vi "FP_Tracker.vi"() -> ()   [LabVIEW 2018, in "Tracker.lvlib"]
uses:
  Tracker.lvlib
  SubVi's/Controls/CTL_IO_status_indicator.ctl
  SubVi's/Controls/CTL_Zones_control_and_indicator.ctl
  SubVi's/Controls/CTL_Zone_indicator.ctl
  SubVi's/Controls/CTL_All_References.ctl
  SubVi's/Controls/CTL_Controls_References.ctl
  SubVi's/Controls/CTL_Indicators_References.ctl
  SubVi's/Controls/CTL_Panes_and_VIs_References.ctl
  SubVi's/Controls/CTL_Cage_radial_segmentation.ctl
  SubVi's/Controls/CTL_Image_Geometrical_and_scaling_parameters.ctl
  <vilib>/ProgressBar/Progress Bar Dialog.lvclass
  SubVi's/Controls/CTL_Calibration_parameters.ctl
  SubVi's/Controls/CTL_Dispenser_calibration_info.ctl
  SubVi's/Controls/CTL_Pre-filter_params.ctl
  SubVi's/Controls/CTL_Mouse_Draw_Params.ctl
  SubVi's/Controls/CTL_IO_params_cluster.ctl
  SubVi's/Controls/CTL_Overlays_cluster.ctl
  SubVi's/Controls/CTL_Animal_Coordinates_and_Speed.ctl
  SubVi's/Controls/CTL_Settings_cluster.ctl
  SubVi's/Controls/CTL_Histogram_parameters.ctl
  SubVi's/Controls/CTL_Filter_selector.ctl
  SubVi's/Controls/CTL_Acquisition_speed_selector.ctl
  SubVi's/Controls/CTL_Segmented_plot_parameters_2.ctl
  Libraries/Cage Diagram/Typedefs/CTL_Cage_type.ctl
  SubVi's/Controls/CTL_Cage_all_segmentation_params_set.ctl
  SubVi's/Controls/CTL_Conditions_Array.ctl
  SubVi's/Controls/CTL_Conditions_Cluster.ctl
  SubVi's/Controls/CTL_Condition_type.ctl
  SubVi's/Controls/CTL_Comparison_type.ctl
  SubVi's/Controls/CTL_Validity_check_criteria.ctl
  SubVi's/Controls/CTL_Response_info.ctl
  SubVi's/Controls/CTL_Condition_response_type.ctl
  SubVi's/Controls/CTL_Reponse_port_info.ctl
  SubVi's/Controls/CTL_Pixel_to_Zone_array.ctl
  SubVi's/Controls/CTL_Stats_parameters_(online).ctl
  SubVi's/Controls/CTL_Control_States.ctl
  SubVi's/Controls/CTL_States_cluster.ctl
  <vilib>/Platform/TimedLoop/XDataNode/timing_clust.ctl
  <vilib>/Platform/TimedLoop/XDataNode/nitl_modes.ctl
  <vilib>/Platform/TimedLoop/XDataNode/wakeup.ctl
  <vilib>/Utility/error.llb/DialogType.ctl
  SubVi's/Controls/CTL_Settings_parameters_groups.ctl
  Libraries/TTL IO/Typedefs/CTL_Parameter_transfer_name.ctl
  SubVi's/Controls/CTL_Post-processing_params.ctl
  <vilib>/vision/Image Controls.llb/IMAQ Image.ctl
  <vilib>/Utility/miscctls.llb/LVBoundsTypeDef.ctl
  SubVi's/Controls/CTL_Color_ramp.ctl
  <vilib>/Instr/_visa.llb/VISA Flush IO Buffer Mask.ctl
  SubVi's/Controls/CTL_Full_data_frame.ctl
  SubVi's/Controls/CTL_Measurements_and_Statistics.ctl
  <extravilib>/ChannelInstances/Stream-t'Tracker.lvlib-CTL_Full_data_frame.ctl'/Read With Abort.vi
  <extravilib>/ChannelInstances/Lossy Stream-t'Tracker.lvlib-CTL_Measurements_and_Statistics.ctl'/Write With Abort.vi
  <extravilib>/ChannelInstances/Lossy Stream-t'Tracker.lvlib-CTL_Animal_Coordinates_and_Speed.ctl'/Read With Abort.vi
  <extravilib>/ChannelInstances/Lossy Stream-a[.](dbl)/Read With Abort.vi
  <extravilib>/ChannelInstances/Lossy Stream-t'Tracker.lvlib-CTL_Measurements_and_Statistics.ctl'/Read With Abort.vi
  <extravilib>/ChannelInstances/Lossy Stream-a[.](dbl)/Write With Abort.vi
  <extravilib>/ChannelInstances/Lossy Stream-t'Tracker.lvlib-CTL_Animal_Coordinates_and_Speed.ctl'/Write With Abort.vi
  <extravilib>/ChannelInstances/Stream-t'Tracker.lvlib-CTL_Full_data_frame.ctl'/Write With Abort.vi
  <extravilib>/ChannelInstances/Stream-t'Tracker.lvlib-CTL_Full_data_frame.ctl'/EndpointRead.vi
  <extravilib>/ChannelInstances/Lossy Stream-t'Tracker.lvlib-CTL_Measurements_and_Statistics.ctl'/Endpoint.vi
  <extravilib>/ChannelInstances/Lossy Stream-t'Tracker.lvlib-CTL_Animal_Coordinates_and_Speed.ctl'/EndpointRead.vi
  <extravilib>/ChannelInstances/Lossy Stream-a[.](dbl)/EndpointRead.vi
  <extravilib>/ChannelInstances/Lossy Stream-t'Tracker.lvlib-CTL_Measurements_and_Statistics.ctl'/EndpointRead.vi
  <extravilib>/ChannelInstances/Lossy Stream-a[.](dbl)/Endpoint.vi
  <extravilib>/ChannelInstances/Lossy Stream-t'Tracker.lvlib-CTL_Animal_Coordinates_and_Speed.ctl'/Endpoint.vi
  <extravilib>/ChannelInstances/Stream-t'Tracker.lvlib-CTL_Full_data_frame.ctl'/Endpoint.vi
  <extravilib>/ChannelInstances/Lossy Stream-t'Tracker.lvlib-CTL_Measurements_and_Statistics.ctl'/Instantiate.vi
  <extravilib>/ChannelInstances/Stream-t'Tracker.lvlib-CTL_Full_data_frame.ctl'/Instantiate.vi
  <extravilib>/ChannelInstances/Lossy Stream-t'Tracker.lvlib-CTL_Animal_Coordinates_and_Speed.ctl'/Instantiate.vi
  <extravilib>/ChannelInstances/Lossy Stream-a[.](dbl)/Instantiate.vi
  SubVi's/SW_Globals_2.2+.vi
  <vilib>/Platform/TimedLoop/scheduler/LVUserAPI/_suppVIs/Create_1kHz_TSource.vi
  <extravilib>/ChannelInstances/Stream-t'Tracker.lvlib-CTL_Full_data_frame.ctl'/)Channel.vi
  <resource>/ChannelSupport/_ChannelSupport/WaitIfNeeded.vi
  <extravilib>/ChannelInstances/Lossy Stream-t'Tracker.lvlib-CTL_Measurements_and_Statistics.ctl'/)Channel.vi
  <extravilib>/ChannelInstances/Lossy Stream-t'Tracker.lvlib-CTL_Animal_Coordinates_and_Speed.ctl'/)Channel.vi
  <extravilib>/ChannelInstances/Lossy Stream-a[.](dbl)/)Channel.vi
  <vilib>/nisyscfg/Close (Resources).vi
  <vilib>/nisyscfg/Close (System).vi
  <userlib>/_OpenG.lib/file/file.llb/Valid Path - Traditional__ogtk.vi
  <vilib>/Utility/file.llb/Write Delimited Spreadsheet (DBL).vi
  <userlib>/_OpenG.lib/file/file.llb/File Exists - Scalar__ogtk.vi
  <vilib>/Platform/TimedLoop/XDataNode/XDataNode.xnode
  <vilib>/Platform/TimedLoop/XDataNode/XDNodeRunTimeDep.lvlib
  Common_Resources.lvlib
  <vilib>/nisyscfg/nisyscfg.lvlib
  <resource>/objmgr/nicontrollersysapi.rc
  <vilib>/Utility/config.llb/NI_LVConfig.lvlib
  <resource>/objmgr/nisysapi.rc
  Device low-level comms.lvlib
  <vilib>/Analysis/NI_AALBase.lvlib
  <extravilib>/ChannelInstances/Lossy Stream-a[.](dbl).lvlib
  <extravilib>/ChannelInstances/Stream-t'Tracker.lvlib-CTL_Full_data_frame.ctl'.lvlib
  <extravilib>/ChannelInstances/Lossy Stream-t'Tracker.lvlib-CTL_Animal_Coordinates_and_Speed.ctl'.lvlib
  <extravilib>/ChannelInstances/Lossy Stream-t'Tracker.lvlib-CTL_Measurements_and_Statistics.ctl'.lvlib
  <vilib>/ptbypt/NI_PtbyPt.lvlib
  Libraries/Tracks Repair/Tracks Repair.lvlib
  Libraries/Stream Data/Stream Data.lvlib
  Libraries/TTL IO/TTL IO.lvlib
  Libraries/Cage Diagram/Cage Diagram.lvlib
panel:
  out "VISA resource name out":refnum<visa-resource-name>
  in  "Load custom? (F)":bool
  out "Settings path to load":path
  out "Loaded.TDMS.path":path
  out "Frame #":u32
  in  "Start over":bool
  out "Active speed chunk":dbl[](array[numeric])
  out "Active part of track":cluster{"Numeric":dbl, "Numeric":dbl}[](array[cluster])
  in  "Stats parameters (online)":T1={"Mouse drawing parameters"={"Trace length, samples"=0, "Rainbow track"=FALSE, "Rainbow track is speed"=FALSE, "Bright mouse lineout"=FALSE, "Colors array"=[], "Pixels per mm"=0.0}, "Size of the image (480x480)"={"Numeric Control"=480.0, "Numeric Control"=480.0}, "Array of the pixel to zone correspondences"=[], "Hist. bins array"=[], "Histogram parameters"={"max"=300.0, "min"=0.0, "# bins"=10, "threshold"=8.0, "thr. type"=enum."higher accepted"}}
  out "Hist. X axis":dbl[](array[numeric])
  out "Loaded.zones":i8[](array[numeric])
  out "Pixel to zone":T3
  out "Current zone":T5
  in  "Save settings":bool
  in  "Reset zones":bool
  in  "Reset stimuli":bool
  out "Array of conditions":T6 {"Specifier(s)"."Validity criteria(s)"."Validity value" min=0.0 step=0.1 format="%.2g"; "Specifier(s)"."Value" step=1.0 format="%#.2g"}
  out "Ready":bool=TRUE
  in  "Check HW connection":bool
  in  "Set IO config":bool
  in  "Cage radial segmentation":T14={"CENTER"={"Radius, mm CENTER"=30}, "MIDFIELD"={"Radius, mm MIDFIELD"=75, "N segments MIDFIELD"=2, "Starting angle MIDFIELD"=0}, "BORDER"={"N segments BORDER"=4, "Starting angle BORDER"=0}} caption="Radial segmentation" {"BORDER"."N segments BORDER" min=1 max=12; "MIDFIELD"."N segments MIDFIELD" max=8; "CENTER"."Radius, mm CENTER" min=5 step=1}
  in  "Diagram (generated)":T15(plugin-control)=refnum
  out "Act. frame time, s":dbl
  out "Settings cluster (local)":T16={"Defaults"={"Default User"=0.0, "VISA Resource Name "="", "Histogram parameters"={"max"=300.0, "min"=0.0, "# bins"=10, "threshold"=8.0, "thr. type"=enum."higher accepted"}}, "Recording and saving"={"Researcher name"="", "Name prefix"="", "Data post-processing"={"Filter type"=enum."Savitzky-Golay", "Length"=31, "Order"=3}, "Stop at"=0.0, "\"Stop at\" enabled"=FALSE, "Default save folder path"=path "", "Acquisition FPS"=enum."Max"}, "Geometry"={"Sensor board size"=enum."", "Bridge swap"=FALSE, "Twisted neck"=FALSE, "Bridge H. offset"=0.0, "Bridge V. offset"=0.0, "Magnets orientation"=0.0, "Cage type"=0, "Cage parameters"={"Round"=variant(i16 0), "Square"=variant(u16 0), "Donut-maze"=variant(u16 0), "T-maze"=variant(u8 0), "Sociability-maze"=variant(u8 0)}}, "IO parameters"={"IO general config."=0, "IO 1 configuration"=0, "IO 2 configuration"=0, "IO 3 configuration"=0, "IO 4 configuration"=0, "Activate ext. RS-232"=0, "IO inversion config."=0, "Sync capability"=1}, "Conditions presets array"=[{"Enabled"=FALSE, "Name"="", "Specifier(s)"=[], "Response"={"Response type"=enum."Air puff", "TTL port"=enum."Port 1", "TTL pulse length, ms"=0.0}, "Has been set"=FALSE}, {"Enabled"=FALSE, "Name"="", "Specifier(s)"=[], "Response"={"Response type"=enum."Air puff", "TTL port"=enum."Port 1", "TTL pulse length, ms"=0.0}, "Has been set"=FALSE}, {"Enabled"=FALSE, "Name"="", "Specifier(s)"=[], "Response"={"Response type"=enum."Air puff", "TTL port"=enum."Port 1", "TTL pulse length, ms"=0.0}, "Has been set"=FALSE}, {"Enabled"=FALSE, "Name"="", "Specifier(s)"=[], "Response"={"Response type"=enum."Air puff", "TTL port"=enum."Port 1", "TTL pulse length, ms"=0.0}, "Has been set"=FALSE}, {"Enabled"=FALSE, "Name"="", "Specifier(s)"=[], "Response"={"Response type"=enum."Air puff", "TTL port"=enum."Port 1", "TTL pulse length, ms"=0.0}, "Has been set"=FALSE}, {"Enabled"=FALSE, "Name"="", "Specifier(s)"=[], "Response"={"Response type"=enum."Air puff", "TTL port"=enum."Port 1", "TTL pulse length, ms"=0.0}, "Has been set"=FALSE}, {"Enabled"=FALSE, "Name"="", "Specifier(s)"=[], "Response"={"Response type"=enum."Air puff", "TTL port"=enum."Port 1", "TTL pulse length, ms"=0.0}, "Has been set"=FALSE}, {"Enabled"=FALSE, "Name"="", "Specifier(s)"=[], "Response"={"Response type"=enum."Air puff", "TTL port"=enum."Port 1", "TTL pulse length, ms"=0.0}, "Has been set"=FALSE}, {"Enabled"=FALSE, "Name"="", "Specifier(s)"=[], "Response"={"Response type"=enum."Air puff", "TTL port"=enum."Port 1", "TTL pulse length, ms"=0.0}, "Has been set"=FALSE}, {"Enabled"=FALSE, "Name"="", "Specifier(s)"=[], "Response"={"Response type"=enum."Air puff", "TTL port"=enum."Port 1", "TTL pulse length, ms"=0.0}, "Has been set"=FALSE}, {"Enabled"=FALSE, "Name"="", "Specifier(s)"=[], "Response"={"Response type"=enum."Air puff", "TTL port"=enum."Port 1", "TTL pulse length, ms"=0.0}, "Has been set"=FALSE}, {"Enabled"=FALSE, "Name"="", "Specifier(s)"=[], "Response"={"Response type"=enum."Air puff", "TTL port"=enum."Port 1", "TTL pulse length, ms"=0.0}, "Has been set"=FALSE}, {"Enabled"=FALSE, "Name"="", "Specifier(s)"=[], "Response"={"Response type"=enum."Air puff", "TTL port"=enum."Port 1", "TTL pulse length, ms"=0.0}, "Has been set"=FALSE}, {"Enabled"=FALSE, "Name"="", "Specifier(s)"=[], "Response"={"Response type"=enum."Air puff", "TTL port"=enum."Port 1", "TTL pulse length, ms"=0.0}, "Has been set"=FALSE}], "Calibration parameters"={"Timing calibration sw/hw"=1.0, "True FPS"=80.0, "True frame time, s"=80.0, "Disp. calibration info"=[]}, "Settings loaded OK"=FALSE} {"Calibration parameters"."True frame time, s" format="%.10g"; "Calibration parameters"."Disp. calibration info"."Speed, µl per ms" format="%.3g"; "Calibration parameters"."True FPS" format="%.10g"; "Calibration parameters"."Timing calibration sw/hw" format="%.10g"; "Conditions presets array"."Specifier(s)"."Validity criteria(s)"."Validity value" min=0.0 step=0.1 format="%.2g"; "Conditions presets array"."Specifier(s)"."Value" step=1.0 format="%#.2g"; "Recording and saving"."Data post-processing"."Order" min=3 max=11 step=2; "Recording and saving"."Data post-processing"."Length" min=5 max=301 step=2; "Geometry"."Cage type" items=["Round", "Square", "Donut-maze", "T-maze", "Sociability maze", ""]}
  out "Loaded.TTL IO and Key":string[][](array[string])
  out "Loaded.HW ts and Frame HW time":u32[][](array[numeric])
  out "Loaded.Properties":string[][](array[string])
  out "Current position":T25
  out "Update timeline index?":bool
  out "Cur. pos. slider index":i32
  out "Timeline absolute min&max indices":T26
  out "Timeline absolute min&max":cluster{"Tl. min":dbl, "TL. max":dbl}
  out "Timeline min&max indices":T26
  out "Loaded.timeline":dbl[](array[numeric])
  out "Loaded.speed":dbl[](array[numeric])
  out "Loaded.alpha":dbl[](array[numeric])
  out "Loaded.Y":dbl[](array[numeric])
  out "Loaded.X":dbl[](array[numeric])
  out "Timeline min&max":cluster{"Tl. min":dbl, "TL. max":dbl}
  in  "Reset buffers?":bool
  out "Overlays cluster":T27
  out "Track show state":u32
  out "Start time (HW)":u32
  out "TTL in time (HW)":u32
  out "Key_pressed":string caption="Key"
  out "TDMS ref.":refnum<k34>
  out "TTL in time (SW)":timestamp
  out "IO parameters":T22
  out "Start time (SW)":timestamp
  out "Mouse drawing parameters":T2
  out "Pre-filter params.":T28
  out "Sensor board size":string
  out "FPS status":i32=80
  out "Rainbow is speed":bool=TRUE
  out "Calibration parameters":T23={"Timing calibration sw/hw"=1.0, "True FPS"=80.0, "True frame time, s"=80.0, "Disp. calibration info"=[]} {"True frame time, s" format="%.10g"; "Disp. calibration info"."Speed, µl per ms" format="%.3g"; "True FPS" format="%.10g"; "Timing calibration sw/hw" format="%.10g"}
  in  "Calibration samples":i32=2000
  out "Calibration SW timings":dbl[](array[numeric])
  out "Calibration HW timings":u32[](array[numeric])
  out "Progress Bar Dialog":refnum<class "Progress Bar Dialog.lvclass">
  out "VISA Resources found":string[](array[string])
  out "CPU load":sgl(slide) scale=0.0..100.0
  in  "ROIs list":i32(listbox)
  out "ROIs":T29
  out "Rainbow track":bool=TRUE
  out "Colors array":u32[](array[colorbox])
  out "UI update period":i64=53
  out "Trace length, samples":u16(slide)=20 scale=0.0..2000.0
  out "Bright mouse lineout":bool
  out "Img geom and scaling":T30
  out "Ports IO config":bool[](array[boolean])
  out "SB size":u8
  out "VISA resource name":refnum<visa-resource-name>
  out "Cage size":string="Large" caption="Cage diameter"
  in  "Set/Rec and Analyse Tab":enum32{"Settings", "Recording and Analysis"}(tab)
  in  "Reward and stimulation":string(tree) caption="Reward and stimulation conditions"
  in  "Add Reward":bool=TRUE
  in  "Modify Reward":bool=TRUE
  in  "Remove Reward":bool=TRUE
  out "Active rules":T31
  out "Average speed, mm/s":dbl caption="Avg., mm/s" format="%05.1f"
  out "Run distance, m":dbl caption="Distance, m" format="%0.3f"
  in  "Speed threshold":dbl=8.0 caption="@ mm/s >" format="%05.1f"
  in  "Rainbow (speed)":bool caption="Spdcode"
  in  "Rainbow (time)":bool caption="Timecode"
  in  "Show magnets":bool=TRUE caption="Magnets"
  in  "Playback speed":u16(ring)=3 caption="Speed" items=["5"=24, "4"=30, "3"=40, "2"=60, "1"=120, "1/2"=240, "1/3"=360, "1/4"=480, "1/5"=600]
  in  "Show heatmap":bool caption="Heat map"
  in  "Show full track":bool caption="Full track"
  in  "Show zones":bool=TRUE caption="Zones"
  in  "Trace, s":u16(slide)=5 max=30 step=1 scale=0.0..30.0
  in  "Multiplyer of chart RX":u8(slide)=1 max=9 step=1 scale=0.0..9.0
  out "Running, perc. of time":dbl caption="Run time, %" format="%05.2f"
  out "Histograms":T32(graph) caption="Speed histogram"
  in  "Reset barplot":bool
  out "Mouse speed":waveform(dbl)(graph)
  out "Mouse speed, mm/s":dbl caption="Speed, mm/s" format="%05.1f"
  out "Timing Source":string
  in  "Panes references":T33
  in  "Indicators references":T34
  in  "Controls references":T35
  in  "All references":T36
  in  "Diagram (display)":T15(plugin-control)=refnum
  out "HW info":string
  out "Port":string="Large"
  in  "Timeline":T37(slide)={"Slider"=0.0, "Slider"=648.2670807453416, "Slider"=2749.5465838509317} scale=0.016953468322753906..7.738564968109131 scale format="%<%H:%M:%S>t"
  in  "Play/Pause":bool
  in  "Open File":bool
  out "Since track start":dbl format="%<%H:%M:%S%1u>t"
  out "Current Time":timestamp=timestamp(3680686800.229 s since 1904-01-01) format="%<%H:%M:%S %d.%m.%Y>T"
  in  "Record/Stop":bool
  in  "By Zone stim. setup":T38=enum."Zone 13"
  out "IO status indicator":T39
  in  "error in (no error)":errorcluster
  out "error out":errorcluster={"status"=TRUE, "code"=1, "source"="Dequeue Element in NI_LVConfig.lvlib:Read Value Without Comment.vi->NI_LVConfig.lvlib:Read Key (I32).vi->SW_Load_settings_to_main_tab.vi"}
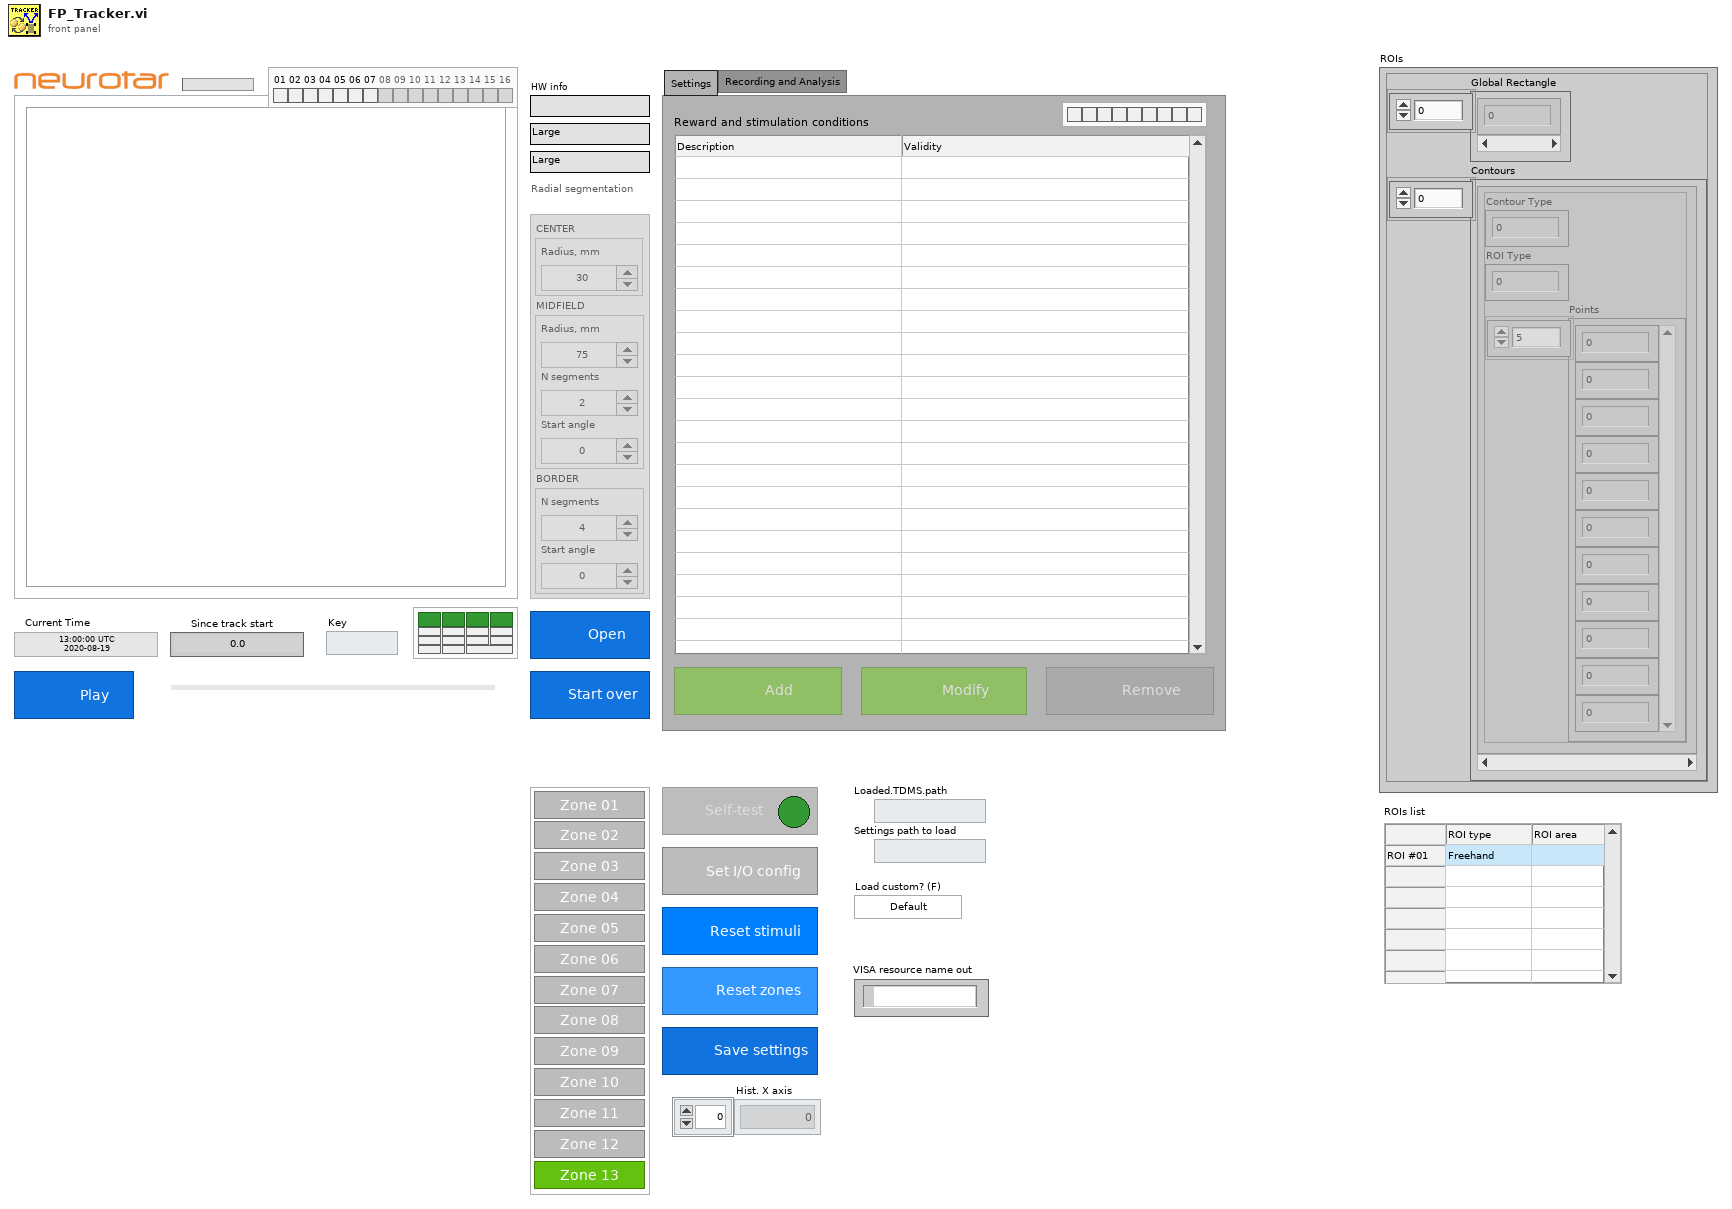
[diagram p1: front panel]
types:
  T1 = typedef "Common_Resources.lvlib/CTL_Stats_parameters_(online).ctl" = cluster{"Mouse drawing parameters":T2, "Size of the image (480x480)":cluster{"Numeric Control":dbl, "Numeric Control":dbl}, "Array of the pixel to zone correspondences":T3, "Hist. bins array":dbl[], "Histogram parameters":T4}
  T2 = typedef "Common_Resources.lvlib/CTL_Mouse_Draw_Params.ctl" = cluster{"Trace length, samples":u16, "Rainbow track":bool, "Rainbow track is speed":bool, "Bright mouse lineout":bool, "Colors array":u32[], "Pixels per mm":dbl}
  T3 = typedef "Common_Resources.lvlib/CTL_Pixel_to_Zone_array.ctl" = i8[][]
  T4 = typedef "Common_Resources.lvlib/CTL_Histogram_parameters.ctl" = cluster{"max":dbl, "min":dbl, "# bins":i32, "threshold":dbl, "thr. type":enum16{"higher accepted", "lower accepted"}}
  T5 = typedef "Common_Resources.lvlib/CTL_Zone_indicator.ctl" = cluster{"01":bool, "02":bool, "03":bool, "04":bool, "05":bool, "06":bool, "07":bool, "08":bool, "09":bool, "10":bool, "11":bool, "12":bool, "13":bool, "14":bool, "15":bool, "16":bool}
  T6 = typedef "Common_Resources.lvlib/CTL_Conditions_Array.ctl" = T7[]
  T7 = typedef "Common_Resources.lvlib/CTL_Conditions_Cluster.ctl" = cluster{"Enabled":bool, "Name":string, "Specifier(s)":cluster{"Specifier enabled":bool, "Condition type":T8, "Comparison type":T9, "Value":dbl, "Validity criteria(s)":cluster{"V. check enabled":bool, "Criteria":T10, "Validity value":dbl}[]}[], "Response":T11, "Has been set":bool}
  T8 = typedef "Common_Resources.lvlib/CTL_Condition_type.ctl" = enum16{"Speed", "Zone", "Angle to wall"}
  T9 = typedef "Common_Resources.lvlib/CTL_Comparison_type.ctl" = enum16{"Less", "Less or Equal", "Equal", "Greater or Equal", "Greater", "Not Equal"}
  T10 = typedef "Common_Resources.lvlib/CTL_Validity_check_criteria.ctl" = enum16{"Running bout (seconds)", "Running bout (meters)"}
  T11 = typedef "Common_Resources.lvlib/CTL_Response_info.ctl" = cluster{"Response type":T12, "TTL port":T13, "TTL pulse length, ms":dbl}
  T12 = typedef "Common_Resources.lvlib/CTL_Condition_response_type.ctl" = enum16{"None", "Air puff", "Liquid reward", "TTL pulse", "TTL pulse (ubr)", "TTL signal"}
  T13 = typedef "Common_Resources.lvlib/CTL_Reponse_port_info.ctl" = enum16{"Port 1", "Port 2", "Port 3", "Port 4"}
  T14 = typedef "Common_Resources.lvlib/CTL_Cage_radial_segmentation.ctl" = cluster{"CENTER":cluster{"Radius, mm CENTER":u16}, "MIDFIELD":cluster{"Radius, mm MIDFIELD":u16, "N segments MIDFIELD":u8, "Starting angle MIDFIELD":i16}, "BORDER":cluster{"N segments BORDER":u8, "Starting angle BORDER":i16}}
  T15 = typedef "IMAQ Image.ctl" = refnum<image>
  T16 = typedef "Common_Resources.lvlib/CTL_Settings_cluster.ctl" = cluster{"Defaults":cluster{"Default User":dbl, "VISA Resource Name ":string, "Histogram parameters":T4}, "Recording and saving":cluster{"Researcher name":string, "Name prefix":string, "Data post-processing":T17, "Stop at":dbl, "\"Stop at\" enabled":bool, "Default save folder path":path, "Acquisition FPS":T18}, "Geometry":T19, "IO parameters":T22, "Conditions presets array":T6, "Calibration parameters":T23, "Settings loaded OK":bool}
  T17 = typedef "Common_Resources.lvlib/CTL_Filter_selector.ctl" = cluster{"Filter type":enum16{"None", "Savitzky-Golay"}, "Length":i32, "Order":i32}
  T18 = typedef "Common_Resources.lvlib/CTL_Acquisition_speed_selector.ctl" = enum16{"Max", "Optimal", "Eco"}
  T19 = typedef "Common_Resources.lvlib/CTL_Segmented_plot_parameters_2.ctl" = cluster{"Sensor board size":enum16{"", "Large"}, "Bridge swap":bool, "Twisted neck":bool, "Bridge H. offset":sgl, "Bridge V. offset":sgl, "Magnets orientation":sgl, "Cage type":T20, "Cage parameters":T21}
  T20 = typedef "Cage Diagram.lvlib/CTL_Cage_type.ctl" = u16
  T21 = typedef "Common_Resources.lvlib/CTL_Cage_all_segmentation_params_set.ctl" = cluster{"Round":variant, "Square":variant, "Donut-maze":variant, "T-maze":variant, "Sociability-maze":variant}
  T22 = typedef "Common_Resources.lvlib/CTL_IO_params_cluster.ctl" = cluster{"IO general config.":u16, "IO 1 configuration":u16, "IO 2 configuration":u16, "IO 3 configuration":u16, "IO 4 configuration":u16, "Activate ext. RS-232":u16, "IO inversion config.":u16, "Sync capability":u8}
  T23 = typedef "Common_Resources.lvlib/CTL_Calibration_parameters.ctl" = cluster{"Timing calibration sw/hw":dbl, "True FPS":dbl, "True frame time, s":dbl, "Disp. calibration info":T24}
  T24 = typedef "Common_Resources.lvlib/CTL_Dispenser_calibration_info.ctl" = cluster{"Channel":u8, "Speed, µl per ms":dbl}[]
  T25 = typedef "Common_Resources.lvlib/CTL_Animal_Coordinates_and_Speed.ctl" = cluster{"R from center":dbl, "phi (mouse angular position in the cage)":dbl, "alpha (mouse rot. angle)":dbl, "X":dbl, "Y":dbl, "theta (from center towards mouse)":dbl, "beta (cage rot. against mouse)":dbl, "w (mouse angle to wall)":dbl, "Speed (filtered)":dbl}
  T26 = cluster{"Tl. min index":i32, "Tl. max index":i32}
  T27 = typedef "Common_Resources.lvlib/CTL_Overlays_cluster.ctl" = cluster{"Time-coded track overlay (array)":u32[][], "Speed-coded track overlay (array)":u32[][], "Plain track overlay pixmap":u32[][], "Location density map image":u32[][], "Speed density map image":u32[][], "Location density map":dbl[][], "Speed density map":dbl[][]}
  T28 = typedef "Common_Resources.lvlib/CTL_Pre-filter_params.ctl" = cluster{"Reverse coefficients":dbl[], "Forward coefficients":dbl[], "Full filter length (info only)":i32, "Type":enum16{"None", "FIR (PtbyPt)", "IIR (PtbyPt)"}}
  T29 = cluster{"Global Rectangle":i32[], "Contours":cluster{"Contour Type":u32, "ROI Type":u32, "Points":i32[]}[]}
  T30 = typedef "Common_Resources.lvlib/CTL_Image_Geometrical_and_scaling_parameters.ctl" = cluster{"Fonts scale factor":dbl, "Pixels per mm":dbl, "Radius of displayed outer segments, pix":dbl, "Radius of displayed midfield segments, pix":dbl, "Radius of displayed central segment, pix":dbl}
  T31 = cluster{"01":bool, "02":bool, "03":bool, "04":bool, "05":bool, "06":bool, "07":bool, "08":bool, "09":bool}
  T32 = cluster{"X Values":dbl[], "Histogram: h(x)":dbl[]}
  T33 = typedef "Common_Resources.lvlib/CTL_Panes_and_VIs_References.ctl" = cluster{"Pane":refnum<vi>, "This VI":refnum<vi>, "Menu":refnum<k9>}
  T34 = typedef "Common_Resources.lvlib/CTL_Indicators_References.ctl" = cluster{"HW info":refnum<vi>, "Port":refnum<vi>, "Ready":refnum<vi>, "IO status indicator":refnum<vi>, "Current Time":refnum<vi>, "Record timestamp":refnum<vi>, "Mouse speed":refnum<vi>, "Mouse speed, mm/s":refnum<vi>, "Running, perc. of time":refnum<vi>, "Histograms":refnum<vi>, "Cage size":refnum<vi>, "Reward":refnum<vi>, "Current zone":refnum<vi>, "Run length, m":refnum<vi>}
  T35 = typedef "Common_Resources.lvlib/CTL_Controls_References.ctl" = cluster{"Check HW connection":refnum<vi>, "Save settings":refnum<vi>, "Reset zones":refnum<vi>, "Reset stimuli":refnum<vi>, "Record/Stop":refnum<vi>, "Reset barplot":refnum<vi>, "Multiplyer of chart RX":refnum<vi>, "Show zones":refnum<vi>, "Show magnets":refnum<vi>, "Show heatmap":refnum<vi>, "Show full track":refnum<vi>, "Open File":refnum<vi>, "Play/Pause":refnum<vi>, "Trace, s":refnum<vi>, "Playback speed":refnum<vi>, "Timeline":refnum<vi>, "By Zone stim. setup":refnum<vi>, "Set/Rec and Analyse Tab":refnum<vi>, "Cage radial segmentation":refnum<vi>, "Set IO config":refnum<vi>, "Rainbow (time)":refnum<vi>, "Rainbow (speed)":refnum<vi>, "Add Reward":refnum<vi>, "Modify Reward":refnum<vi>, "Delete Reward":refnum<vi>, "Speed threshold, mm/s":refnum<vi>, "Start Over":refnum<vi>}
  T36 = typedef "Common_Resources.lvlib/CTL_All_References.ctl" = cluster{"Controls references":T35, "Indicators references":T34, "Service references":T33}
  T37 = cluster{"Slider":dbl, "Slider":dbl, "Slider":dbl}
  T38 = typedef "Common_Resources.lvlib/CTL_Zones_control_and_indicator.ctl" = enum32{"No Selection", "Zone 01", "Zone 02", "Zone 03", "Zone 04", "Zone 05", "Zone 06", "Zone 07", "Zone 08", "Zone 09", "Zone 10", "Zone 11", "Zone 12", "Zone 13"}
  T39 = typedef "Common_Resources.lvlib/CTL_IO_status_indicator.ctl" = cluster{"IO1":bool, "IO2":bool, "IO3":bool, "IO4":bool, "St1":bool, "St2":bool, "St3":bool, "St4":bool, "Z1":bool, "Z2":bool, "Z3":bool, "Z4":bool, "Syn1":bool, "Syn2":bool, "RS-232 ext. activated":bool}
  T40 = cluster{"[0]":bool, "[1]":bool, "[2]":bool, "[3]":bool, "[4]":bool, "[5]":bool, "[6]":bool, "[7]":bool, "[8]":bool}
  T41 = cluster{"Boolean Round":bool, "code":i32, "source":string}
  T42 = typedef "Tracks Repair.lvlib/Broadcast Events--cluster.ctl" = cluster{"Module Did Init":refnum<user-event>, "Status Updated":refnum<user-event>, "Error Reported":refnum<user-event>, "Module Did Stop":refnum<user-event>, "Update Module Execution Status":refnum<user-event>}
  T43 = typedef "Stream Data.lvlib/Broadcast Events--cluster.ctl" = cluster{"Module Did Init":refnum<user-event>, "Status Updated":refnum<user-event>, "Error Reported":refnum<user-event>, "Module Did Stop":refnum<user-event>, "Update Module Execution Status":refnum<user-event>}
  T44 = typedef "TTL IO.lvlib/Broadcast Events--cluster.ctl" = cluster{"Module Did Init":refnum<user-event>, "Status Updated":refnum<user-event>, "Error Reported":refnum<user-event>, "Module Did Stop":refnum<user-event>, "Update Module Execution Status":refnum<user-event>, "Conditions that are TRUE (active rules)":refnum<user-event>}
  T45 = typedef "Cage Diagram.lvlib/Broadcast Events--cluster.ctl" = cluster{"Module Did Init":refnum<user-event>, "Status Updated":refnum<user-event>, "Error Reported":refnum<user-event>, "Module Did Stop":refnum<user-event>, "Update Module Execution Status":refnum<user-event>, "Broadcast New Layout":refnum<user-event>}
  T46 = typedef "Common_Resources.lvlib/CTL_States_cluster.ctl" = cluster{"Acq. is ON":bool, "Playing loaded":bool, "Recording now":bool, "Has been recorded":bool, "Data saved":bool, "Data loaded":bool, "Calibration mode":bool, "Offline mode":bool, "Stop and Exit":bool, "Updating layout":bool}
  T47 = typedef "Common_Resources.lvlib/CTL_Control_States.ctl" = enum16{"SW Init", "HW Init", "Close App", "Update port info (Init OK)", "Unlock UI (init OK)", "Save HW Settings", "Re-check HW (init failed)", "Configure port(s)", "Switch to Offline mode", "Switch to Online mode", "Zones layout update", "Set I/O config (silent)", "Set I/O config", "Play Start", "Play Stop", "Upd. FPS", "Upd. trace length", "Cage and recording settings", "Update filter", "Timings calibration start", "Timings calibration finish", "Dispension calibration", "Save all settings to custom location", "Save all settings", "Start Recording", "Stop Recording", "Recording post-processing", "Timeline update", "Overlay tracks update", "Load custom settings", "Load recorded data", "Save density map(s)", "Process loaded settings", "Prepare loaded data playback", "Add Reward condition", "Modify Reward condition", "Delete Reward condition", "Check Reward condition(s)", "Location map update", "Speed map update", "Start over", "Default (test)", "IDL Error", "Recalculate track with new settings"}
  T48 = typedef "XDNodeRunTimeDep.lvlib/timing_clust.ctl" = cluster{"Expected End [f-1]":u64, "Actual End [f-1]":u64, "Finished Late? [f-1]":bool, "Expected End [i-1]":u64, "Actual End [i-1]":u64, "Finished Late? [i-1]":bool, "Expected Start [i]":u64, "Actual Start [i]":u64, "Expected Start [f]":u64, "Actual Start [f]":u64, "Source Name":string, "Structure Name":string, "Period":i64, "Deadline":i64, "Offset":i64, "Start":i64, "Priority":i32, "Timeout":i32, "Mode":T49, "Wakeup Reason":T50, "Error":errorcluster, "Source Type":string, "Secondary Source Type":string, "Global End Time":u64, "Global Start Time":u64, "Frame Duration":u64, "Iteration Duration":u64, "Assigned CPU":i32, "I/O Scan Engine Mode":u32}
  T49 = typedef "XDNodeRunTimeDep.lvlib/nitl_modes.ctl" = enum32{"No Change", "Process missed periods, maintain original phase", "Discard missed periods, maintain original phase", "Process missed periods, ignore original phase", "Discard missed periods, ignore original phase"}
  T50 = typedef "XDNodeRunTimeDep.lvlib/wakeup.ctl" = enum32{"Normal", "Aborted", "Asynchronous wakeup", "Timing source error", "Timed loop error", "Timeout"}
  T51 = typedef "Common_Resources.lvlib/CTL_Full_data_frame.ctl" = cluster{"Times":cluster{"ms since ON":u32, "delta time":u32, "Frame timestamp":timestamp}, "TTLs":cluster{"TTL input":i16, "TTL output":i16}, "Animal coordinates":T25, "Magnets coords raw":cluster{"X1 raw":dbl, "Y1 raw":dbl, "X2 raw":dbl, "Y2 raw":dbl}, "Measurements and statistics":T52}
  T52 = typedef "Common_Resources.lvlib/CTL_Measurements_and_Statistics.ctl" = cluster{"Zone #":i8, "Histogram":dbl[], "Running, perc. of time":dbl, "Run, meters":dbl, "Avg. speed":dbl}
  T53 = typedef "Lossy Stream-a[.](dbl).lvlib/)Channel.ctl" = refnum<queue>
  T54 = typedef "Common_Resources.lvlib/CTL_Decoded_data_frame.ctl" = cluster{"ms since ON":u32, "delta time":u32, "X1":sgl, "Y1":sgl, "X2":sgl, "Y2":sgl, "TTL input":i16, "TTL output":i16, "Frame timestamp":timestamp, "Frame OK":bool}
  T55 = cluster{"X1 raw":dbl, "Y1 raw":dbl, "X2 raw":dbl, "Y2 raw":dbl}
  T56 = cluster{"ms since ON":u32, "delta time":u32, "Frame timestamp":timestamp}
  T57 = typedef "Common_Resources.lvlib/CTL_Cage_Coords.ctl" = cluster{"R from center":dbl, "sin(a)":dbl, "Mouse Xc":dbl, "Mouse Yc":dbl, "X1-X2":dbl, "Y1-Y2":dbl, "Cage Xc":dbl, "Cage Yc":dbl, "Frame time, s":dbl}
  T58 = typedef "Lossy Stream-t'Tracker.lvlib-CTL_Animal_Coordinates_and_Speed.ctl'.lvlib/)Channel.ctl" = refnum<queue>
  T59 = typedef "Stream-t'Tracker.lvlib-CTL_Full_data_frame.ctl'.lvlib/)Channel.ctl" = refnum<queue>
  T60 = cluster{"Numeric Control":u32, "Numeric Control":u32}[]
  T61 = typedef "Common_Resources.lvlib/CTL_Settings_parameters_groups.ctl" = string
  T62 = enum32{"Page Enabled", "Page Disabled", "Page Disabled & Grayed"}
  T63 = enum8{"Enabled", "Disabled", "Disabled and Grayed Out"}
  T64 = typedef "TTL IO.lvlib/CTL_Parameter_transfer_name.ctl" = enum16{"None", "All parameters", "IO parameters", "Conditions"}
  T65 = typedef "Common_Resources.lvlib/CTL_Post-processing_params.ctl" = cluster{"Defragment TDMS? (F)":bool, "Start time (SW)":timestamp, "Start time (HW)":u32, "Data filtering":T17, "Mouse drawing parameters":T2, "Size of the image (480x480)":cluster{"X size":dbl, "Y size":dbl}, "Image ref. in":T15, "Calibration parameters":T23, "Pixel to zone":T3}
  T66 = cluster{"TL. min index":i32, "TL. max index":i32}
  T67 = typedef "LVBoundsTypeDef.ctl" = cluster{"Width":u32, "Height":u32}
  T68 = typedef "DialogType.ctl" = u16
  T69 = cluster{"Previous step":T47, "error IO":errorcluster}
  T70 = enum32{"invalid app kind", "Development System", "Run Time System", "Student Edition", "Embedded LabVIEW", "Evaluation", "Custom"}
  T71 = typedef "Cage Diagram.lvlib/New Layout (instant) (Reply Payload)--cluster.ctl" = cluster{"Cage Diagram ref":T15, "Pixel <> Zone":T3, "Cage drawing parameters out":T72, "New Layout (instant)_error":errorcluster}
  T72 = typedef "Cage Diagram.lvlib/CTL_Cage_drawing_params.ctl" = cluster{"Draw Area Size":T73, "Cage External Dims.":T74, "Background color":u32, "Image Scaling info":T75, "Segments Colors":T76}
  T73 = typedef "Common_Resources.lvlib/CTL_Draw_Area_Size.ctl" = cluster{"Width, pix":i32, "Height, pix":i32}
  T74 = typedef "Cage Diagram.lvlib/CTL_Cage_External_dimensions.ctl" = cluster{"Width, mm":dbl, "Height, mm":dbl}
  T75 = typedef "Cage Diagram.lvlib/CTL_Image_Scaling_info.ctl" = cluster{"Fonts scale factor":dbl, "Pixels per mm":dbl}
  T76 = typedef "Common_Resources.lvlib/CTL_Segments_Colors_(pie).ctl" = cluster{"Colors array for outer segments":u32[], "Colors array for midfield segments":u32[], "Color for central segment":u32, "Fill color for no segments image":u32}
  T77 = typedef "Common_Resources.lvlib/CTL_Paths_cluster.ctl" = cluster{"Program settings":path, "Folder":path, "TDMS file reference":refnum<k34>, "TDMS track":path, "Track settings":path, "Layout picture":path, "Density map matrix (time)":path, "Density map picture (time)":path, "Density map matrix (speed)":path, "Density map picture (speed)":path, "ZIP":path}
  T78 = typedef "NI_LVConfig.lvlib/Config Data RefNum.ctl" = refnum<k1>
  T79 = enum16{"Left Button", "Center Button", "Right Button", "Window Close"}
  T80 = cluster{"Geometry out":T19, "Value":bool, "Value":bool}
  T81 = cluster{"Slider 1":dbl, "Slider 2":dbl, "Slider 3":dbl}
  T82 = cluster{"Numeric Control":dbl, "Numeric Control":dbl}
  T83 = typedef "Common_Resources.lvlib/CTL_Loaded_data_output_(offline).ctl" = cluster{"HW ts and Frame HW time":u32[][], "SW timestamp":dbl[], "TTL IO and Key":string[][], "Track properties":string[][], "Coords data":dbl[][], "Zone":i8[]}
  T84 = typedef "Cage Diagram.lvlib/Get Layout Image as Array (Reply Payload)--cluster.ctl" = cluster{"Layout image array (U32)":u32[][], "Get Layout Image as Array_error":errorcluster}
  T85 = typedef "imagedata.ctl" = cluster{"image type":i32, "image depth":i32, "image":u8[], "mask":u8[], "colors":u32[], "Rectangle":cluster{"left":i16, "top":i16, "right":i16, "bottom":i16}}
  T86 = typedef "Common_Resources.lvlib/CTL_Color_ramp.ctl" = u32[]
  T87 = typedef "LVNodeAndColumnTypeDef.ctl" = cluster{"Node":string, "Column":i32}
  T88 = typedef "VISA Flush IO Buffer Mask.ctl" = u16
  T89 = typedef "Tracker.lvlib/CTL_States_cluster.ctl" = cluster{"Acq. is ON":bool, "Playing loaded":bool, "Recording now":bool, "Has been recorded":bool, "Data saved":bool, "Data loaded":bool, "Calibration mode":bool, "Offline mode":bool, "Stop and Exit":bool, "Updating layout":bool}
  T90 = typedef "Lossy Stream-t'Tracker.lvlib-CTL_Measurements_and_Statistics.ctl'.lvlib/)Channel.ctl" = refnum<queue>
  T91 = cluster{"Tl. min":dbl, "TL. max":dbl, "Numeric":dbl}
  T92 = cluster{"array[0]":bool, "array[1]":bool, "array[2]":bool, "array[3]":bool, "array[4]":bool, "array[5]":bool, "array[6]":bool, "array[7]":bool, "array[8]":bool, "array[9]":bool, "array[10]":bool, "array[11]":bool, "array[12]":bool, "array[13]":bool, "array[14]":bool, "array[15]":bool}
  T93 = cluster{"Contour Type":u32, "ROI Type":u32, "Points":i32[]}[]
  T94 = cluster{"Active rules[0]":bool, "Active rules[1]":bool, "Active rules[2]":bool, "Active rules[3]":bool, "Active rules[4]":bool, "Active rules[5]":bool, "Active rules[6]":bool, "Active rules[7]":bool, "Active rules[8]":bool}
  T95 = typedef "eventvkey.ctl" = enum16{"ASCII", "Enter", "Return", "Shift", "Ctrl", "Alt", "Cmd", "Opt", "Caps", "NumLock", "Clear", "Break", "Up", "Down", "Left", "Right", "Insert", "Delete", "Home", "End", "PageUp", "PageDown", "Escape", "Help", "Pause", "ScrollLock", "F1", "F2", "F3", "F4", "F5", "F6", "F7", "F8", "F9", "F10", "F11", "F12", "F13", "F14", "F15", "F16", "F17", "F18", "F19", "F20", "F21", "F22", "F23", "F24", "Play", "VolumeUp", "VolumeDown", "Mute", "Two Byte Char"}
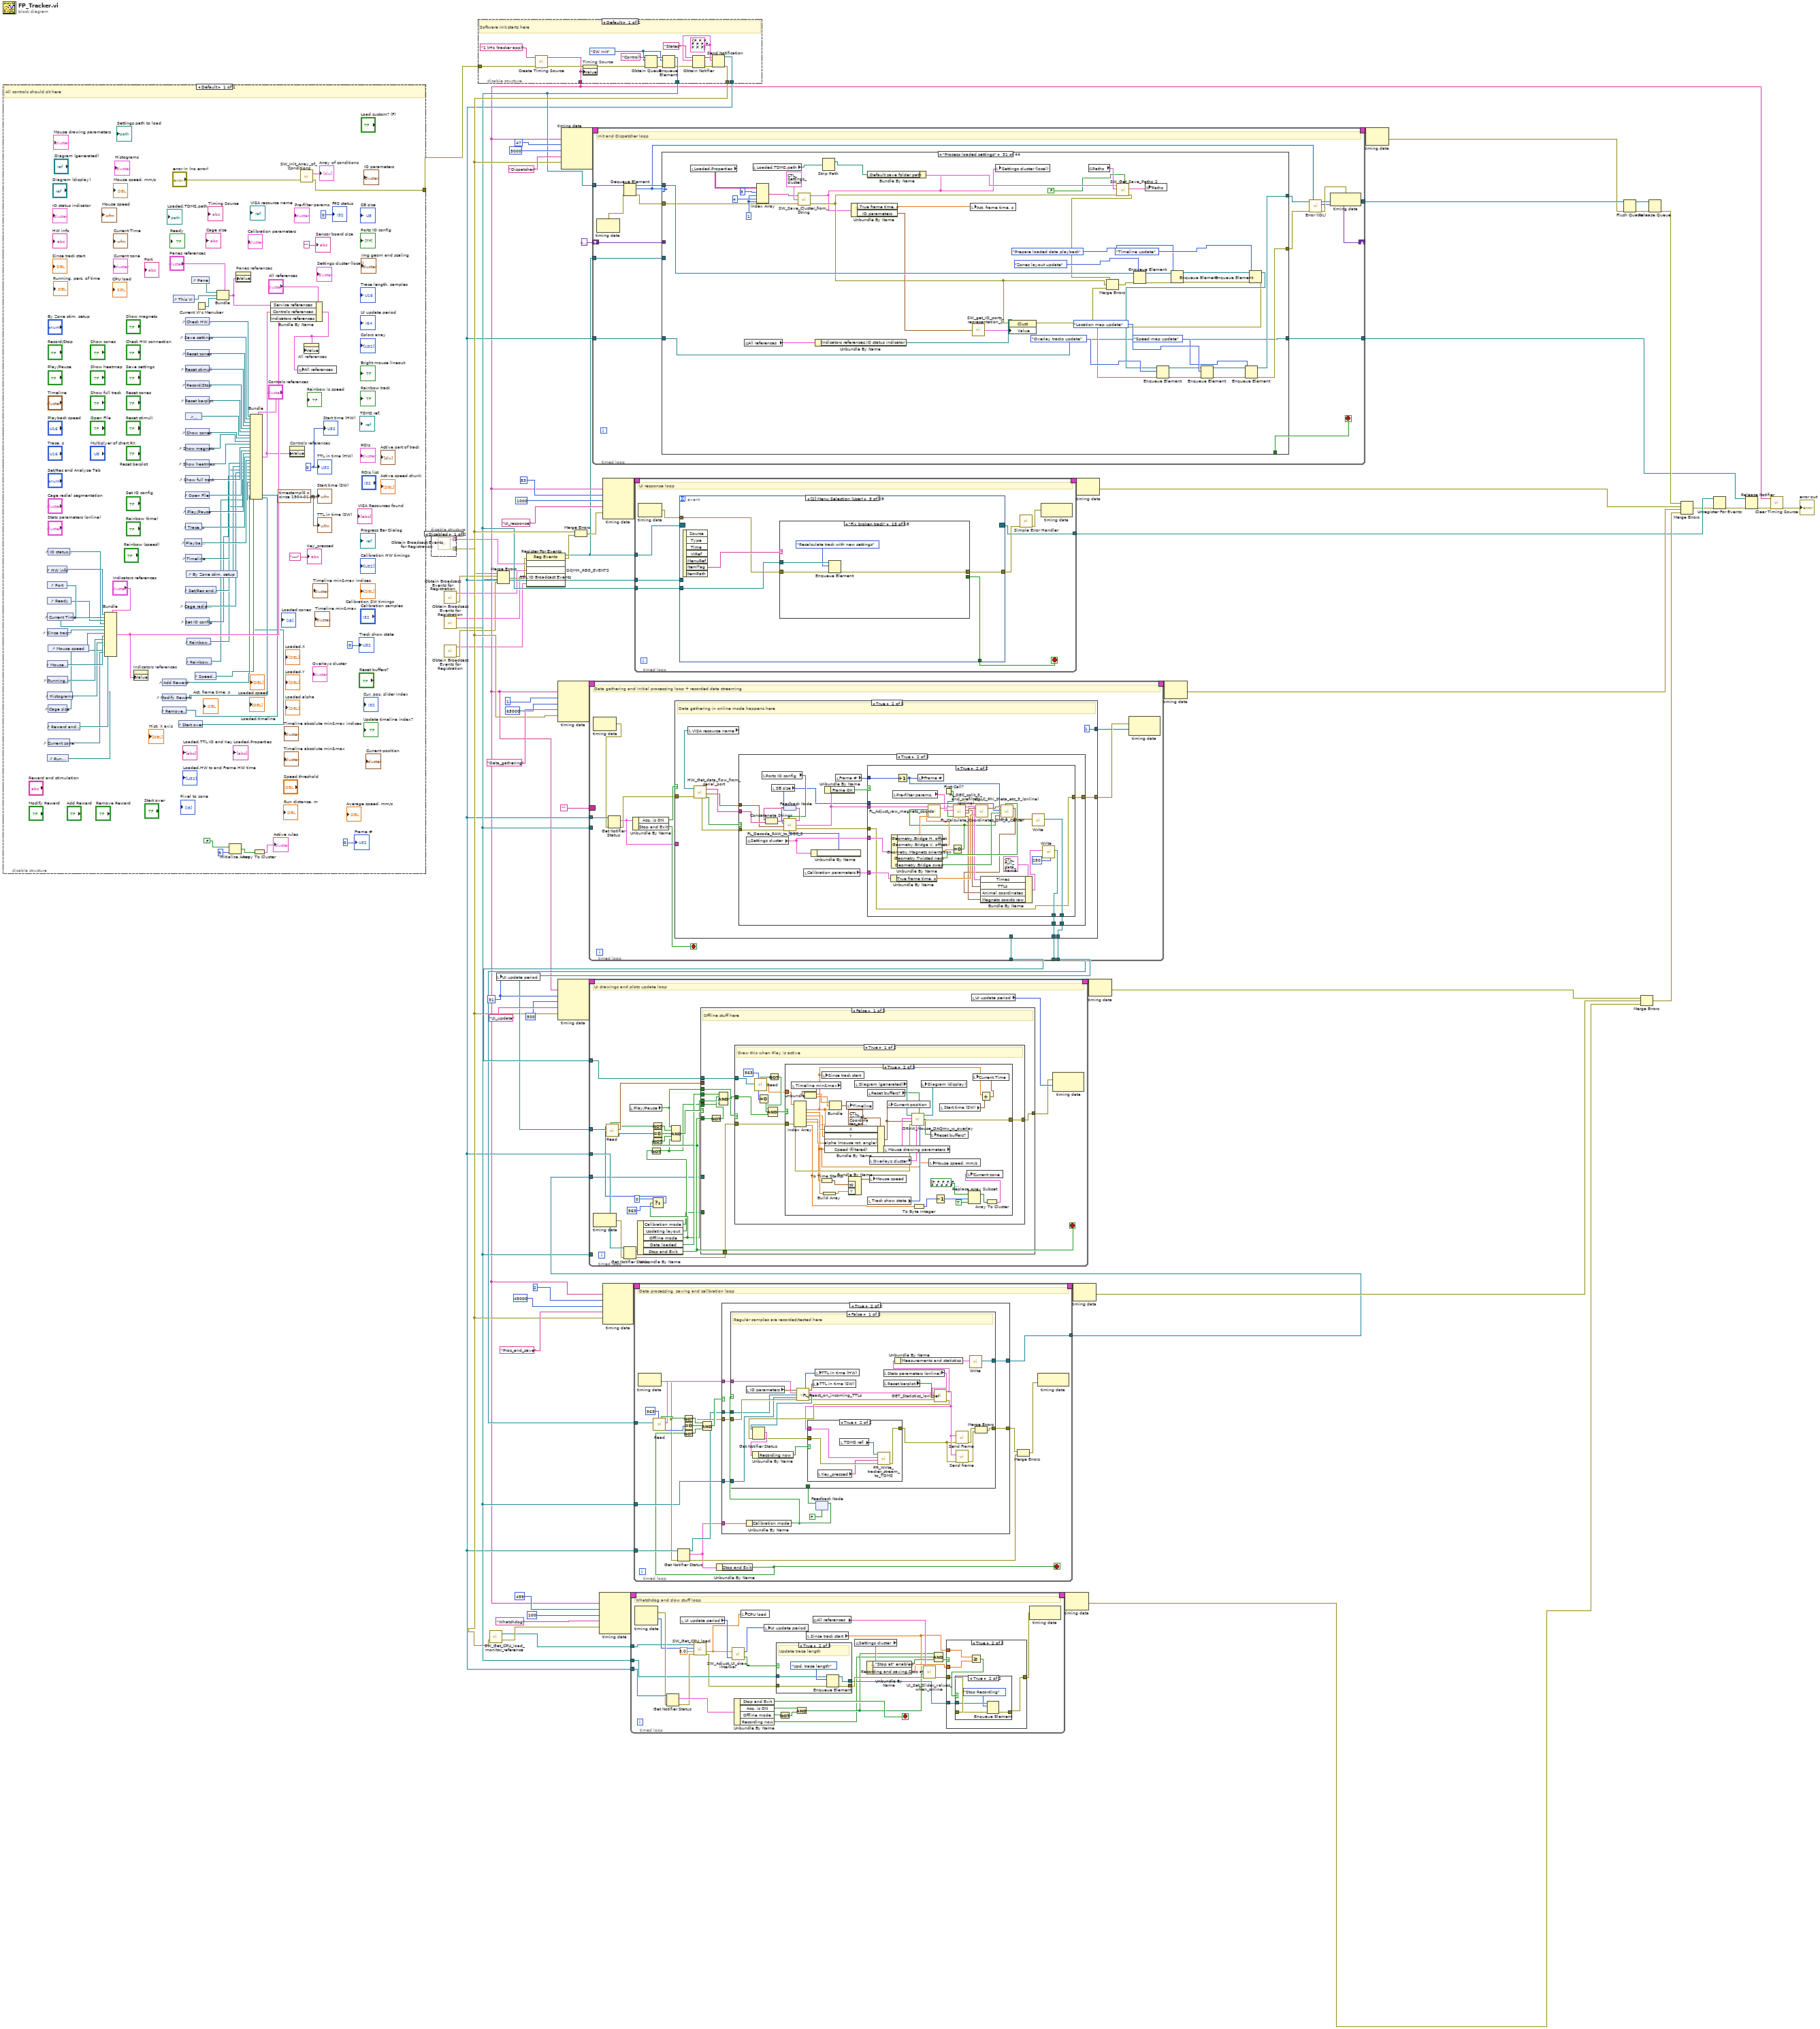
[diagram p0: block diagram]
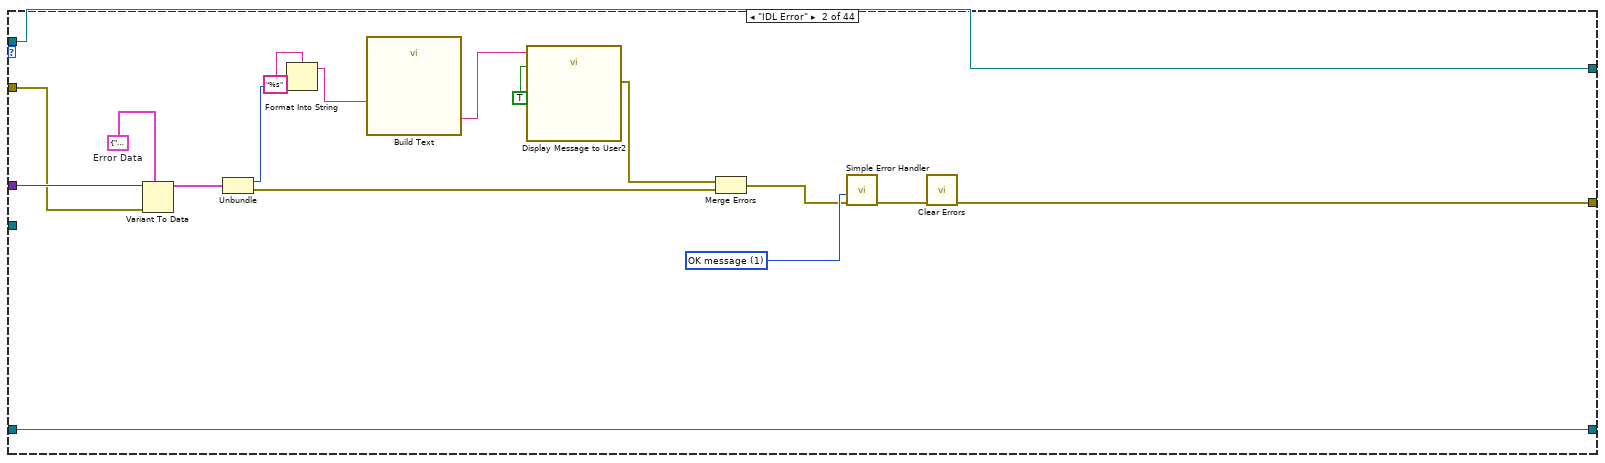
[diagram p4: hidden frame]
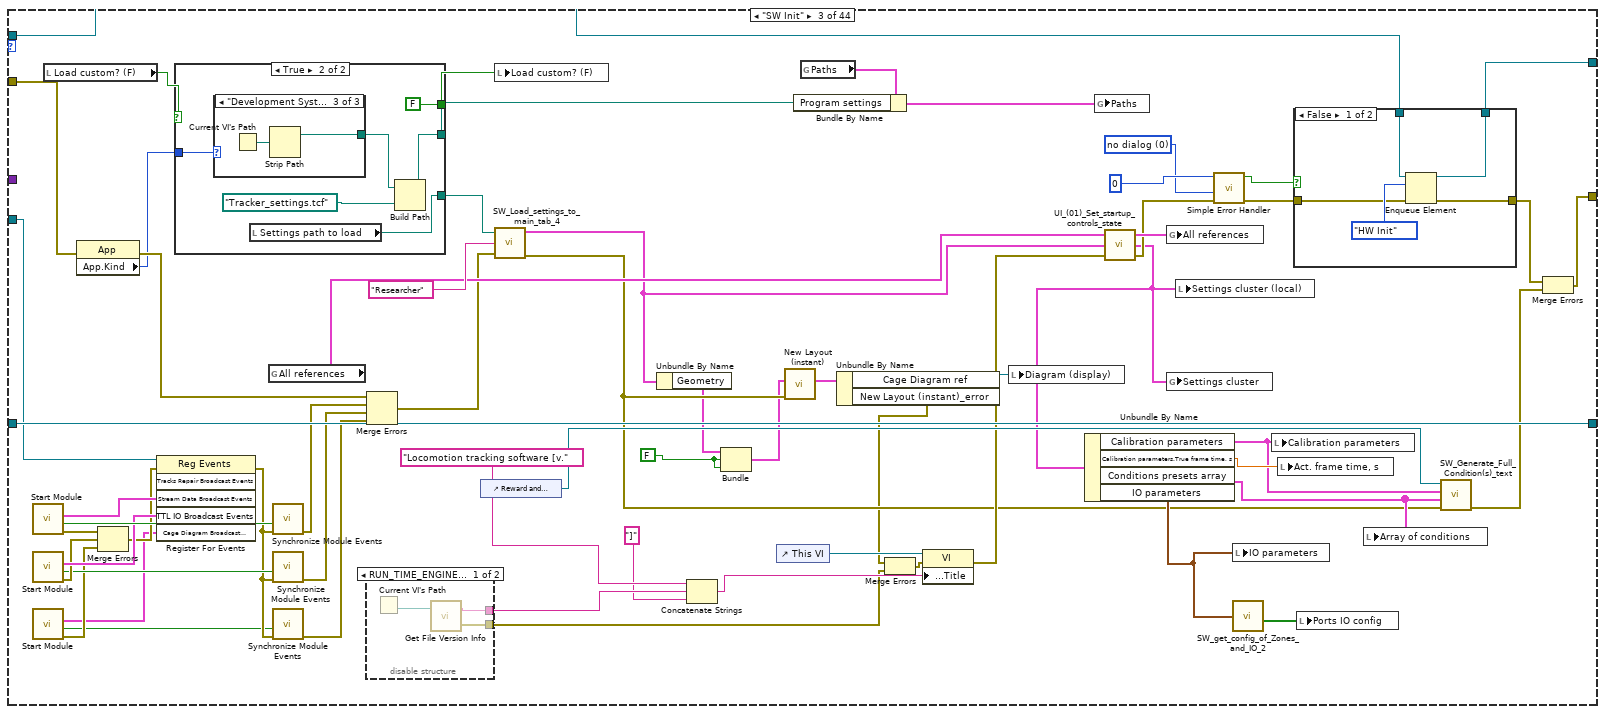
[diagram p5: hidden frame]
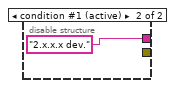
[diagram p6: hidden frame]
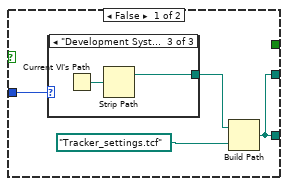
[diagram p7: hidden frame]
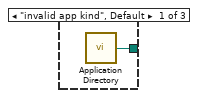
[diagram p8: hidden frame]
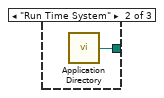
[diagram p9: hidden frame]
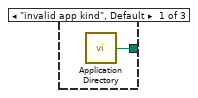
[diagram p10: hidden frame]
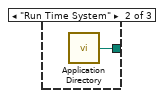
[diagram p11: hidden frame]
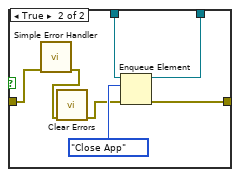
[diagram p12: hidden frame]
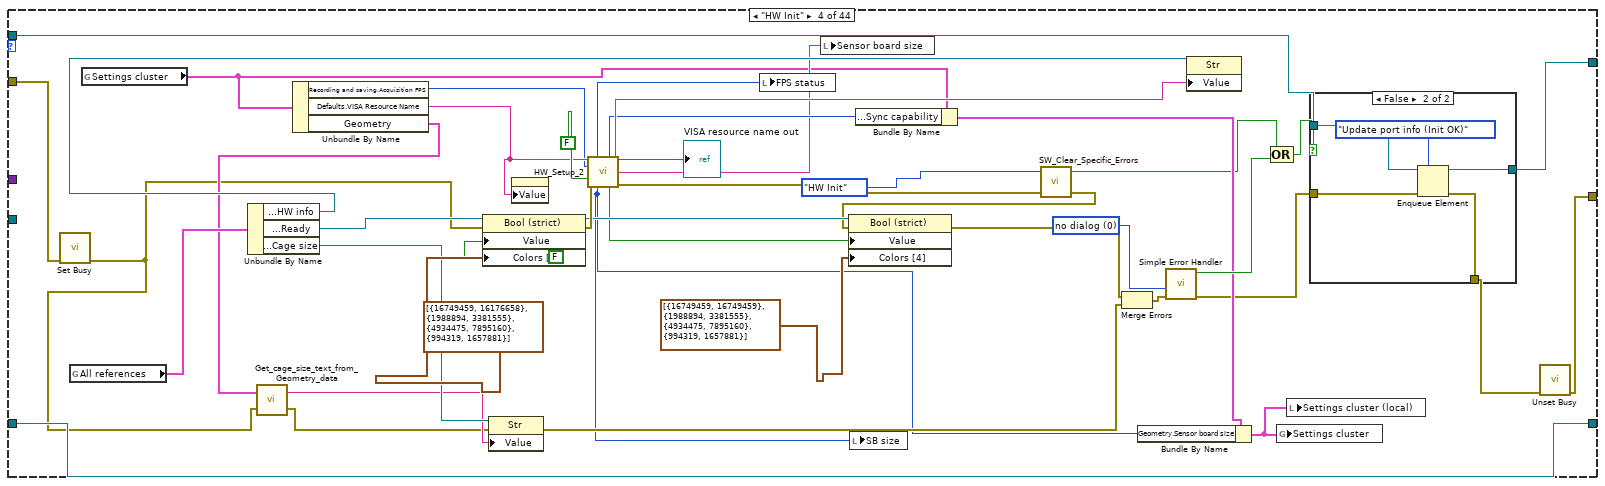
[diagram p13: hidden frame]
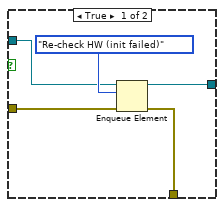
[diagram p14: hidden frame]
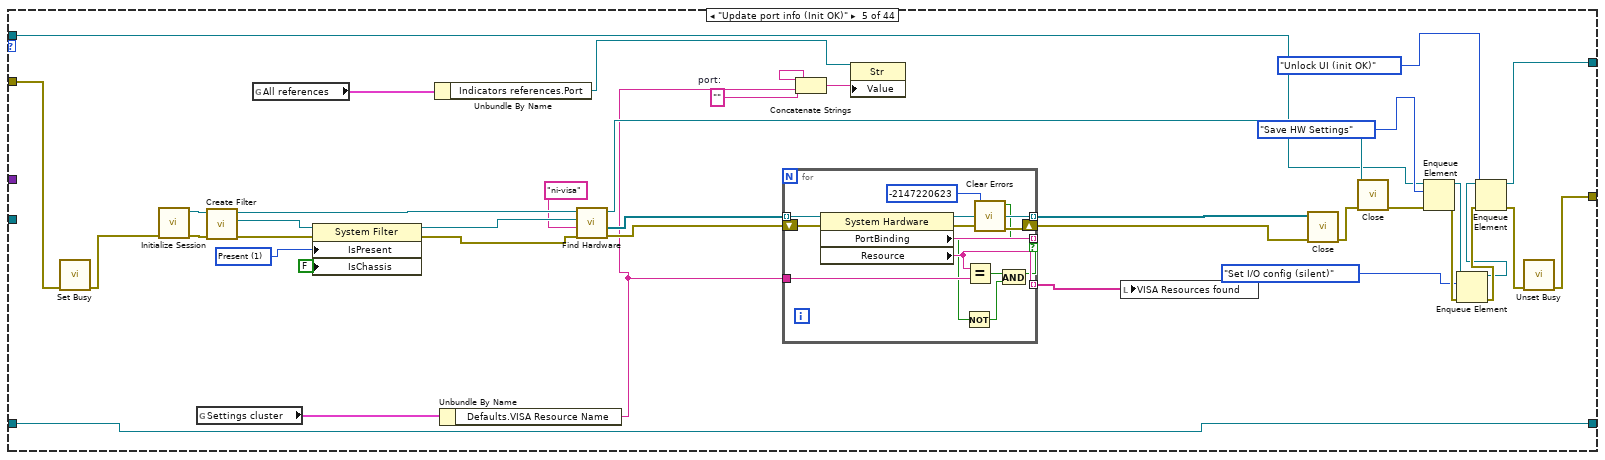
[diagram p15: hidden frame]
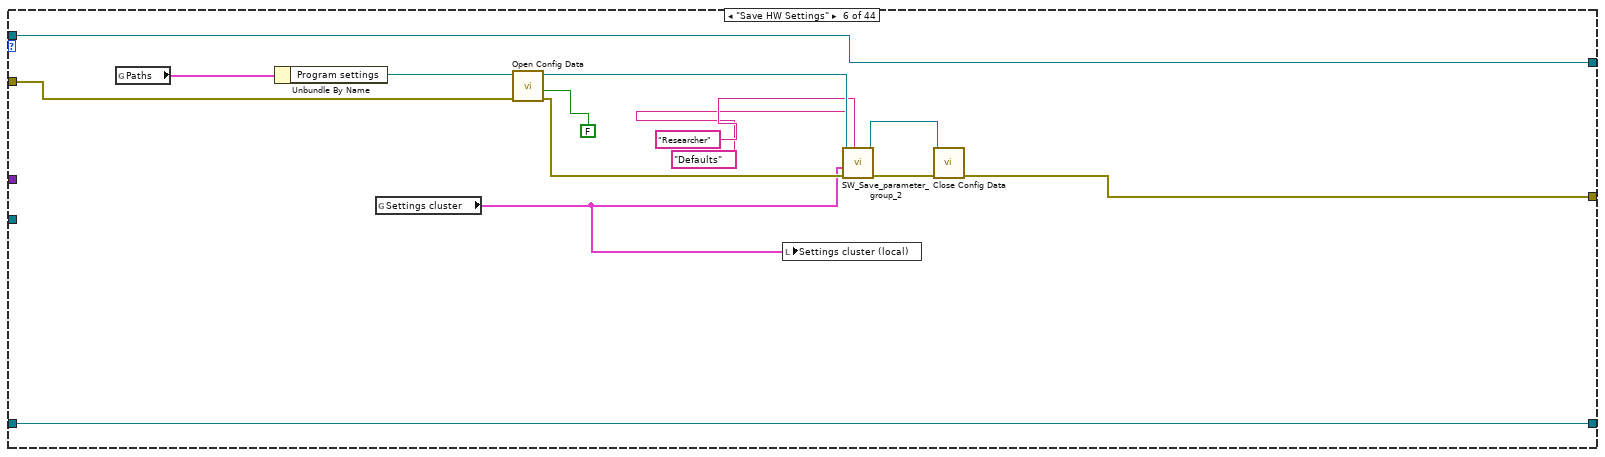
[diagram p16: hidden frame]
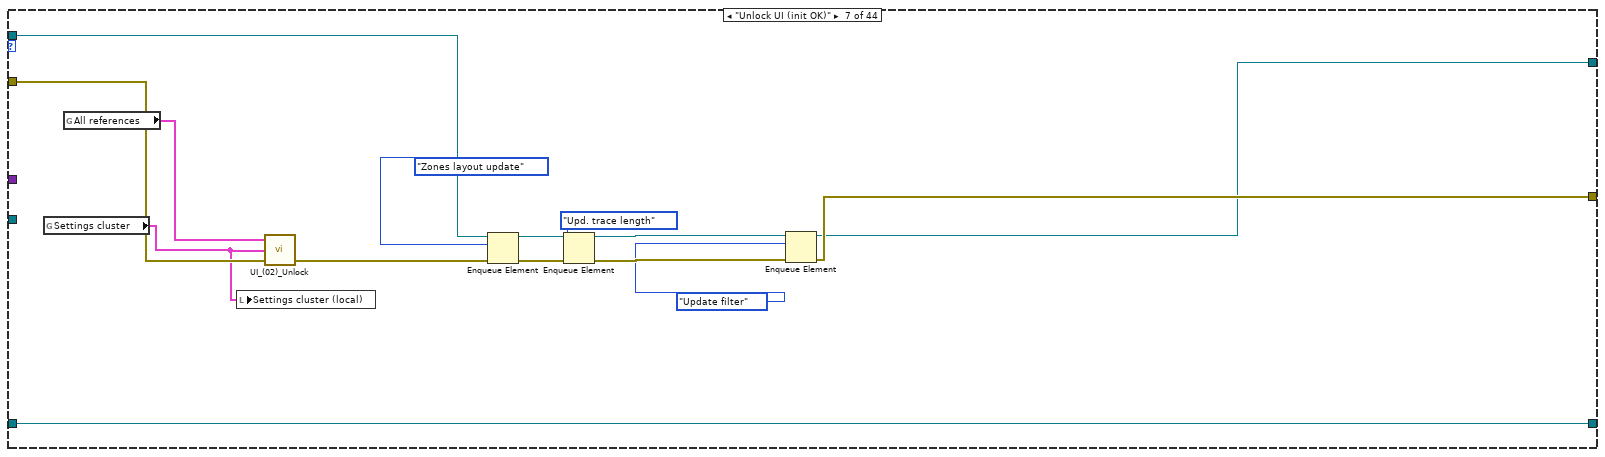
[diagram p17: hidden frame]
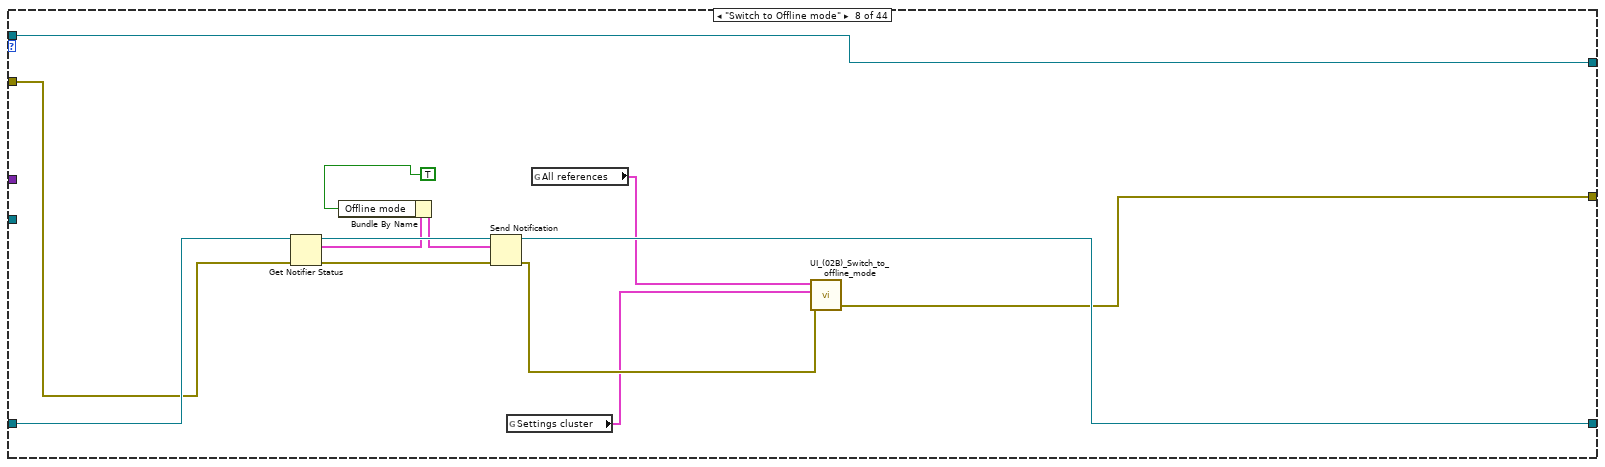
[diagram p18: hidden frame]
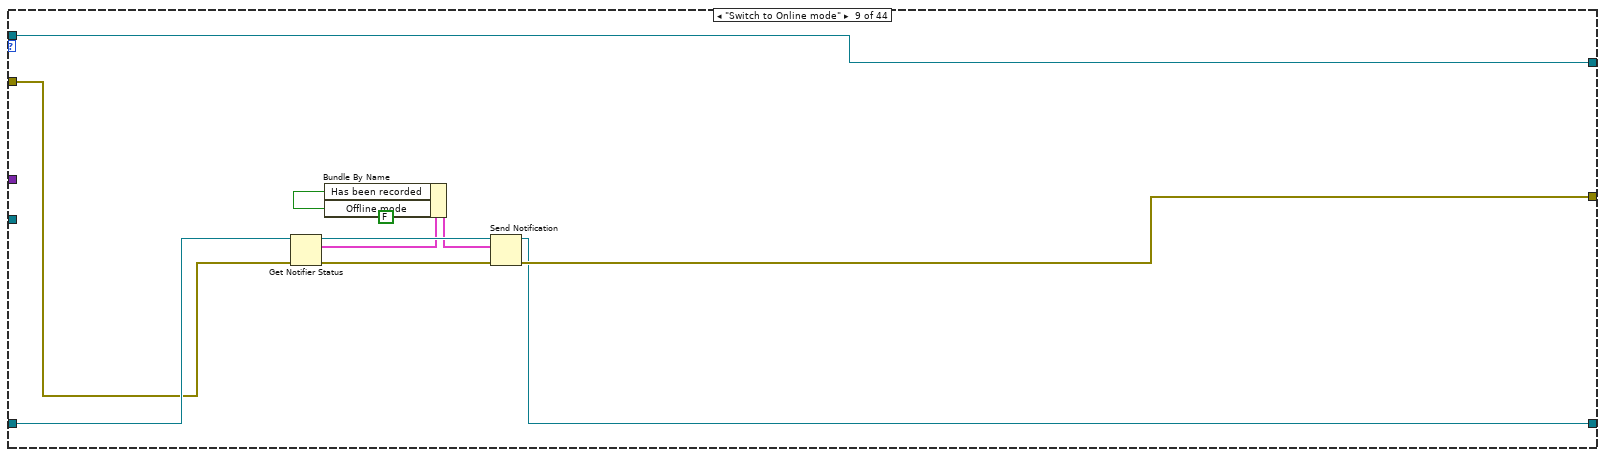
[diagram p19: hidden frame]
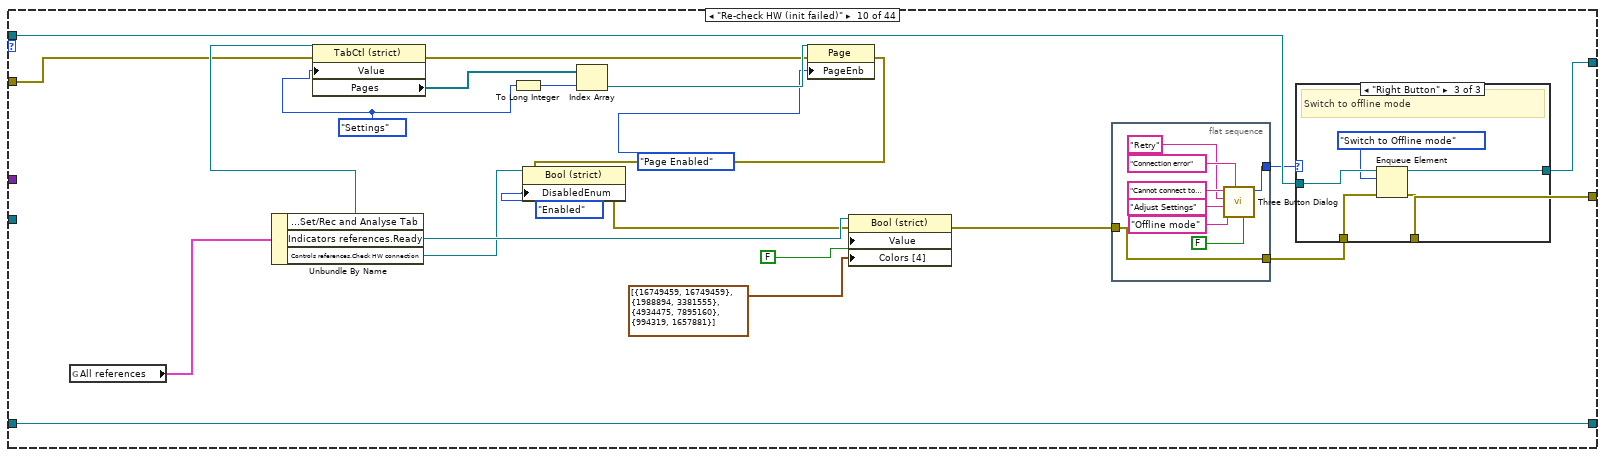
[diagram p20: hidden frame]
diagram:
  w50 = i64 31 ("Period")
  n1 = disable-structure shown="Default" {
    disable-tunnel: [w85] -> w4
    frame Enabled {
      w97 = timestamp(0 s since 1904-01-01) ("Start time (SW)")
      w96 = u32 0 ("TTL in time (HW)")
      # "All controls should sit here"
      n2 = control-ref of="Since track start"() -> (w118:refnum<vi>)
      n3 = control-ref of="Mouse speed, mm/s"() -> (w117:refnum<vi>)
      n4 = control-ref of="Running, perc. of time"() -> (w116:refnum<vi>)
      n5 = control-ref of="Histograms"() -> (w83:refnum<vi>)
      n6 = control-ref of="HW info"() -> (w122:refnum<vi>)
      n7 = control-ref of="Port"() -> (w121:refnum<vi>)
      n8 = control-ref of="Ready"() -> (w120:refnum<vi>)
      n9 = control-ref of="Current Time"() -> (w119:refnum<vi>)
      n10 = control-ref of="Run distance, m"() -> (w82:refnum<vi>)
      n11 = control-ref of="Cage size"() -> (w104:refnum<vi>)
      n12 = control-ref of="Reward and stimulation"() -> (w87:refnum<vi>)
      n13 = control-ref of="Current zone"() -> (w84:refnum<vi>)
      n14 = control-ref of="IO status indicator"() -> (w112:refnum<vi>)
      n15 = control-ref of="Mouse speed"() -> (w80:refnum<vi>)
      n16 = Bundle(cluster="Indicators references", "HW info"=w122, "Port"=w121, "Ready"=w120, "IO status indicator"=w112, "Current Time"=w119, "Record timestamp"=w118, "Mouse speed"=w80, "Mouse speed, mm/s"=w117, "Running, perc. of time"=w116, "Histograms"=w83, "Cage size"=w104, "Reward"=w87, "Current zone"=w84, "Run length, m"=w82) -> (w109:T34)
      n17 = property on="Indicators references" class="Clust (strict)"("Value"=w109) -> ()  [unwired: 2 in, 2 out]
      n18 = control-ref of="Add Reward"() -> (w90:refnum<vi>)
      n19 = control-ref of="Modify Reward"() -> (w89:refnum<vi>)
      n20 = control-ref of="Remove Reward"() -> (w88:refnum<vi>)
      n21 = control-ref of="This VI"() -> (w114:refnum<vi>)
      n22 = control-ref of="Start over"() -> (w79:refnum<vi>)
      n23 = control-ref of="Playback speed"() -> (w125:refnum<vi>)
      n24 = control-ref of="Check HW connection"() -> (w138:refnum<vi>)
      n25 = control-ref of="Save settings"() -> (w137:refnum<vi>)
      n26 = control-ref of="Reset zones"() -> (w136:refnum<vi>)
      n27 = control-ref of="Reset stimuli"() -> (w135:refnum<vi>)
      n28 = control-ref of="Record/Stop"() -> (w134:refnum<vi>)
      n29 = control-ref of="Reset barplot"() -> (w133:refnum<vi>)
      n30 = control-ref of="Multiplyer of chart RX"() -> (w132:refnum<vi>)
      n31 = control-ref of="Show zones"() -> (w131:refnum<vi>)
      n32 = control-ref of="Show magnets"() -> (w113:refnum<vi>)
      n33 = control-ref of="Show heatmap"() -> (w130:refnum<vi>)
      n34 = control-ref of="Show full track"() -> (w129:refnum<vi>)
      n35 = control-ref of="Open File"() -> (w128:refnum<vi>)
      n36 = control-ref of="Play/Pause"() -> (w127:refnum<vi>)
      n37 = control-ref of="Trace, s"() -> (w126:refnum<vi>)
      n38 = control-ref of="Timeline"() -> (w124:refnum<vi>)
      n39 = control-ref of="Cage radial segmentation"() -> (w106:refnum<vi>)
      n40 = control-ref of="Set IO config"() -> (w105:refnum<vi>)
      n41 = control-ref of="Set/Rec and Analyse Tab"() -> (w107:refnum<vi>)
      n42 = control-ref of="By Zone stim. setup"() -> (w123:refnum<vi>)
      n43 = control-ref of="Rainbow (time)"() -> (w102:refnum<vi>)
      n44 = control-ref of="Rainbow (speed)"() -> (w101:refnum<vi>)
      n45 = control-ref of="Pane"() -> (w115:refnum<vi>)
      n46 = control-ref of="Speed threshold"() -> (w81:refnum<vi>)
      n47 = Current VI's Menubar() -> (w103:refnum<k9>)
      n48 = Bundle(cluster="Panes references", "Pane"=w115, "This VI"=w114, "Menu"=w103) -> (w110:T33)
      n49 = Initialize Array(FALSE ("Activation"), 9 ("dimension size")) -> (w74:bool[])
      n50 = property on="Panes references" class="Clust (strict)"("Value"=w110) -> ()  [unwired: 2 in, 2 out]
      n51 = Bundle(cluster="Controls references", "Check HW connection"=w138, "Save settings"=w137, "Reset zones"=w136, "Reset stimuli"=w135, "Record/Stop"=w134, "Reset barplot"=w133, "Multiplyer of chart RX"=w132, "Show zones"=w131, "Show magnets"=w113, "Show heatmap"=w130, "Show full track"=w129, "Open File"=w128, "Play/Pause"=w127, "Trace, s"=w126, "Playback speed"=w125, "Timeline"=w124, "By Zone stim. setup"=w123, "Set/Rec and Analyse Tab"=w107, "Cage radial segmentation"=w106, "Set IO config"=w105, "Rainbow (time)"=w102, "Rainbow (speed)"=w101, "Add Reward"=w90, "Modify Reward"=w89, "Delete Reward"=w88, "Speed threshold, mm/s"=w81, "Start Over"=w79) -> (w94:T35)
      n52 = Array To Cluster(array=w74) -> (cluster=→"Active rules":T40)
      n53 = Bundle By Name(cluster="All references", "Service references"=w110, "Controls references"=w94, "Indicators references"=w109) -> (w108:T36)
      n54 = property on="Controls references" class="Clust (strict)"("Value"=w94) -> ()  [unwired: 2 in, 2 out]
      n55 = global write "SW_Globals_2.2+.vi" "All references"(w108) -> ()
      n56 = call "SW_Init_Array_of_Conditions.vi"("error in (no error)"="error in (no error)") -> ("error out"=w85:T41, "Array of conditions"=→"Array of conditions":T6)  [unwired: 1 in]
      n57 = property on="All references" class="Clust (strict)"("Value"=w108) -> ()  [unwired: 2 in, 2 out]
      "FPS status" <- 0 ("FPS status")
      "Sensor board size" <- "" ("Sensor board size")
      "Start time (SW)" <- w97
      "TTL in time (SW)" <- w97
      "Key_pressed" <- "----" ("Key_pressed")
      "TTL in time (HW)" <- w96
      "Start time (HW)" <- w96
      "Track show state" <- u32 0 ("Track show state")
      "Frame #" <- u32 0 ("Frame #")
    }
  }
  n58 = disable-structure shown="Disabled" {
    disable-tunnel: [w140 _] -> w16
    disable-tunnel: [w139 _] -> w15
    frame Disabled {
      n59 = call "Obtain Broadcast Events for Registration.vi"() -> ("error out"=w139:errorcluster, "Tracks Repair Broadcast Events"=w140:T42)  [unwired: 9 in, 1 out]
    }
    frame Enabled {
    }
  }
  n60 = call "Obtain Broadcast Events for Registration.vi"() -> ("error out"=w7:errorcluster, "Stream Data Broadcast Events"=w9:T43)  [unwired: 9 in, 1 out]
  n61 = call "Obtain Broadcast Events for Registration.vi"() -> ("error out"=w5:errorcluster, "TTL IO Broadcast Events"=w6:T44)  [unwired: 9 in, 1 out]
  n62 = call "Obtain Broadcast Events for Registration.vi"() -> ("error out"=w2:errorcluster, "Cage Diagram Broadcast Events"=w1:T45)  [unwired: 9 in, 1 out]
  n63 = disable-structure shown="Default" {
    disable-tunnel: w4 -> [w150]
    disable-tunnel: [w149] -> w23
    disable-tunnel: [w148] -> w19
    disable-tunnel: [w142] -> w22
    disable-tunnel: [w141] -> w24
    frame Enabled {
      w144 = T46 {"Acq. is ON"=FALSE, "Playing loaded"=FALSE, "Recording now"=FALSE, "Has been recorded"=FALSE, "Data saved"=FALSE, "Data loaded"=FALSE, "Calibration mode"=FALSE, "Offline mode"=FALSE, "Stop and Exit"=FALSE, "Updating layout"=FALSE} ("States cluster")
      w151 = CTL_Control_States."SW Init"
      # "Software Init starts here"
      n64 = call-poly <vilib>:"Create Timing Source.vi"("error in (no error)"=w150, "name (in)"="1 kHz (tracker app)") -> ("error out"=w157:errorcluster, "name (out)"=w148:string)  [unwired: 8 in]
      n65 = property on="Timing Source" class="Str"(error in=w157, "Value"=w148) -> (error out=w155:errorcluster)  [unwired: 1 in, 1 out]
      n66 = Obtain Queue(name (unnamed)="Control", element data type=w151, error in (no error)=w155) -> (queue out=w152:refnum<queue>, error out=w153:errorcluster)  [unwired: 2 in, 1 out]
      n67 = Enqueue Element(queue=w152, element=w151, error in (no error)=w153) -> (queue out=w149:refnum<queue>, error out=w147:errorcluster)  [unwired: 1 in, 1 out]
      n68 = Obtain Notifier(name (unnamed)="States", notification data type=w144, error in (no error)=w147) -> (notifier out=w143:refnum<notifier>, error out=w145:errorcluster)  [unwired: 1 in, 1 out]
      n69 = Send Notification(notification=w144, notifier=w143, error in (no error)=w145) -> (notifier out=w142:refnum<notifier>, error out=w141:errorcluster)
    }
  }
  n70 = call "SW_Get_CPU_load_monitor_reference.vi"("error in (no error)"=w24) -> ("error out"=w37:errorcluster, "CPU monitor .NET reference"=w36:refnum<k24>)  [unwired: 1 in]
  n71 = local write "UI update period"(w50) -> ()
  n72 = Merge Errors(w15, w7, w5, w2) -> (w8:errorcluster)
  n73 = register-events "DQMH_REG_EVENTS"(error in=w8, w16, w9, w6, w1) -> (reference out=w13:refnum<event-registration>, error out=w14:errorcluster)  [unwired: 1 in]
  n74 = node-c288(w19, i64 1 ("Period"), 65000 ("Priority"), "Data_gathering" ("Structure Name"), w24) -> (w60:T48)
  n75 = node-c288(w19, w50, 500 ("Priority"), "UI_update" ("Structure Name"), w24) -> (w54:T48)
  n76 = node-c288(w19, i64 47 ("Period"), 5000 ("Priority"), "Dispatcher" ("Structure Name"), w24) -> (w72:T48)
  n77 = Merge Errors(w24, w14) -> (w17:errorcluster)
  n78 = timed-loop {
    timing: w60 -> [_]
    timing-out: [_] -> w59
    tunnel: w23 -> [_]
    tunnel: w22 -> [w168]
    border: "" -> [_]
    tunnel: [w164] -> w27
    tunnel: [w161] -> w26
    tunnel: [w158] -> w28
    stop <- w167 stop-if-true
    # "Data gathering and initial processing loop + recorded data streaming"
    n79 = node-c288() -> (w162:errorcluster)  [unwired: 1 in]
    n80 = Get Notifier Status(notifier=w168, error in (no error)=w162) -> (current notification=w159:T46, error out=w163:errorcluster)  [unwired: 3 out]
    n81 = Unbundle By Name(w159) -> ("Acq. is ON"=w166:bool, "Stop and Exit"=w167:bool)
    n82 = case shown="True" w166 {
      tunnel: w163 -> [w170 w229]
      tunnel: [w171 w223] -> w165
      tunnel: [_ w222] -> w164
      tunnel: [_ w221] -> w161
      tunnel: [w173 i64 1] -> w160
      tunnel: w159 -> [w179 _]
      tunnel: [w169 _] -> w158
      frame False {
        # "This part in certain conditions will be used for offline data streaming from loaded files"
        n83 = local read "Play/Pause"() -> (w172:bool)
        n84 = Unbundle By Name(w179) -> ("Data loaded"=w175:bool, "Offline mode"=w177:bool, "Stop and Exit"=w178:bool)
        n85 = Not(x=w178) -> (.not. x?=w176:bool)
        n86 = Compound Arithmetic op=AND(w172, w175, w177, w176) -> (w174:bool)
        n87 = case shown="True" w174 {
          tunnel: [i64 101 w187] -> w173
          tunnel: [w180 w209] -> w171
          tunnel: w170 -> [w180 w209]
          tunnel: [_ w198] -> w169
          frame False {
            # "Some conditionas are not met"
          }
          frame True {
            # "Data loaded, oflline mode is on and we are good to stream loaded data"
            n88 = local read "Timeline min&max indices"() -> (w208:T26)
            n89 = local read "Loaded.zones"() -> (w191:i8[])
            n90 = local read "Loaded.timeline"() -> (w214:dbl[])
            n91 = local read "Loaded.X"() -> (w213:dbl[])
            n92 = local read "Loaded.Y"() -> (w212:dbl[])
            n93 = local read "Loaded.alpha"() -> (w211:dbl[])
            n94 = local read "Loaded.speed"() -> (w210:dbl[])
            n95 = local read "Act. frame time, s"() -> (w188:dbl)
            n96 = Unbundle(w208) -> ("Tl. min index"=w205:i32, "Tl. max index"=w195:i32)
            n97 = local read "Playback speed"() -> (w189:u16)
            n98 = expression code="x * 8.333333"(w188) -> (w218:dbl)
            n99 = local read "Cur. pos. slider index"() -> (w197:i32)
            n100 = local read "Update timeline index?"() -> (w196:bool)
            n101 = feedback #1(w205) -> (w192:i32)
            n102 = Index Array(array=w214, index=w192) -> (element=w204:dbl)
            n103 = Index Array(array=w213, index=w192) -> (element=w203:dbl)
            n104 = Index Array(array=w212, index=w192) -> (element=w202:dbl)
            n105 = Index Array(array=w211, index=w192) -> (element=w201:dbl)
            n106 = Index Array(array=w210, index=w192) -> (element=w200:dbl)
            n107 = Index Array(array=w191, index=w192) -> (element=w190:i8)
            n108 = Build Array(w204, w203, w202, w201, w200, w190) -> (w199:dbl[])
            n109 = Increment(x=w192) -> (x+1=w194:i32)
            n110 = Multiply(x=w189, y=w218) -> (x*y=w184:dbl)
            n111 = call <extravilib>:"Write.vi"("element"=w199) -> ("channel"=w198:T53)  [unwired: 8 in, 2 out]
            n112 = feedback #2(0.0) -> (w182:dbl)
            n113 = Add(x=w182, y=w184) -> (x+y=w183:dbl)
            n114 = Select(t=w197, s=w196, f=w194) -> (s? t:f=w193:i32)
            n115 = case shown="True" w196 {
              frame False {
              }
              frame True {
                n116 = local write "Update timeline index?"(FALSE ("Update timeline index?")) -> ()
              }
            }
            n117 = Greater Or Equal?(x=w193, y=w195) -> (x >= y?=w207:bool)
            n118 = To Quad Integer(1:w183) -> (0:w217:i64)
            n119 = Select(t=w205, s=w207, f=w193) -> (s? t:f=w206:i32)
            n120 = feedback-in #1(w206) -> ()
            n121 = In Range and Coerce(upper limit=i64 1000, x=w217, lower limit=i64 1) -> (coerced(x)=w187:i64)  [unwired: 1 out]
            n122 = Subtract(x=w183, y=w187) -> (x-y=w185:dbl)
            n123 = feedback-in #2(w185) -> ()
          }
        }
      }
      frame True {
        # "Data gathering in online mode happens here"
        n124 = local read "VISA resource name"() -> (w227:refnum<visa-resource-name>)
        n125 = call "HW_Get_data_flow_from_serial_port.vi"("error in"=w229, "VISA resource name in"=w227) -> ("Not empty?"=w228:bool, "error out"=w224:errorcluster, "Timestamp"=w225:timestamp, "Data"=w226:string)  [unwired: 2 in, 1 out]
        n126 = case shown="True" w228 {
          tunnel: w226 -> [_ w245]
          tunnel: w225 -> [_ w244]
          tunnel: w224 -> [w230 w248]
          tunnel: [w230 w239] -> w223
          tunnel: [_ w234] -> w222
          tunnel: [_ w233] -> w221
          frame False {
          }
          frame True {
            n127 = global read "SW_Globals_2.2+.vi" "Settings cluster"() -> (w236:T16)
            n128 = local read "Ports IO config"() -> (w242:bool[])
            n129 = local read "SB size"() -> (w235:u8)
            n130 = feedback #3() -> (w246:string)
            n131 = Concatenate Strings(w246, w245) -> (w243:string)
            n132 = local read "Calibration parameters"() -> (w232:T23)
            n133 = Unbundle By Name(w236) -> ("IO parameters.IO inversion config."=w241:u16)
            n134 = call "FL_Decode_RAW_to_DEC_2.vi"("SB size (loc. var. only)"=w235, "IO ports config"=w242, "Input string"=w243, "Input timestamp"=w244, "IO inversion config."=w241, "Error In"=w248) -> ("Output string leftover"=w247:string, "DEC output cluster"=w238:T54, "Error Out"=w240:errorcluster)
            n135 = feedback-in #3(w247) -> ()
            n136 = Unbundle By Name(w238) -> ("Frame OK"=w237:bool)
            n137 = local read "Frame #"() -> (w231:u32)
            n138 = case shown="True" w237 {
              tunnel: w238 -> [_ w277]
              tunnel: w240 -> [w249 w252]
              tunnel: [w249 w252] -> w239
              tunnel: w236 -> [_ w274]
              tunnel: w235 -> [_ w270]
              tunnel: [_ w261] -> w234
              tunnel: [_ w254] -> w233
              tunnel: w232 -> [_ w264]
              tunnel: w231 -> [_ w256]
              frame False {
              }
              frame True {
                n139 = Unbundle By Name(w264) -> ("True frame time, s"=w263:dbl)
                n140 = Unbundle By Name(w274) -> ("Geometry.Bridge H. offset"=w276:sgl, "Geometry.Bridge V. offset"=w275:sgl, "Geometry.Magnets orientation"=w251:sgl, "Geometry.Twisted neck"=w268:bool, "Geometry.Bridge swap"=w269:bool)
                n141 = local read "Pre-filter params."() -> (w265:T28)
                n142 = Increment(x=w256) -> (x+1=w255:u32)
                n143 = local write "Frame #"(w255) -> ()
                n144 = First Call?() -> (First Call?: T/F=w266:bool)
                n145 = Equal To 0?(x=w251) -> (x = 0?=w250:bool)
                n146 = call "FL_Adjust_raw_magnets_coords.vi"("Offset H."=w276, "Offset V."=w275, "Alternative magnets orientation"=w250, "DEC cluster in"=w277) -> ("DEC cluster out"=w273:T54)  [unwired: 3 in]
                n147 = call "FL_DEC_split_3_and_prefilter_(online).vi"("Initialize? (F)"=w266, "Pre-filter params."=w265, "DEC input cluster"=w273) -> ("Magnets coords raw"=w257:T55, "Magnets coords"=w272:cluster{"X1":dbl, "Y1":dbl, "X2":dbl, "Y2":dbl}, "TTLs"=w259:cluster{"TTL input":i16, "TTL output":i16}, "Times"=w260:T56)  [unwired: 3 in]
                n148 = call "FL_Calculate_Coordinates_Diff_R_Center.vi"("Frame time, s"=w263, "Magnets coords in"=w272) -> ("Output cluster of data"=w271:T57)  [unwired: 1 in]
                n149 = call "CALC_Phi_theta_etc_3_(online).vi"("Current frame #"=w255, "Twisted neck"=w268, "Use alternative magnets orientation"=w250, "Bridge swap"=w269, "SB size"=w270, "Input cluster of data"=w271) -> ("Animal coordinates"=w258:T25)  [unwired: 1 in]
                n150 = Bundle By Name(cluster=T51 {"Times"={"ms since ON"=0, "delta time"=0, "Frame timestamp"=timestamp(0 s since 1904-01-01)}, "TTLs"={"TTL input"=0, "TTL output"=0}, "Animal coordinates"={"R from center"=0.0, "phi (mouse angular position in the cage)"=0.0, "alpha (mouse rot. angle)"=0.0, "X"=0.0, "Y"=0.0, "theta (from center towards mouse)"=0.0, "beta (cage rot. against mouse)"=0.0, "w (mouse angle to wall)"=0.0, "Speed (filtered)"=0.0}, "Magnets coords raw"={"X1 raw"=0.0, "Y1 raw"=0.0, "X2 raw"=0.0, "Y2 raw"=0.0}, "Measurements and statistics"={"Zone #"=0, "Histogram"=[], "Running, perc. of time"=0.0, "Run, meters"=0.0, "Avg. speed"=0.0}} ("Data in"), "Times"=w260, "TTLs"=w259, "Animal coordinates"=w258, "Magnets coords raw"=w257) -> (w253:T51)
                n151 = call <extravilib>:"Write.vi"("element"=w258) -> ("channel"=w261:T58)  [unwired: 8 in, 2 out]
                n152 = call <extravilib>:"Write.vi"("size (unlimited)"=250, "element"=w253) -> ("channel"=w254:T59)  [unwired: 7 in, 2 out]
              }
            }
          }
        }
      }
    }
    n153 = node-c288(w165, w160) -> ()  [unwired: 1 out]
  }
  n154 = timed-loop {
    timing: w72 -> [_]
    timing-out: [_] -> w71
    tunnel: w23 -> [w298]
    tunnel: [w292] -> w67
    tunnel: w22 -> [w295]
    tunnel: [w294] -> w44
    shift-right: [w288] -> _
    shift-left: variant ("Error data") -> [w285]
    tunnel: w13 -> [w284]
    stop <- w296 stop-if-true
    # "Init and Dispatcher loop"
    n155 = node-c288() -> (w287:errorcluster)  [unwired: 1 in]
    n156 = Dequeue Element(queue=w298, error in (no error)=w287) -> (queue out=w297:refnum<queue>, element=w289:T47, error out=w286:errorcluster)  [unwired: 1 in, 1 out]
    n157 = case shown="\"Process loaded settings\"" w289 {
      tunnel: [w301 w317 w371 w443 w482 w522 w537 w560 w570 w585 w633 w663 w715 w726 w759 w803 w844 w890 w920 w962 w1010 w1031 w1090 w1181 w1221 w1321 w1363 w1406 w1474 w1488 w1539 w1616 w1647 w1703 w1712 w1737 w1784 w1794 w1820 w1836 w1865 w1897 w1914 w1963] -> w293
      tunnel: w297 -> [w301 w317 w360 w444 w483 w522 w544 w560 w570 w586 w634 w663 w715 w727 w759 w798 w844 w890 w920 w963 w1009 w1032 w1091 w1182 w1222 w1322 w1364 w1407 w1474 w1486 w1558 w1616 w1648 w1703 w1712 w1738 w1784 w1795 w1821 w1837 w1865 w1897 w1914 w1963]
      tunnel: [_ _ _ _ _ _ _ _ _ _ _ _ _ _ _ _ _ _ _ _ _ _ _ _ _ _ _ _ _ _ _ _ _ _ _ _ _ _ _ _ _ _ _ TRUE] -> w296
      tunnel: [w300 w307 w362 w450 w504 w523 w538 w550 w565 w584 w632 w664 w695 w724 w758 w791 w840 w889 w915 w961 w1008 w1033 w1087 w1183 w1223 w1323 w1365 w1408 w1472 w1487 w1540 w1580 w1650 w1701 w1715 w1741 w1778 w1793 w1812 w1838 w1856 w1894 w1911 w1936] -> w291
      tunnel: w286 -> [w300 w314 w368 w451 w505 w528 w547 w558 w568 w579 w627 w664 w701 w736 w771 w805 w845 w891 w921 w968 w1006 w1037 w1095 w1187 w1227 w1327 w1369 w1421 w1473 w1502 w1528 w1586 w1658 w1704 w1718 w1744 w1783 w1803 w1828 w1847 w1863 w1890 w1912 w1944]
      tunnel: w295 -> [w299 w318 w367 w432 w486 w532 w534 w559 w569 w574 w622 w661 w710 w723 w763 w799 w846 w892 w922 w969 w1001 w1038 w1096 w1188 w1228 w1328 w1370 w1415 w1475 w1496 w1538 w1606 w1659 w1683 w1719 w1745 w1785 w1804 w1829 w1853 w1857 w1891 w1908 w1955]
      tunnel: [w299 w318 w367 w432 w486 w532 w534 w555 w564 w574 w622 w661 w694 w723 w763 w799 w841 w885 w916 w964 w1002 w1034 w1092 w1184 w1224 w1324 w1366 w1415 w1475 w1496 w1538 w1606 w1649 w1683 w1714 w1740 w1785 w1804 w1829 w1853 w1857 w1891 w1908 w1948] -> w294
      tunnel: w285 -> [_ w315 _ _ _ _ _ _ _ _ _ _ _ _ _ _ _ _ _ _ _ _ _ _ _ _ _ _ _ _ _ _ _ _ _ _ _ _ _ _ _ _ _ _]
      tunnel: w284 -> [_ _ w344 _ _ _ _ _ _ _ _ _ _ _ _ _ _ _ _ _ _ _ _ _ _ _ _ _ w1471 _ _ _ _ _ _ _ _ _ _ _ _ _ _ _]
      frame Default {
      }
      frame "IDL Error" {
        w311 = T68 1 items=["no dialog", "OK message", "continue or stop message", "OK message + warnings", "continue/stop + warnings"] ("type of dialog (OK msg:1)")
        w316 = T69 {"Previous step"=enum."SW Init", "error IO"={"status"=FALSE, "code"=0, "source"=""}}  # Error Data
        n158 = Variant To Data(error in=w314, type=w316, Variant=w315) -> (data=w313:T69)  [unwired: 1 out]
        n159 = Unbundle(w313) -> ("Previous step"=w310:T47, "error IO"=w312:errorcluster)
        n160 = Format Into String(format string="%s", w310) -> (resulting string=w306:string)  [unwired: 2 in, 1 out]
        n161 = call "Build Text"("stage"=w306) -> ("Result"=w305:string)  [unwired: 13 in, 1 out]
        n162 = call "Display Message to User2"("Enable"=TRUE, "Message"=w305) -> ("error out"=w302:errorcluster)  [unwired: 8 in, 1 out]
        n163 = Merge Errors(w302, w312) -> (w303:errorcluster)
        n164 = call <vilib>:"Simple Error Handler.vi"("type of dialog (OK msg:1)"=w311, "error in (no error)"=w303) -> ("error out"=w308:errorcluster)  [unwired: 3 in, 4 out]
        n165 = call <vilib>:"Clear Errors.vi"("error in (no error)"=w308) -> ("error out"=w307:errorcluster)  [unwired: 5 in, 1 out]
      }
      frame "SW Init" {
        w319 = FALSE
        w373 = T68 0 items=["no dialog", "OK message", "continue or stop message", "OK message + warnings", "continue/stop + warnings"] ("type of dialog (OK msg:1)")
        n166 = call "Start Module.vi"() -> ("error out"=w340:errorcluster, "Wait for Event Sync?"=w341:bool, "Stream Data Broadcast Events"=w342:T43)  [unwired: 8 in, 1 out]
        n167 = call "Start Module.vi"() -> ("error out"=w336:errorcluster, "Wait for Event Sync?"=w335:bool, "TTL IO Broadcast Events"=w338:T44)  [unwired: 8 in, 1 out]
        n168 = call "Start Module.vi"() -> ("error out"=w331:errorcluster, "Wait for Event Sync?"=w328:bool, "Cage Diagram Broadcast Events"=w330:T45)  [unwired: 8 in, 1 out]
        n169 = local read "Load custom? (F)"() -> (w358:bool)
        n170 = property class="App"(error in=w368) -> (error out=w379:errorcluster, "App.Kind"=w375:T70)  [unwired: 1 in, 1 out]
        n171 = Merge Errors(w340, w336, w331) -> (w337:errorcluster)
        n172 = register-events(reference=w344, error in=w337, w342, w338, w330) -> (error out=w329:errorcluster)  [unwired: 1 in, 1 out]
        n173 = case shown="True" w358 {
          tunnel: [w385 w394] -> w359
          tunnel: w375 -> [w387 w397]
          tunnel: [_ FALSE] -> w357
          tunnel: [w385 w393] -> w354
          frame False {
            n174 = case shown="\"Development System\"" w387 {
              tunnel: [w389 w390 w391] -> w388
              frame "invalid app kind", Default {
                n175 = call <vilib>:"Application Directory.vi"() -> ("Application Directory"=w389:path)
              }
              frame "Run Time System" {
                n176 = call <vilib>:"Application Directory.vi"() -> ("Application Directory"=w390:path)
              }
              frame "Development System" {
                n177 = Current VI's Path() -> (path=w392:path)
                n178 = Strip Path(path=w392) -> (stripped path=w391:path)  [unwired: 1 out]
              }
            }
            n179 = Build Path(base path=w388, name or relative path=path "Tracker_settings.tcf") -> (appended path=w385:path)
          }
          frame True {
            n180 = case shown="\"Development System\"" w397 {
              tunnel: [w399 w400 w401] -> w398
              frame "invalid app kind", Default {
                n181 = call <vilib>:"Application Directory.vi"() -> ("Application Directory"=w399:path)
              }
              frame "Run Time System" {
                n182 = call <vilib>:"Application Directory.vi"() -> ("Application Directory"=w400:path)
              }
              frame "Development System" {
                n183 = Current VI's Path() -> (path=w402:path)
                n184 = Strip Path(path=w402) -> (stripped path=w401:path)  [unwired: 1 out]
              }
            }
            n185 = local read "Settings path to load"() -> (w394:path)
            n186 = Build Path(base path=w398, name or relative path=path "Tracker_settings.tcf") -> (appended path=w393:path)
          }
        }
        n187 = global read "SW_Globals_2.2+.vi" "All references"() -> (w365:T36)
        n188 = call "Synchronize Module Events.vi"("error in (no error)"=w329, "Wait for Event Sync?"=w341) -> ("error out"=w339:errorcluster)  [unwired: 9 in]
        n189 = call "Synchronize Module Events.vi"("error in (no error)"=w329, "Wait for Event Sync?"=w335) -> ("error out"=w334:errorcluster)  [unwired: 9 in]
        n190 = call "Synchronize Module Events.vi"("error in (no error)"=w329, "Wait for Event Sync?"=w328) -> ("error out"=w327:errorcluster)  [unwired: 9 in]
        n191 = Merge Errors(w379, w339, w334, w327) -> (w343:errorcluster)
        n192 = disable-structure shown="RUN_TIME_ENGINE==True, Default" {
          disable-tunnel: [w383 "2.x.x.x dev." ("App Version Info")] -> w348
          disable-tunnel: [w382 _] -> w346
          frame condition #0 {
            n193 = Current VI's Path() -> (path=w381:path)
            n194 = call "Get File Version Info.vi"("File path"=w381) -> ("error out"=w382:errorcluster, "File Version"=w383:string)  [unwired: 1 in]
          }
          frame condition #1 (active) {
          }
        }
        n195 = control-ref of="Reward and stimulation"() -> (w363:refnum<vi>)
        n196 = local write "Load custom? (F)"(w357) -> ()
        n197 = call "SW_Load_settings_to_main_tab_4.vi"("Settings path in"=w359, "Researcher name"="Researcher", "error in (no error)"=w343) -> ("Settings cluster out"=w322:T16, "Error Out"=w326:errorcluster)  [unwired: 5 in, 1 out]
        n198 = Unbundle By Name(w322) -> ("Geometry"=w321:T19)
        n199 = Concatenate Strings("Locomotion tracking software [v." ("string"), w348, "]" ("string")) -> (w351:string)
        n200 = Bundle("Geometry"=w321, w319, w319) -> (w320:cluster{"Geometry":T19, bool, bool})  [unwired: 1 in]
        n201 = control-ref of="This VI"() -> (w352:refnum<vi>)
        n202 = call "New Layout (instant).vi"("error in (no error)"=w326, "Cage parameters"=w320) -> ("Reply Payload"=w325:T71)  [unwired: 7 in, 2 out]
        n203 = global read "SW_Globals_2.2+.vi" "Paths"() -> (w378:T77)
        n204 = Bundle By Name(cluster=w378, "Program settings"=w354) -> (w377:T77)
        n205 = Unbundle By Name(w325) -> ("Cage Diagram ref"=w324:T15, "New Layout (instant)_error"=w323:errorcluster)
        n206 = Merge Errors(w323, w346) -> (w347:errorcluster)
        n207 = property class="VI"(reference=w352, error in=w347, "Front Panel.Title"=w351) -> (error out=w349:errorcluster)  [unwired: 1 out]
        n208 = local write "Diagram (display)"(w324) -> ()
        n209 = global write "SW_Globals_2.2+.vi" "Paths"(w377) -> ()
        n210 = call "UI_(01)_Set_startup_controls_state.vi"("error in (no error)"=w349, "Settings cluster in"=w322, "All references in"=w365) -> ("error out"=w353:errorcluster, "Settings cluster out"=w333:T16, "All references out"=w380:T36)
        n211 = Unbundle By Name(w333) -> ("Calibration parameters"=w364:T23, "Calibration parameters.True frame time, s"=w366:dbl, "Conditions presets array"=w361:T6, "IO parameters"=w355:T22)
        n212 = global write "SW_Globals_2.2+.vi" "All references"(w380) -> ()
        n213 = global write "SW_Globals_2.2+.vi" "Settings cluster"(w333) -> ()
        n214 = local write "Settings cluster (local)"(w333) -> ()
        n215 = call <vilib>:"Simple Error Handler.vi"("error code (no error:0)"=0, "type of dialog (OK msg:1)"=w373, "error in (no error)"=w353) -> ("error?"=w372:bool, "error out"=w370:errorcluster)  [unwired: 2 in, 3 out]
        n216 = local write "IO parameters"(w355) -> ()
        n217 = call "SW_get_config_of_Zones_and_IO_2.vi"("Sync parameters cluster input"=w355) -> ("Ports IO config (OUT is FALSE)"=w356:bool[])  [unwired: 3 out]
        n218 = local write "Calibration parameters"(w364) -> ()
        n219 = local write "Act. frame time, s"(w366) -> ()
        n220 = case shown="False" w372 {
          tunnel: w360 -> [w407 w414]
          tunnel: [w406 w413] -> w371
          tunnel: w370 -> [w404 w410]
          tunnel: [w403 w411] -> w369
          frame False {
            n221 = Enqueue Element(queue=w407, element=CTL_Control_States."HW Init", error in (no error)=w404) -> (queue out=w406:refnum<queue>, error out=w403:errorcluster)  [unwired: 1 in, 1 out]
          }
          frame True {
            n222 = call <vilib>:"Simple Error Handler.vi"("error in (no error)"=w410) -> ("error out"=w409:errorcluster)  [unwired: 4 in, 4 out]
            n223 = call <vilib>:"Clear Errors.vi"("error in (no error)"=w409) -> ("error out"=w408:errorcluster)  [unwired: 5 in, 1 out]
            n224 = Enqueue Element(queue=w414, element=CTL_Control_States."Close App", error in (no error)=w408) -> (queue out=w413:refnum<queue>, error out=w411:errorcluster)  [unwired: 1 in, 1 out]
          }
        }
        n225 = local write "Ports IO config"(w356) -> ()
        n226 = local write "Array of conditions"(w361) -> ()
        n227 = call "SW_Generate_Full_Condition(s)_text.vi"("error in (no error)"=w326, "Array of conditions in"=w361, "Calibration parameters"=w364, "TreeControl ref in"=w363) -> ("error out"=w332:errorcluster)  [unwired: 6 in, 1 out]
        n228 = Merge Errors(w369, w332) -> (w362:errorcluster)
      }
      frame "HW Init" {
        w439 = T68 0 items=["no dialog", "OK message", "continue or stop message", "OK message + warnings", "continue/stop + warnings"] ("type of dialog (OK msg:1)")
        n229 = call <vilib>:"Set Busy.vi"("error in (no error)"=w451) -> ("error out"=w416:errorcluster)  [unwired: 9 in, 1 out]
        n230 = global read "SW_Globals_2.2+.vi" "All references"() -> (w457:T36)
        n231 = global read "SW_Globals_2.2+.vi" "Settings cluster"() -> (w425:T16)
        n232 = Unbundle By Name(w457) -> ("Indicators references.HW info"=w456:refnum<vi>, "Indicators references.Ready"=w454:refnum<vi>, "Indicators references.Cage size"=w437:refnum<vi>)
        n233 = Unbundle By Name(w425) -> ("Recording and saving.Acquisition FPS"=w430:T18, "Defaults.VISA Resource Name"=w433:string, "Geometry"=w417:T19)
        n234 = call "Get_cage_size_text_from_Geometry_data.vi"("Error In"=w416, "Geometry"=w417) -> ("Error Out"=w415:errorcluster, "Cage size text"=w436:string)
        n235 = property class="Bool (strict)"(reference=w454, error in=w416, "Value"=FALSE, "Colors [4]"=T60 [{"Numeric Control"=16749459, "Numeric Control"=16176658}, {"Numeric Control"=1988894, "Numeric Control"=3381555}, {"Numeric Control"=4934475, "Numeric Control"=7895160}, {"Numeric Control"=994319, "Numeric Control"=1657881}]) -> (reference out=w449:refnum<vi>, error out=w453:errorcluster)
        n236 = property class="Str"(reference=w437, error in=w415, "Value"=w436) -> (error out=w434:errorcluster)  [unwired: 1 out]
        n237 = property on="VISA resource name" class="VISAName"("Value"=w433) -> ()  [unwired: 2 in, 2 out]
        n238 = call "HW_Setup_2.vi"("VISA resource name in"=w433, "Acquisition FPS"=w430, "Close port? (F)"=FALSE, "error in"=w453) -> ("FPS status"=w429:i32, "Sync capability"=w448:u8, "VISA resource name out"=→"VISA resource name out":refnum<visa-resource-name>, "HW information"=w455:string, "Sensor board size"=w428:string, "SB size"=w426:u8, "Instrument OK?"=w441:bool, "error out"=w423:errorcluster)  [unwired: 3 in, 1 out]
        n239 = local write "FPS status"(w429) -> ()
        n240 = local write "Sensor board size"(w428) -> ()
        n241 = local write "SB size"(w426) -> ()
        n242 = Bundle By Name(cluster=w425, "IO parameters.Sync capability"=w448) -> (w427:T16)
        n243 = call "SW_Clear_Specific_Errors.vi"("Error In"=w423, "Code section"=enum16{"Not Specified", "HW Init"}."HW Init") -> ("Error Out"=w422:errorcluster, "specific error cleared?"=w421:bool)  [unwired: 2 in]
        n244 = property class="Bool (strict)"(reference=w449, error in=w422, "Value"=w441, "Colors [4]"=T60 [{"Numeric Control"=16749459, "Numeric Control"=16749459}, {"Numeric Control"=1988894, "Numeric Control"=3381555}, {"Numeric Control"=4934475, "Numeric Control"=7895160}, {"Numeric Control"=994319, "Numeric Control"=1657881}]) -> (error out=w445:errorcluster)  [unwired: 1 out]
        n245 = Merge Errors(w445, w434) -> (w435:errorcluster)
        n246 = Bundle By Name(cluster=w427, "Geometry.Sensor board size"=w426) -> (w418:T16)
        n247 = call <vilib>:"Simple Error Handler.vi"("type of dialog (OK msg:1)"=w439, "error in (no error)"=w435) -> ("error?"=w440:bool, "error out"=w420:errorcluster)  [unwired: 3 in, 3 out]
        n248 = property on="Property Node" class="Str"(reference=w456, "Value"=w455) -> ()  [unwired: 1 in, 2 out]
        n249 = Compound Arithmetic op=OR(w421, w440) -> (w431:bool)
        n250 = global write "SW_Globals_2.2+.vi" "Settings cluster"(w418) -> ()
        n251 = local write "Settings cluster (local)"(w418) -> ()
        n252 = case shown="False" w431 {
          tunnel: [w460 w464] -> w446
          tunnel: w420 -> [w461 w465]
          tunnel: w444 -> [w458 w467]
          tunnel: [w462 w466] -> w443
          frame True {
            n253 = Enqueue Element(queue=w458, element=CTL_Control_States."Re-check HW (init failed)", error in (no error)=w461) -> (queue out=w462:refnum<queue>, error out=w460:errorcluster)  [unwired: 1 in, 1 out]
          }
          frame False {
            n254 = Enqueue Element(queue=w467, element=CTL_Control_States."Update port info (Init OK)", error in (no error)=w465) -> (queue out=w466:refnum<queue>, error out=w464:errorcluster)  [unwired: 1 in, 1 out]
          }
        }
        n255 = call <vilib>:"Unset Busy.vi"("error in (no error)"=w446) -> ("error out"=w450:errorcluster)  [unwired: 10 in]
      }
      frame "Update port info (Init OK)" {
        w489 = ""  # port:
        w501 = 1 items=["Initializing"=-2, "Unknown"=-1, "Not Present"=0, "Present"=1] ("Devices & Chassis:Is Present")
        n256 = call <vilib>:"Set Busy.vi"("error in (no error)"=w505) -> ("error out"=w496:errorcluster)  [unwired: 9 in, 1 out]
        n257 = call <vilib>:"Initialize Session.vi"("error in (no error)"=w496) -> ("error out"=w499:errorcluster, "Session out"=w500:refnum<k21>)  [unwired: 9 in]
        n258 = global read "SW_Globals_2.2+.vi" "Settings cluster"() -> (w476:T16)
        n259 = call <vilib>:"Create Filter.vi"("error in (no error)"=w499, "Session in"=w500) -> ("error out"=w503:errorcluster, "Filter out"=w502:refnum<k20>, "Session out"=w479:refnum<k21>)  [unwired: 7 in]
        n260 = global read "SW_Globals_2.2+.vi" "All references"() -> (w490:T36)
        n261 = property class="System Filter"(reference=w502, error in=w503, "IsPresent"=w501, "IsChassis"=FALSE ("Is Chassis")) -> (reference out=w497:refnum<k20>, error out=w498:errorcluster)
        n262 = Unbundle By Name(w490) -> ("Indicators references.Port"=w488:refnum<vi>)
        n263 = Unbundle By Name(w476) -> ("Defaults.VISA Resource Name"=w475:string)
        n264 = call <vilib>:"Find Hardware.vi"("error in (no error)"=w498, "Experts"="ni-visa", "Filter in"=w497, "Session in"=w479) -> ("error out"=w494:errorcluster, "Resources out"=w495:refnum<k20>[], "Session out"=w492:refnum<k21>)  [unwired: 4 in, 1 out]
        n265 = for {
          tunnel: w495 -> [w518] mode=indexing
          tunnel: [w512] -> _ mode=indexing if=w511
          tunnel: w475 -> [w516]
          tunnel: [w515] -> w493 mode=indexing
          tunnel: [w514] -> w477 mode=indexing
          shift-right: [w509] -> w469
          shift-left: w494 -> [w517]
          n266 = property class="System Hardware"(reference=w518, error in=w517) -> (reference out=w515:refnum<k20>, error out=w508:errorcluster, "PortBinding"=w512:string, "Resource"=w514:string)
          n267 = Equal?(x=w514, y=w516) -> (x = y?=w513:bool)
          n268 = call <vilib>:"Clear Errors.vi"("error in (no error)"=w508, "specific error code to clear (0: all)"=-2147220623) -> ("error out"=w509:errorcluster, "specific error cleared?"=w506:bool)  [unwired: 4 in]
          n269 = Not(x=w506) -> (.not. x?=w510:bool)
          n270 = And(x=w513, y=w510) -> (x .and. y?=w511:bool)
        }
        n271 = Concatenate Strings(w489, w475) -> (w487:string)
        n272 = property class="Str"(reference=w488, "Value"=w487) -> ()  [unwired: 1 in, 2 out]
        n273 = local write "VISA Resources found"(w477) -> ()
        n274 = call-poly <vilib>:"Close.vi"("error in (no error)"=w469, "Resources in"=w493) -> ("error out"=w491:errorcluster)  [unwired: 9 in]
        n275 = call-poly <vilib>:"Close.vi"("error in (no error)"=w491, "Session in"=w492) -> ("error out"=w485:errorcluster)  [unwired: 9 in]
        n276 = Enqueue Element(queue=w483, element=CTL_Control_States."Save HW Settings", error in (no error)=w485) -> (queue out=w472:refnum<queue>, error out=w474:errorcluster)  [unwired: 1 in, 1 out]
        n277 = Enqueue Element(queue=w472, element=CTL_Control_States."Set I/O config (silent)", error in (no error)=w474) -> (queue out=w471:refnum<queue>, error out=w473:errorcluster)  [unwired: 1 in, 1 out]
        n278 = Enqueue Element(queue=w471, element=CTL_Control_States."Unlock UI (init OK)", error in (no error)=w473) -> (queue out=w482:refnum<queue>, error out=w481:errorcluster)  [unwired: 1 in, 1 out]
        n279 = call <vilib>:"Unset Busy.vi"("error in (no error)"=w481) -> ("error out"=w504:errorcluster)  [unwired: 10 in]
      }
      frame "Save HW Settings" {
        n280 = global read "SW_Globals_2.2+.vi" "Paths"() -> (w531:T77)
        n281 = Unbundle By Name(w531) -> ("Program settings"=w530:path)
        n282 = global read "SW_Globals_2.2+.vi" "Settings cluster"() -> (w519:T16)
        n283 = call <vilib>:"Open Config Data.vi"("error in (no error)"=w528, "create file if necessary (T)"=FALSE, "configuration file path"=w530) -> ("error out"=w526:errorcluster, "refnum"=w527:T78)  [unwired: 6 in, 1 out]
        n284 = local write "Settings cluster (local)"(w519) -> ()
        n285 = call "SW_Save_parameter_group_2.vi"("Researcher name"="Researcher", "error in"=w526, "Settings cluster in"=w519, "Parameter group"=T61 "Defaults", "Settings file refnum in"=w527) -> ("error out"=w525:errorcluster, "Settings file refnum out"=w524:T78)  [unwired: 4 in, 1 out]
        n286 = call <vilib>:"Close Config Data.vi"("error in (no error)"=w525, "refnum"=w524) -> ("error out"=w523:errorcluster)  [unwired: 8 in, 1 out]
      }
      frame "Unlock UI (init OK)" {
        n287 = global read "SW_Globals_2.2+.vi" "Settings cluster"() -> (w533:T16)
        n288 = global read "SW_Globals_2.2+.vi" "All references"() -> (w546:T36)
        n289 = local write "Settings cluster (local)"(w533) -> ()
        n290 = call "UI_(02)_Unlock.vi"("error in (no error)"=w547, "Settings cluster in"=w533, "All references in"=w546) -> ("error out"=w545:errorcluster)  [unwired: 2 out]
        n291 = Enqueue Element(queue=w544, element=CTL_Control_States."Zones layout update", error in (no error)=w545) -> (queue out=w541:refnum<queue>, error out=w542:errorcluster)  [unwired: 1 in, 1 out]
        n292 = Enqueue Element(queue=w541, element=CTL_Control_States."Upd. trace length", error in (no error)=w542) -> (queue out=w536:refnum<queue>, error out=w539:errorcluster)  [unwired: 1 in, 1 out]
        n293 = Enqueue Element(queue=w536, element=CTL_Control_States."Update filter", error in (no error)=w539) -> (queue out=w537:refnum<queue>, error out=w538:errorcluster)  [unwired: 1 in, 1 out]
      }
      frame "Switch to Offline mode" {
        n294 = Get Notifier Status(notifier=w559, error in (no error)=w558) -> (notifier out=w557:refnum<notifier>, current notification=w554:T46, error out=w556:errorcluster)  [unwired: 2 out]
        n295 = Bundle By Name(cluster=w554, "Offline mode"=TRUE) -> (w552:T46)
        n296 = Send Notification(notification=w552, notifier=w557, error in (no error)=w556) -> (notifier out=w555:refnum<notifier>, error out=w551:errorcluster)
        n297 = global read "SW_Globals_2.2+.vi" "Settings cluster"() -> (w548:T16)
        n298 = global read "SW_Globals_2.2+.vi" "All references"() -> (w549:T36)
        n299 = call "UI_(02B)_Switch_to_offline_mode.vi"("error in (no error)"=w551, "Settings cluster in"=w548, "All references in"=w549) -> ("error out"=w550:errorcluster)  [unwired: 5 in, 2 out]
      }
      frame "Switch to Online mode" {
        w561 = FALSE ("Offline mode")
        n300 = Get Notifier Status(notifier=w569, error in (no error)=w568) -> (notifier out=w567:refnum<notifier>, current notification=w563:T46, error out=w566:errorcluster)  [unwired: 2 out]
        n301 = Bundle By Name(cluster=w563, "Has been recorded"=w561, "Offline mode"=w561) -> (w562:T46)
        n302 = Send Notification(notification=w562, notifier=w567, error in (no error)=w566) -> (notifier out=w564:refnum<notifier>, error out=w565:errorcluster)
      }
      frame "Re-check HW (init failed)" {
        w582 = enum32{"Settings", "Recording and Analysis"}."Settings" ("Value")
        n303 = global read "SW_Globals_2.2+.vi" "All references"() -> (w593:T36)
        n304 = Unbundle By Name(w593) -> ("Controls references.Set/Rec and Analyse Tab"=w583:refnum<vi>, "Indicators references.Ready"=w590:refnum<vi>, "Controls references.Check HW connection"=w589:refnum<vi>)
        n305 = property class="TabCtl (strict)"(reference=w583, error in=w579, "Value"=w582) -> (error out=w576:errorcluster, "Pages"=w580:refnum<vi>[])  [unwired: 1 out]
        n306 = To Long Integer(number=w582) -> (32bit integer=w581:i32)
        n307 = Index Array(array=w580, index=w581) -> (element=w578:refnum<vi>)
        n308 = property class="Page"(reference=w578, error in=w576, "PageEnb"=T62."Page Enabled" ("Page Enabled State")) -> (error out=w575:errorcluster)  [unwired: 1 out]
        n309 = property class="Bool (strict)"(reference=w589, error in=w575, "DisabledEnum"=T63."Enabled" ("Disabled")) -> (error out=w587:errorcluster)  [unwired: 1 out]
        n310 = property class="Bool (strict)"(reference=w590, error in=w587, "Value"=FALSE, "Colors [4]"=T60 [{"Numeric Control"=16749459, "Numeric Control"=16749459}, {"Numeric Control"=1988894, "Numeric Control"=3381555}, {"Numeric Control"=4934475, "Numeric Control"=7895160}, {"Numeric Control"=994319, "Numeric Control"=1657881}]) -> (error out=w572:errorcluster)  [unwired: 1 out]
        n311 = flat-sequence {
          tunnel: [w595] -> w573
          tunnel: w572 -> [w594]
          tunnel: [w594] -> w571
          frame #0 {
            n312 = call <vilib>:"Three Button Dialog.vi"("Allow user to close window? (TRUE)"=FALSE, "Window Title (\"\")"="Connection error" ("Window Title (\"\")"), "Right Button Text (\"Cancel\")"="Offline mode" ("Right Button Text (\"Cancel\")"), "Center Button Text (\"No\")"="Adjust Settings" ("Center Button Text (\"No\")"), "Left Button Text (\"Yes\")"="Retry" ("Left Button Text (\"Yes\")"), "message"="Cannot connect to hardware!") -> ("Which Button?"=w595:T79)  [unwired: 5 in]
          }
        }
        n313 = case shown="\"Right Button\"" w573 {
          tunnel: w586 -> [w606 w611 w616]
          tunnel: [w605 w610 w615] -> w585
          tunnel: w571 -> [w604 w609 w614]
          tunnel: [w603 w608 w613] -> w584
          frame "Left Button", Default {
            # "Re-check automatically"
            n314 = Enqueue Element(queue=w606, element=CTL_Control_States."HW Init", error in (no error)=w604) -> (queue out=w605:refnum<queue>, error out=w603:errorcluster)  [unwired: 1 in, 1 out]
          }
          frame "Center Button" {
            # "Pop-up manual port adjustment dialog"
            n315 = Enqueue Element(queue=w611, element=CTL_Control_States."Configure port(s)", error in (no error)=w609) -> (queue out=w610:refnum<queue>, error out=w608:errorcluster)  [unwired: 1 in, 1 out]
          }
          frame "Right Button" {
            # "Switch to offline mode"
            n316 = Enqueue Element(queue=w616, element=CTL_Control_States."Switch to Offline mode", error in (no error)=w614) -> (queue out=w615:refnum<queue>, error out=w613:errorcluster)  [unwired: 1 in, 1 out]
          }
        }
      }
      frame "Configure port(s)" {
        w630 = enum32{"Settings", "Recording and Analysis"}."Settings" ("Value")
        n317 = global read "SW_Globals_2.2+.vi" "All references"() -> (w641:T36)
        n318 = Unbundle By Name(w641) -> ("Controls references.Set/Rec and Analyse Tab"=w631:refnum<vi>, "Indicators references.Ready"=w638:refnum<vi>, "Controls references.Check HW connection"=w637:refnum<vi>)
        n319 = property class="TabCtl (strict)"(reference=w631, error in=w627, "Value"=w630) -> (error out=w624:errorcluster, "Pages"=w628:refnum<vi>[])  [unwired: 1 out]
        n320 = To Long Integer(number=w630) -> (32bit integer=w629:i32)
        n321 = Index Array(array=w628, index=w629) -> (element=w626:refnum<vi>)
        n322 = property class="Page"(reference=w626, error in=w624, "PageEnb"=T62."Page Enabled" ("Page Enabled State")) -> (error out=w623:errorcluster)  [unwired: 1 out]
        n323 = property class="Bool (strict)"(reference=w637, error in=w623, "DisabledEnum"=T63."Enabled" ("Disabled")) -> (error out=w635:errorcluster)  [unwired: 1 out]
        n324 = global read "SW_Globals_2.2+.vi" "Settings cluster"() -> (w619:T16)
        n325 = property class="Bool (strict)"(reference=w638, error in=w635, "Value"=FALSE, "Colors [4]"=T60 [{"Numeric Control"=16749459, "Numeric Control"=16749459}, {"Numeric Control"=1988894, "Numeric Control"=3381555}, {"Numeric Control"=4934475, "Numeric Control"=7895160}, {"Numeric Control"=994319, "Numeric Control"=1657881}]) -> (error out=w621:errorcluster)  [unwired: 1 out]
        n326 = call "HW_Configure_port(s).vi"("Settings cluster in"=w619, "error in (no error)"=w621) -> ("Settings cluster out"=w617:T16, "error out"=w620:errorcluster)  [unwired: 1 out]
        n327 = global write "SW_Globals_2.2+.vi" "Settings cluster"(w617) -> ()
        n328 = local write "Settings cluster (local)"(w617) -> ()
        n329 = Enqueue Element(queue=w634, element=CTL_Control_States."HW Init", error in (no error)=w620) -> (queue out=w633:refnum<queue>, error out=w632:errorcluster)  [unwired: 1 in, 1 out]
      }
      frame "Update filter" {
        (unwired) dbl[] [] ("Reverse coefficients")
        w645 = 11 ("half-width")
        n330 = global read "SW_Globals_2.2+.vi" "Settings cluster"() -> (w662:T16)
        n331 = local read "Calibration parameters"() -> (w658:T23)
        n332 = Unbundle By Name(w662) -> ()  [unwired: 1 out]
        n333 = Unbundle By Name(w658) -> ("True FPS"=w651:dbl)
        n334 = Greater Than 0?(x=w651) -> (x > 0?=w650:bool)
        n335 = local read "FPS status"() -> (w649:i32)
        n336 = Select(t=w651, s=w650, f=w649) -> (s? t:f=w648:dbl)
        n337 = local read "Pre-filter params."() -> (w656:T28)
        n338 = Reciprocal(x=w648) -> (1/x=w647:dbl)
        n339 = call <vilib>:"Smoothing Filter Coefficients.vi"("fs"=w648, "time constant"=0.1, "shape"=enum16{"rectangular", "triangular"}."rectangular", "half-width"=w645, "type"=enum16{"moving average", "exponential"}."exponential") -> ("forward coefficients"=w652:dbl[], "reverse coefficients"=w653:dbl[])  [unwired: 4 in, 1 out]
        n340 = call "SW_SG_coefficients.vi"("Filter parameters"=T17 {"Filter type"=enum."Savitzky-Golay", "Length"=23, "Order"=3}) -> ()  [unwired: 2 in, 1 out]
        n341 = Multiply(x=w645, y=2) -> (x*y=w643:i32)
        n342 = Increment(x=w643) -> (x+1=w642:i32)
        n343 = Bundle(cluster=w656, "Reverse coefficients"=w653, "Forward coefficients"=w652, "Full filter length (info only)"=w642, "Type"=enum16{"None", "FIR (PtbyPt)", "IIR (PtbyPt)"}."IIR (PtbyPt)") -> (w655:T28)
        n344 = local write "Act. frame time, s"(w647) -> ()
        n345 = local write "Pre-filter params."(w655) -> ()
      }
      frame "Zones layout update" {
        n346 = global read "SW_Globals_2.2+.vi" "All references"() -> (w706:T36)
        n347 = local read "Settings cluster (local)"() -> (w708:T16)
        n348 = Unbundle By Name(w706) -> ("Indicators references.Current zone"=w705:refnum<vi>)
        n349 = Get Notifier Status(notifier=w710, error in (no error)=w701) -> (notifier out=w698:refnum<notifier>, current notification=w700:T46, error out=w696:errorcluster)  [unwired: 2 out]
        n350 = Unbundle By Name(w706) -> ("Controls references.Show zones"=w717:refnum<vi>, "Controls references.Show magnets"=w716:refnum<vi>)
        n351 = Unbundle By Name(w708) -> ("Geometry"=w678:T19)
        n352 = Bundle By Name(cluster=w700, "Updating layout"=TRUE) -> (w697:T46)
        n353 = call "SW_Check_segments_parameters_2.vi"("Geometry in"=w678) -> ("Error Out"=w676:errorcluster, "Segmentation out"=w707:T14, "Geometry out"=w665:T19)  [unwired: 2 in]
        n354 = property class="Bool (strict)"(reference=w717) -> ("Value"=w671:bool)  [unwired: 1 in, 2 out]
        n355 = Select(t=T63."Disabled and Grayed Out" ("Disabled"), s=w671, f=T63."Enabled" ("Disabled")) -> (s? t:f=w713:T63)
        n356 = property class="Bool (strict)"(reference=w716, "DisabledEnum"=w713) -> ("Value"=w670:bool)  [unwired: 1 in, 2 out]
        n357 = Send Notification(notification=w697, notifier=w698, error in (no error)=w696) -> (notifier out=w691:refnum<notifier>, error out=w686:errorcluster)
        n358 = local write "Cage radial segmentation"(w707) -> ()
        n359 = call "2 ms delay"("error in (no error)"=w686) -> ("error out"=w675:errorcluster)  [unwired: 10 in]
        n360 = Merge Errors(w676, w675) -> (w677:errorcluster)
        n361 = call "UI_update_Zone_indicator_params_(univ).vi"("error in (no error)"=w677, "Geometry"=w678, "Zone indicator ref. in"=w705) -> ("error out"=w704:errorcluster)  [unwired: 7 in, 1 out]
        n362 = Bundle("Geometry out"=w665, "Value"=w671, "Value"=w670) -> (w668:T80)  [unwired: 1 in]
        n363 = call "New Layout (instant).vi"("error in (no error)"=w675, "Cage parameters"=w668) -> ("Reply Payload"=w674:T71)  [unwired: 7 in, 2 out]
        n364 = Unbundle By Name(w674) -> ("Cage Diagram ref"=w673:T15, "Pixel <> Zone"=w672:T3, "Cage drawing parameters out.Image Scaling info.Pixels per mm"=w666:dbl, "New Layout (instant)_error"=w667:errorcluster)
        n365 = local read "Speed threshold"() -> (w680:dbl)
        n366 = Not(x=w671) -> (.not. x?=w711:bool)
        n367 = local write "Diagram (generated)"(w673) -> ()
        n368 = disable-structure shown="Disabled" {
          disable-tunnel: [w718 _] -> _
          frame Disabled {
            n369 = call "SW_Generate_Segmented_Plot_v4_DAQmx.vi"() -> ("Image geometrical and scaling parameters"=w719:T30)  [unwired: 9 in, 6 out]
            n370 = local write "Img geom and scaling"(w719) -> ()
            n371 = Unbundle By Name(w719) -> ("Pixels per mm"=w718:dbl)
          }
          frame Enabled {
          }
        }
        n372 = local write "Bright mouse lineout"(w711) -> ()
        n373 = Bundle By Name(cluster=T4 {"max"=300.0, "min"=0.0, "# bins"=10, "threshold"=8.0, "thr. type"=enum."higher accepted"} ("Histogram parameters"), "threshold"=w680) -> (w679:T4)
        n374 = Bundle By Name(cluster=w708, "Geometry"=w665, "Defaults.Histogram parameters"=w679) -> (w669:T16)
        n375 = local write "Settings cluster (local)"(w669) -> ()
        n376 = global write "SW_Globals_2.2+.vi" "Settings cluster"(w669) -> ()
        n377 = local write "Pixel to zone"(w672) -> ()
        n378 = local read "Stats parameters (online)"() -> (w685:T1)
        n379 = local read "Mouse drawing parameters"() -> (w712:T2)
        n380 = Merge Errors(w667, w704) -> (w702:errorcluster)
        n381 = Bundle By Name(cluster=w712, "Bright mouse lineout"=w711, "Pixels per mm"=w666) -> (w684:T2)
        n382 = call "GEN_Histo_Bins_And_X_axis.vi"("Error In"=w702, "Histogram parameters"=w679) -> ("Error Out"=w690:errorcluster, "Bins"=w683:dbl[], "X axis values"=w703:dbl[])  [unwired: 6 in, 1 out]
        n383 = Bundle By Name(cluster=w685, "Mouse drawing parameters"=w684, "Array of the pixel to zone correspondences"=w672, "Hist. bins array"=w683, "Histogram parameters"=w679) -> (w682:T1)
        n384 = Get Notifier Status(notifier=w691, error in (no error)=w690) -> (notifier out=w688:refnum<notifier>, current notification=w687:T46, error out=w689:errorcluster)  [unwired: 2 out]
        n385 = local write "Mouse drawing parameters"(w684) -> ()
        n386 = Bundle By Name(cluster=w687, "Updating layout"=FALSE) -> (w692:T46)
        n387 = local write "Hist. X axis"(w703) -> ()
        n388 = local write "Stats parameters (online)"(w682) -> ()
        n389 = Send Notification(notification=w692, notifier=w688, error in (no error)=w689) -> (notifier out=w694:refnum<notifier>, error out=w695:errorcluster)
      }
      frame "Set I/O config" {
        n390 = global read "SW_Globals_2.2+.vi" "Settings cluster"() -> (w729:T16)
        n391 = global read "SW_Globals_2.2+.vi" "All references"() -> (w739:T36)
        n392 = Unbundle By Name(w729) -> ("Defaults.VISA Resource Name"=w735:string, "IO parameters"=w740:T22, "IO parameters.Sync capability"=w731:u8)
        n393 = Unbundle By Name(w739) -> ("Indicators references.IO status indicator"=w738:refnum<vi>)
        n394 = call "HW_set_IO_ports_3-pos_2.vi"("IO parameters cluster"=w740) -> ("IO parameters cluster output"=w721:T22, "IO changed"=w728:bool)
        n395 = call "SW_get_IO_ports_representation_2.vi"("Sync parameters cluster input"=w721) -> ("IO status indicator"=w737:T39)
        n396 = call "SW_get_config_of_Zones_and_IO_2.vi"("Sync parameters cluster input"=w721) -> ("Ports IO config (OUT is FALSE)"=w722:bool[], "IO inversion config."=w734:u16)  [unwired: 2 out]
        n397 = property class="Clust"(reference=w738, error in=w736, "Value"=w737) -> (error out=w733:errorcluster)  [unwired: 1 out]
        n398 = local write "Ports IO config"(w722) -> ()
        n399 = Bundle By Name(cluster=w729, "IO parameters"=w721) -> (w720:T16)
        n400 = call "HW_Set_IO_Dir_on_ECU.vi"("Error In"=w733, "IO ports config"=w722, "VISA resource name"=w735, "IO inversion config."=w734) -> ("error out"=w730:errorcluster, "VISA resource name out"=w732:refnum<visa-resource-name>)
        n401 = local write "IO parameters"(w721) -> ()
        n402 = case shown="1.." w731 {
          tunnel: w732 -> [_ w757]
          tunnel: w730 -> [w748 w756]
          tunnel: w721 -> [_ w755]
          tunnel: [w748 w751] -> w725
          frame 0, Default {
          }
          frame 1.. {
            w752 = u16 4
            n403 = Unbundle By Name(w755) -> ("IO 1 configuration"=w754:u16, "IO 2 configuration"=w753:u16)
            n404 = Equal?(x=w754, y=w752) -> (x = y?=w750:bool)
            n405 = Equal?(x=w753, y=w752) -> (x = y?=w749:bool)
            n406 = call "HW_Set_SYNC_Status.vi"("error in (no error)"=w756, "SYNC 2"=w750, "SYNC 1"=w749, "VISA Resource name IN"=w757) -> ("error out"=w751:errorcluster)  [unwired: 6 in, 1 out]
          }
        }
        n407 = local write "Settings cluster (local)"(w720) -> ()
        n408 = global write "SW_Globals_2.2+.vi" "Settings cluster"(w720) -> ()
        n409 = case shown="True" w728 {
          tunnel: w727 -> [w742 w743]
          tunnel: [w742 w745] -> w726
          tunnel: w725 -> [w741 w747]
          tunnel: [w741 w744] -> w724
          frame False {
            # "IO not changed"
          }
          frame True {
            # "IO changed"
            n410 = Enqueue Element(queue=w743, element=CTL_Control_States."Save all settings", error in (no error)=w747) -> (queue out=w745:refnum<queue>, error out=w744:errorcluster)  [unwired: 1 in, 1 out]
          }
        }
      }
      frame "Set I/O config (silent)" {
        n411 = global read "SW_Globals_2.2+.vi" "Settings cluster"() -> (w764:T16)
        n412 = global read "SW_Globals_2.2+.vi" "All references"() -> (w774:T36)
        n413 = Unbundle By Name(w764) -> ("Defaults.VISA Resource Name"=w770:string, "IO parameters"=w760:T22, "IO parameters.Sync capability"=w766:u8)
        n414 = Unbundle By Name(w774) -> ("Indicators references.IO status indicator"=w773:refnum<vi>)
        n415 = call "SW_get_IO_ports_representation_2.vi"("Sync parameters cluster input"=w760) -> ("IO status indicator"=w772:T39)
        n416 = call "SW_get_config_of_Zones_and_IO_2.vi"("Sync parameters cluster input"=w760) -> ("Ports IO config (OUT is FALSE)"=w762:bool[], "IO inversion config."=w769:u16)  [unwired: 2 out]
        n417 = property class="Clust"(reference=w773, error in=w771, "Value"=w772) -> (error out=w768:errorcluster)  [unwired: 1 out]
        n418 = local write "Ports IO config"(w762) -> ()
        n419 = Bundle By Name(cluster=w764, "IO parameters"=w760) -> (w761:T16)
        n420 = call "HW_Set_IO_Dir_on_ECU.vi"("Error In"=w768, "IO ports config"=w762, "VISA resource name"=w770, "IO inversion config."=w769) -> ("error out"=w765:errorcluster, "VISA resource name out"=w767:refnum<visa-resource-name>)
        n421 = local write "IO parameters"(w760) -> ()
        n422 = case shown="1.." w766 {
          tunnel: w767 -> [_ w784]
          tunnel: w765 -> [w775 w783]
          tunnel: w760 -> [_ w782]
          tunnel: [w775 w778] -> w758
          frame 0, Default {
          }
          frame 1.. {
            w779 = u16 4
            n423 = Unbundle By Name(w782) -> ("IO 1 configuration"=w781:u16, "IO 2 configuration"=w780:u16)
            n424 = Equal?(x=w781, y=w779) -> (x = y?=w777:bool)
            n425 = Equal?(x=w780, y=w779) -> (x = y?=w776:bool)
            n426 = call "HW_Set_SYNC_Status.vi"("error in (no error)"=w783, "SYNC 2"=w777, "SYNC 1"=w776, "VISA Resource name IN"=w784) -> ("error out"=w778:errorcluster)  [unwired: 6 in, 1 out]
          }
        }
        n427 = local write "Settings cluster (local)"(w761) -> ()
        n428 = global write "SW_Globals_2.2+.vi" "Settings cluster"(w761) -> ()
      }
      frame "Cage and recording settings" {
        n429 = global read "SW_Globals_2.2+.vi" "Paths"() -> (w794:T77)
        n430 = call "SW_Set_Cage_and_Recording_Settings.vi"("error in (no error)"=w805) -> ("Update FPS?"=w797:bool, "Save Config?"=w785:bool, "error out"=w796:errorcluster)  [unwired: 1 in]
        n431 = global read "SW_Globals_2.2+.vi" "Settings cluster"() -> (w792:T16)
        n432 = call "SW_Get_Save_Paths_2.vi"("Settings cluster in"=w792, "Paths in"=w794, "error in (no error)"=w796) -> ("Paths out"=w793:T77, "error out"=w795:errorcluster)  [unwired: 2 in, 2 out]
        n433 = global write "SW_Globals_2.2+.vi" "Paths"(w793) -> ()
        n434 = case shown="True" w797 {
          tunnel: w795 -> [w813 w822]
          tunnel: [w813 w821] -> w787
          tunnel: w798 -> [w814 w820]
          tunnel: [w814 w819] -> w789
          frame False {
          }
          frame True {
            n435 = Enqueue Element(queue=w820, element=CTL_Control_States."Play Stop", error in (no error)=w822) -> (queue out=w816:refnum<queue>, error out=w817:errorcluster)  [unwired: 1 in, 1 out]
            n436 = Enqueue Element(queue=w816, element=CTL_Control_States."Upd. FPS", error in (no error)=w817) -> (queue out=w819:refnum<queue>, error out=w821:errorcluster)  [unwired: 1 in, 1 out]
          }
        }
        n437 = case shown="True" w785 {
          tunnel: w789 -> [w807 w810]
          tunnel: [w807 w809] -> w788
          tunnel: w787 -> [w806 w811]
          tunnel: [w806 w808] -> w786
          frame False {
          }
          frame True {
            n438 = Enqueue Element(queue=w810, element=CTL_Control_States."Save all settings", error in (no error)=w811) -> (queue out=w809:refnum<queue>, error out=w808:errorcluster)  [unwired: 1 in, 1 out]
          }
        }
        n439 = flat-sequence {
          tunnel: w786 -> [w825]
          tunnel: [w832] -> w790
          frame #0 {
            n440 = global read "SW_Globals_2.2+.vi" "Settings cluster"() -> (w831:T16)
            n441 = Unbundle By Name(w831) -> ("Geometry"=w830:T19)
            n442 = global read "SW_Globals_2.2+.vi" "All references"() -> (w835:T36)
            n443 = Unbundle By Name(w835) -> ("Indicators references.Cage size"=w834:refnum<vi>)
            n444 = call "SW_Read_Cage's_Geometrical_Parameter.vi"("Error In"=w825, "Parameter to read"=enum16{"None", "Cage diameter/size"}."Cage diameter/size", "Geometry in"=w830) -> ("Error Out"=w826:errorcluster, "Parameter value"=w828:variant)  [unwired: 6 in, 1 out]
            n445 = local write "Settings cluster (local)"(w831) -> ()
            n446 = Variant To Data(error in=w826, type=u16 0, Variant=w828) -> (data=w827:u16, error out=w824:errorcluster)
            n447 = Number To Decimal String(number=w827) -> (decimal integer string=w837:string)  [unwired: 1 in]
            n448 = Concatenate Strings(w837, " mm cage" ("string")) -> (w833:string)
            n449 = property class="Str"(reference=w834, error in=w824, "Value"=w833) -> (error out=w832:errorcluster)  [unwired: 1 out]
          }
        }
        n450 = Enqueue Element(queue=w788, element=CTL_Control_States."Zones layout update", error in (no error)=w790) -> (queue out=w802:refnum<queue>, error out=w804:errorcluster)  [unwired: 1 in, 1 out]
        n451 = Enqueue Element(queue=w802, element=CTL_Control_States."Update filter", error in (no error)=w804) -> (queue out=w803:refnum<queue>, error out=w791:errorcluster)  [unwired: 1 in, 1 out]
      }
      frame "Play Start" {
        n452 = Get Notifier Status(notifier=w846, error in (no error)=w845) -> (notifier out=w843:refnum<notifier>, current notification=w842:T46, error out=w847:errorcluster)  [unwired: 2 out]
        n453 = Unbundle By Name(w842) -> ("Data loaded"=w838:bool, "Offline mode"=w839:bool)
        n454 = case shown="False" w839 {
          tunnel: w847 -> [w859 w868]
          tunnel: [w853 w869] -> w840
          tunnel: w843 -> [w863 w866]
          tunnel: w842 -> [w862 _]
          tunnel: [w851 w865] -> w841
          tunnel: w838 -> [_ w867]
          frame False {
            # "This part is running when working online"
            n455 = global read "SW_Globals_2.2+.vi" "Settings cluster"() -> (w849:T16)
            n456 = Unbundle By Name(w849) -> ("Defaults.VISA Resource Name"=w860:string)
            n457 = call "HW_Acquisition_Start.vi"("Error In"=w859, "VISA resource name in"=w860) -> ("Error Out"=w856:errorcluster)  [unwired: 1 out]
            n458 = call "Set Parameters and data.vi"("Data"=w849, "Parameter"=CTL_Parameter_transfer_name."All parameters") -> ()  [unwired: 9 in, 1 out]
            n459 = global read "SW_Globals_2.2+.vi" "All references"() -> (w852:T36)
            n460 = Unbundle By Name(w852) -> ("Controls references.Play/Pause"=w858:refnum<vi>)
            n461 = property class="Bool (strict)"(reference=w858, error in=w856, "Value"=TRUE) -> (error out=w855:errorcluster)  [unwired: 1 out]
            n462 = Bundle By Name(cluster=w862, "Acq. is ON"=TRUE ("\"Play\" is ON")) -> (w861:T46)
            n463 = Send Notification(notification=w861, notifier=w863, error in (no error)=w855) -> (notifier out=w851:refnum<notifier>, error out=w854:errorcluster)
            n464 = call "UI_(03A)_Set_Play_State.vi"("error in (no error)"=w854, "Settings cluster in"=w849, "All references in"=w852) -> ("error out"=w853:errorcluster)  [unwired: 2 out]
            n465 = Get Date/Time In Seconds() -> (seconds since 1Jan1904=w850:timestamp)
            n466 = local write "Start time (SW)"(w850) -> ()
          }
          frame True {
            # "This part is running when working offline"
            n467 = case shown="True" w867 {
              tunnel: [w871 w880] -> w869
              tunnel: w868 -> [w871 w878]
              tunnel: w866 -> [w870 w876]
              tunnel: [w870 w876] -> w865
              frame False {
              }
              frame True {
                w872 = TRUE ("Value")
                n468 = local read "Settings cluster (local)"() -> (w877:T16)
                n469 = global read "SW_Globals_2.2+.vi" "All references"() -> (w879:T36)
                n470 = Unbundle By Name(w879) -> ("Controls references.Play/Pause"=w881:refnum<vi>, "Controls references.Reset barplot"=w875:refnum<vi>)
                n471 = property class="Bool (strict)"(reference=w881, error in=w878, "Value"=w872) -> (error out=w874:errorcluster)  [unwired: 1 out]
                n472 = property class="Bool (strict)"(reference=w875, error in=w874, "Val(Sgnl)"=w872) -> (error out=w873:errorcluster)  [unwired: 1 out]
                n473 = call "UI_(07A)_Set_Play_State_(offline).vi"("error in (no error)"=w873, "Settings cluster in"=w877, "All references in"=w879) -> ("error out"=w880:errorcluster)  [unwired: 2 out]
              }
            }
          }
        }
      }
      frame "Play Stop" {
        n474 = Get Notifier Status(notifier=w892, error in (no error)=w891) -> (notifier out=w888:refnum<notifier>, current notification=w887:T46, error out=w893:errorcluster)  [unwired: 2 out]
        n475 = Unbundle By Name(w887) -> ("Acq. is ON"=w884:bool, "Offline mode"=w886:bool)
        n476 = Not(x=w886) -> (.not. x?=w882:bool)
        n477 = And(x=w884, y=w882) -> (x .and. y?=w883:bool)
        n478 = case shown="True" w883 {
          tunnel: w893 -> [w898 w909]
          tunnel: [w894 w903] -> w889
          tunnel: w888 -> [w899 w913]
          tunnel: w887 -> [_ w912]
          tunnel: [w899 w901] -> w885
          frame False {
            w895 = T63."Enabled" ("Disabled")
            # "This part is running when working with the recorded data"
            n479 = property on="Timeline" class="Slide (strict)"(error in=w898, "DisabledEnum"=w895) -> (error out=w897:errorcluster)  [unwired: 1 in, 1 out]
            n480 = property on="Open File" class="Bool (strict)"(error in=w897, "DisabledEnum"=w895) -> (error out=w896:errorcluster)  [unwired: 1 in, 1 out]
            n481 = property on="Start over" class="Bool (strict)"(error in=w896, "DisabledEnum"=w895) -> (error out=w894:errorcluster)  [unwired: 1 in, 1 out]
          }
          frame True {
            # "This part is running when working online"
            n482 = Bundle By Name(cluster=w912, "Acq. is ON"=FALSE ("\"Play\" is ON")) -> (w911:T46)
            n483 = global read "SW_Globals_2.2+.vi" "Settings cluster"() -> (w900:T16)
            n484 = Send Notification(notification=w911, notifier=w913, error in (no error)=w909) -> (notifier out=w901:refnum<notifier>, error out=w908:errorcluster)
            n485 = Unbundle By Name(w900) -> ("Defaults.VISA Resource Name"=w910:string)
            n486 = call "HW_Acquisition_Stop.vi"("Error In"=w908, "VISA resource name in"=w910) -> ("Error Out"=w905:errorcluster)  [unwired: 1 out]
            n487 = global read "SW_Globals_2.2+.vi" "All references"() -> (w902:T36)
            n488 = Unbundle By Name(w902) -> ("Controls references.Play/Pause"=w907:refnum<vi>)
            n489 = property class="Bool (strict)"(reference=w907, error in=w905, "Value"=FALSE) -> (error out=w904:errorcluster)  [unwired: 1 out]
            n490 = call "UI_(04A)_Set_Stop_State.vi"("error in (no error)"=w904, "Settings cluster in"=w900, "All references in"=w902) -> ("error out"=w903:errorcluster)  [unwired: 2 out]
          }
        }
      }
      frame "Start Recording" {
        n491 = Get Notifier Status(notifier=w922, error in (no error)=w921) -> (notifier out=w919:refnum<notifier>, current notification=w918:T46, error out=w923:errorcluster)  [unwired: 2 out]
        n492 = Unbundle By Name(w918) -> ("Offline mode"=w917:bool)
        n493 = case shown="False" w917 {
          tunnel: w923 -> [w935 w960]
          tunnel: [w944 w960] -> w915
          tunnel: w919 -> [w954 w959]
          tunnel: w918 -> [w955 _]
          tunnel: [w943 w959] -> w916
          frame False {
            # "This part is running when working online"
            n494 = global read "SW_Globals_2.2+.vi" "Settings cluster"() -> (w938:T16)
            n495 = global read "SW_Globals_2.2+.vi" "All references"() -> (w937:T36)
            n496 = Unbundle By Name(w937) -> ("Controls references.Reset barplot"=w936:refnum<vi>)
            n497 = local read "TTL in time (HW)"() -> (w939:u32)
            n498 = local read "TTL in time (SW)"() -> (w942:timestamp)
            n499 = global read "SW_Globals_2.2+.vi" "Paths"() -> (w952:T77)
            n500 = call "UI_(05A)_Set_Record_Start_State.vi"("error in (no error)"=w935, "Settings cluster in"=w938, "All references in"=w937) -> ("error out"=w953:errorcluster, "Settings cluster out"=w951:T16)  [unwired: 1 out]
            n501 = property class="Bool (strict)"(reference=w936, error in=w935, "Val(Sgnl)"=TRUE ("Value (Signaling)")) -> (error out=w933:errorcluster)  [unwired: 1 out]
            n502 = local write "Start time (HW)"(w939) -> ()
            n503 = local write "Frame #"(u32 0 ("Frame #")) -> ()
            n504 = call "SW_Get_Save_Paths_2.vi"("Settings cluster in"=w951, "Paths in"=w952, "Time stamp in"=w942, "error in (no error)"=w953) -> ("Settings cluster out"=w947:T16, "Paths out"=w948:T77, "Time stamp out"=w949:timestamp, "error out"=w950:errorcluster)  [unwired: 1 in]
            n505 = call "PR_Prepare_TDMS_for_Recording.vi"("Buffer size, samples"=400, "error in (no error)"=w950, "Time Stamp in"=w949, "Paths in"=w948, "Settings cluster"=w947) -> ("error out"=w945:errorcluster, "Time Stamp out"=w946:timestamp, "Paths out"=w941:T77, "Settings cluster out"=w929:T16)  [unwired: 3 in]
            n506 = Unbundle By Name(w929) -> ("Defaults.VISA Resource Name"=w928:string, "IO parameters"=w926:T22)
            n507 = local write "Start time (SW)"(w946) -> ()
            n508 = global write "SW_Globals_2.2+.vi" "Settings cluster"(w929) -> ()
            n509 = local write "Settings cluster (local)"(w929) -> ()
            n510 = Unbundle By Name(w941) -> ("TDMS file reference"=w940:refnum<k34>)
            n511 = Merge Errors(w945, w933) -> (w931:errorcluster)
            n512 = Bundle By Name(cluster=w955, "Recording now"=TRUE, "Has been recorded"=FALSE) -> (w957:T46)
            n513 = global write "SW_Globals_2.2+.vi" "Paths"(w941) -> ()
            n514 = call "SW_Fire_TTL_on_start_or_stop.vi"("TTL pulse length, ms"=25.0, "error in (no error)"=w931, "Serial Port In"=w928, "Flush receive buffer?"=TRUE, "IO parameters cluster in"=w926) -> ("error out"=w930:errorcluster)  [unwired: 4 in, 2 out]
            n515 = local write "TDMS ref."(w940) -> ()
            n516 = Send Notification(notification=w957, notifier=w954, error in (no error)=w930) -> (notifier out=w943:refnum<notifier>, error out=w944:errorcluster)
          }
          frame True {
            # "This part is running when working with the recorded data"
          }
        }
      }
      frame "Stop Recording" {
        n517 = Get Notifier Status(notifier=w969, error in (no error)=w968) -> (notifier out=w967:refnum<notifier>, current notification=w966:T46, error out=w970:errorcluster)  [unwired: 2 out]
        n518 = Unbundle By Name(w966) -> ("Offline mode"=w965:bool)
        n519 = case shown="False" w965 {
          tunnel: w970 -> [w971 w1000]
          tunnel: [w982 w1000] -> w961
          tunnel: w967 -> [w997 w999]
          tunnel: w966 -> [w996 _]
          tunnel: [w995 w999] -> w964
          tunnel: w963 -> [w985 w998]
          tunnel: [w983 w998] -> w962
          frame False {
            # "This part is running when working online"
            n520 = Bundle By Name(cluster=w996, "Acq. is ON"=FALSE, "Recording now"=FALSE, "Has been recorded"=FALSE) -> (w993:T46)
            n521 = global read "SW_Globals_2.2+.vi" "Settings cluster"() -> (w979:T16)
            n522 = Unbundle By Name(w979) -> ("Defaults.VISA Resource Name"=w975:string, "IO parameters"=w974:T22)
            n523 = call "SW_Fire_TTL_on_start_or_stop.vi"("TTL pulse length, ms"=50.0, "error in (no error)"=w971, "Serial Port In"=w975, "Flush receive buffer?"=FALSE, "IO parameters cluster in"=w974) -> ("error out"=w972:errorcluster, "Serial Port Out"=w976:refnum<visa-resource-name>)  [unwired: 4 in, 1 out]
            n524 = global read "SW_Globals_2.2+.vi" "All references"() -> (w991:T36)
            n525 = Send Notification(notification=w993, notifier=w997, error in (no error)=w972) -> (notifier out=w995:refnum<notifier>, error out=w973:errorcluster)
            n526 = call "HW_Acquisition_Stop.vi"("Error In"=w973, "VISA resource name in"=w976) -> ("Error Out"=w980:errorcluster)  [unwired: 1 out]
            n527 = local read "TDMS ref."() -> (w987:refnum<k34>)
            n528 = call "UI_(06A)_Set_Record_Stop_State.vi"("error in (no error)"=w980, "Settings cluster in"=w979, "All references in"=w991) -> ("error out"=w990:errorcluster)  [unwired: 2 out]
            n529 = TDMS Flush(4:w990, 7:w987) -> (0:w989:errorcluster, 3:w986:refnum<k34>)
            n530 = TDMS Close(8:w989, 11:w986) -> (0:w988:errorcluster)  [unwired: 1 out]
            n531 = Enqueue Element(queue=w985, element=CTL_Control_States."Recording post-processing", error in (no error)=w988) -> (queue out=w983:refnum<queue>, error out=w982:errorcluster)  [unwired: 1 in, 1 out]
          }
          frame True {
            # "This part is running when working with the recorded data"
          }
        }
      }
      frame "Start over" {
        n532 = Two Button Dialog(message="Do you really want to start over? All unsaved changes will be lost!", 1:"No" ("F button name (\"Cancel\")"), 2:"Yes" ("T button name (\"OK\")")) -> (T button?=w1007:bool)
        n533 = case shown="True" w1007 {
          tunnel: [w1012 w1026] -> w1010
          tunnel: w1009 -> [w1012 w1022]
          tunnel: w1006 -> [w1013 w1021]
          tunnel: [w1013 w1015] -> w1008
          tunnel: [w1011 w1014] -> w1002
          tunnel: w1001 -> [w1011 w1014]
          frame False {
          }
          frame True {
            n534 = Enqueue Element(queue=w1022, element=CTL_Control_States."Switch to Online mode", error in (no error)=w1021) -> (queue out=w1023:refnum<queue>, error out=w1024:errorcluster)  [unwired: 1 in, 1 out]
            n535 = Enqueue Element(queue=w1023, element=CTL_Control_States."SW Init", error in (no error)=w1024) -> (queue out=w1026:refnum<queue>, error out=w1020:errorcluster)  [unwired: 1 in, 1 out]
            n536 = invoke on="Overlays cluster" class="Clust (strict)" method="Reinit To Default"(error in=w1020) -> (error out=w1016:errorcluster)  [unwired: 2 in, 2 out]
            n537 = call <vilib>:"Set Busy.vi"("error in (no error)"=w1016) -> ("error out"=w1019:errorcluster)  [unwired: 9 in, 1 out]
            n538 = flat-sequence {
              tunnel: w1019 -> [w1028]
              tunnel: [w1028] -> w1018
              frame #0 {
                n539 = Request Deallocation(TRUE ("flag")) -> ()
              }
            }
            n540 = call "0,5s delay"("error in (no error)"=w1018) -> ("error out"=w1017:errorcluster)  [unwired: 10 in]
            n541 = Merge Errors(w1017) -> (w1015:errorcluster)
          }
        }
      }
      frame "Recording post-processing" {
        n542 = Get Notifier Status(notifier=w1038, error in (no error)=w1037) -> (notifier out=w1036:refnum<notifier>, current notification=w1035:T46, error out=w1039:errorcluster)  [unwired: 2 out]
        n543 = Unbundle By Name(w1035) -> ("Offline mode"=w1030:bool)
        n544 = case shown="False" w1030 {
          tunnel: w1039 -> [w1082 w1085]
          tunnel: [w1042 w1085] -> w1033
          tunnel: w1036 -> [w1065 w1084]
          tunnel: w1035 -> [_ _]
          tunnel: [w1065 w1084] -> w1034
          tunnel: w1032 -> [w1063 w1083]
          tunnel: [w1041 w1083] -> w1031
          frame False {
            # "This part is running when working online"
            n545 = local read "Mouse drawing parameters"() -> (w1070:T2)
            n546 = local read "Start time (HW)"() -> (w1073:u32)
            n547 = local read "Diagram (display)"() -> (w1069:T15)
            n548 = local read "Start time (SW)"() -> (w1074:timestamp)
            n549 = call <vilib>:"Set Busy.vi"("error in (no error)"=w1082) -> ("error out"=w1080:errorcluster)  [unwired: 9 in, 1 out]
            n550 = call <vilib>:"Launch Progress Bar.vi"("error in (no error)"=w1080, "Enable Cancellation? (T)"=FALSE, "Main Title (\"Working...\")"="Data post-processing: " ("Main Title (\"Working...\")"), "Total Count"=5) -> ("error out"=w1068:errorcluster, "Progress Bar Dialog"=w1076:refnum<class "Progress Bar Dialog.lvclass">)  [unwired: 6 in]
            n551 = local read "Pixel to zone"() -> (w1049:T3)
            n552 = Bundle By Name(cluster=T65 {"Defragment TDMS? (F)"=FALSE, "Start time (SW)"=timestamp(0 s since 1904-01-01), "Start time (HW)"=0, "Data filtering"={"Filter type"=enum."Savitzky-Golay", "Length"=41, "Order"=3}, "Mouse drawing parameters"={"Trace length, samples"=200, "Rainbow track"=FALSE, "Rainbow track is speed"=FALSE, "Bright mouse lineout"=FALSE, "Colors array"=[255, 1791, 3583, 5119, 6911, 8447, 9983, 11775, 13311, 14847, 16639, 18175, 19711, 21503, 23039, 24831, 26367, 27903, 29695, 31231, 33023, 34559, 36095, 37887, 39423, 40959, 42751, 44287, 45823, 47615, 49151, 50943, 52479, 54015, 55807, 57343, 59135, 60671, 62207, 63999, 65535, 196601, 393202, 524268, 720869, 851935, 1048537, 1245138, 1376204, 1572806, 1703871, 1834937, 2031538, 2162604, 2359206, 2555807, 2686873, 2883475, 3014540, 3211142, 3342208, 3473273, 3669875, 3800940, 3997542, 4128608, 4325209, 4521811, 4652876, 4849478, 4980544, 5111609, 5308211, 5439277, 5635878, 5832480, 5963546, 6094611, 6291213, 6487814, 6618880, 6881024, 7143168, 7405312, 7667456, 7864064, 8126208, 8388352, 8650496, 8912640, 9174784, 9436928, 9633536, 9895680, 10157824, 10419968, 10682112, 10944256, 11206400, 11468544, 11730688, 11927296, 12189440, 12451584, 12713728, 12975872, 13238016, 13500160, 13762304, 13958912, 14221056, 14483200, 14745344, 15007488, 15269632, 15531776, 15793920, 15990528, 16252672, 16514816, 16776960, 16776192, 16775424, 16774400, 16773632, 16772864, 16772096, 16771328, 16770560, 16769536, 16768768, 16768000, 16767232, 16766464, 16765696, 16764672, 16763904, 16763136, 16762368, 16761600, 16760832, 16759808, 16759040, 16758272, 16757504, 16756736, 16755712, 16754944, 16754176, 16753408, 16752640, 16751872, 16750848, 16750080, 16749312, 16748544, 16747776, 16747008, 16745984, 16745216, 16744448, 16743680, 16742912, 16741888, 16741120, 16740352, 16739584, 16738816, 16737792, 16737024, 16736256, 16735488, 16734720, 16733696, 16732928, 16732160, 16731392, 16730624, 16729600, 16728832, 16728064, 16727296, 16726528, 16725504, 16724736, 16723968, 16723200, 16722432, 16721408, 16720640, 16719872, 16719104, 16718336, 16717312, 16716544, 16715776, 16715008, 16714240, 16713216, 16712448], "Pixels per mm"=2.533333333333333}, "Size of the image (480x480)"={"X size"=480.0, "Y size"=480.0}, "Image ref. in"="remote image 00000223CD816B68", "Calibration parameters"={"Timing calibration sw/hw"=1.0, "True FPS"=80.0, "True frame time, s"=0.0125, "Disp. calibration info"=[]}, "Pixel to zone"=[]} ("Processing parameters"), "Defragment TDMS? (F)"=TRUE, "Start time (SW)"=w1074, "Start time (HW)"=w1073, "Data filtering"=T17 {"Filter type"=enum."Savitzky-Golay", "Length"=41, "Order"=3}, "Mouse drawing parameters"=w1070, "Image ref. in"=w1069, "Pixel to zone"=w1049) -> (w1071:T65)
            n553 = global read "SW_Globals_2.2+.vi" "Settings cluster"() -> (w1050:T16)
            n554 = local write "Reset buffers?"(TRUE ("Reset buffers?")) -> ()
            n555 = global read "SW_Globals_2.2+.vi" "Paths"() -> (w1081:T77)
            n556 = call "PR_Recording_post-processing.vi"("Progress Bar Dialog in"=w1076, "error in (no error)"=w1068, "Processing parameters"=w1071, "Paths"=w1081, "Settings cluster"=w1050) -> ("error out"=w1064:errorcluster, "Loaded array data out"=w1057:dbl[][], "Overlays cluster out"=w1067:T27)  [unwired: 4 in]
            n557 = local write "Overlays cluster"(w1067) -> ()
            n558 = Enqueue Element(queue=w1063, element=CTL_Control_States."Prepare loaded data playback", error in (no error)=w1064) -> (queue out=w1044:refnum<queue>, error out=w1043:errorcluster)  [unwired: 1 in, 1 out]
            n559 = Index Array(array=w1057, index (row) #1=0 ("index (row)"), index (row) #2=3 ("index (row)"), index (row) #3=4 ("index (row)"), index (row) #4=5 ("index (row)"), index (row) #5=9 ("index (row)"), index (row) #6=10 ("index (row)")) -> (element #1=w1055:dbl[], element #2=w1054:dbl[], element #3=w1053:dbl[], element #4=w1052:dbl[], element #5=w1051:dbl[], element #6=w1046:dbl[])  [unwired: 6 in]
            n560 = To Byte Integer(number=w1046) -> (8bit integer=w1045:i8[])
            n561 = Enqueue Element(queue=w1044, element=CTL_Control_States."Save density map(s)", error in (no error)=w1043) -> (queue out=w1041:refnum<queue>, error out=w1042:errorcluster)  [unwired: 1 in, 1 out]
            n562 = local write "Loaded.timeline"(w1055) -> ()
            n563 = local write "Loaded.X"(w1053) -> ()
            n564 = local write "Loaded.Y"(w1052) -> ()
            n565 = local write "Loaded.alpha"(w1054) -> ()
            n566 = local write "Loaded.speed"(w1051) -> ()
            n567 = local write "Loaded.zones"(w1045) -> ()
          }
          frame True {
            # "This part is running when working with the recorded data"
          }
        }
      }
      frame "Prepare loaded data playback" {
        n568 = Get Notifier Status(notifier=w1096, error in (no error)=w1095) -> (notifier out=w1094:refnum<notifier>, current notification=w1093:T46, error out=w1097:errorcluster)  [unwired: 2 out]
        n569 = Unbundle By Name(w1093) -> ("Offline mode"=w1086:bool)
        n570 = case shown="True" w1086 {
          tunnel: w1097 -> [w1134 w1168]
          tunnel: [w1138 w1172] -> w1088
          tunnel: w1094 -> [w1137 w1171]
          tunnel: w1093 -> [_ _]
          tunnel: [w1135 w1169] -> w1092
          tunnel: w1091 -> [w1136 w1170]
          tunnel: [w1136 w1170] -> w1090
          frame False {
            w1122 = 0 ("index")
            w1139 = TRUE ("Has been recorded")
            # "This part is running when working online"
            n571 = local read "Loaded.timeline"() -> (w1130:dbl[])
            n572 = global read "SW_Globals_2.2+.vi" "Settings cluster"() -> (w1115:T16)
            n573 = global read "SW_Globals_2.2+.vi" "All references"() -> (w1133:T36)
            n574 = local read "Speed threshold"() -> (w1104:dbl)
            n575 = Array Max & Min(array=w1130) -> (max value=w1131:dbl, max index (indices)=w1128:i32, min value=w1132:dbl, min index (indices)=w1129:i32)
            n576 = call "UI_(08A)_Prepare_loaded_data_playback.vi"("Timeline max, s"=w1131, "error in (no error)"=w1134, "Timeline min, s"=w1132, "Settings cluster in"=w1115, "All references in"=w1133) -> ("error out"=w1108:errorcluster)  [unwired: 3 in, 2 out]
            n577 = Bundle(cluster=cluster{"Min":dbl, "Max":dbl} {"Min"=0.0, "Max"=0.0}, "Min"=w1132, "Max"=w1131) -> (w1125:cluster{"Min":dbl, "Max":dbl})
            n578 = Bundle(cluster=T66 {"TL. min index"=0, "TL. max index"=0}, "TL. min index"=w1129, "TL. max index"=w1128) -> (w1124:T66)
            n579 = Bundle By Name(cluster=T4 {"max"=300.0, "min"=0.0, "# bins"=10, "threshold"=8.0, "thr. type"=enum."higher accepted"} ("Histogram parameters"), "threshold"=w1104) -> (w1111:T4)
            n580 = local write "Timeline absolute min&max indices"(w1124) -> ()
            n581 = local write "Timeline absolute min&max"(w1125) -> ()
            n582 = local write "Timeline min&max"(w1125) -> ()
            n583 = local write "Timeline min&max indices"(w1124) -> ()
            n584 = local read "Loaded.X"() -> (w1107:dbl[])
            n585 = local read "Loaded.Y"() -> (w1106:dbl[])
            n586 = local read "Loaded.alpha"() -> (w1123:dbl[])
            n587 = local read "Loaded.speed"() -> (w1105:dbl[])
            n588 = call "GET_Travel_(offline).vi"("Loaded.X in"=w1107, "Loaded.Y in"=w1106, "Loaded.Speed in"=w1105, "Speed threshold"=w1104, "Error In"=w1108) -> ("Run length, m"=w1100:dbl, "Loaded.Speed out"=w1101:dbl[], "Error Out"=w1109:errorcluster)  [unwired: 8 in]
            n589 = local write "Run distance, m"(w1100) -> ()
            n590 = call "GET_Statistics_(offline).vi"("Error In"=w1109, "Histogram parameters"=w1111, "Data vector in"=w1101) -> ("Error Out"=w1103:errorcluster, "Mean thresholded"=w1098:dbl, "Perc. thresholded"=w1113:dbl, "Histogram data out"=w1112:T32)  [unwired: 3 in]
            n591 = local write "Running, perc. of time"(w1113) -> ()
            n592 = local write "Histograms"(w1112) -> ()
            n593 = call "250 ms delay"("error in (no error)"=w1103) -> ("error out"=w1102:errorcluster)  [unwired: 10 in]
            n594 = Get Notifier Status(notifier=w1137, error in (no error)=w1102) -> (notifier out=w1142:refnum<notifier>, current notification=w1141:T46, error out=w1110:errorcluster)  [unwired: 2 out]
            n595 = Bundle By Name(cluster=w1141, "Data loaded"=w1139, "Has been recorded"=w1139, "Offline mode"=w1139) -> (w1140:T46)
            n596 = local write "Average speed, mm/s"(w1098) -> ()
            n597 = Index Array(array=w1107, index=w1122) -> (element=w1120:dbl)
            n598 = Index Array(array=w1106, index=w1122) -> (element=w1119:dbl)
            n599 = Index Array(array=w1123, index=w1122) -> (element=w1118:dbl)
            n600 = Index Array(array=w1105, index=w1122) -> (element=w1117:dbl)
            n601 = Send Notification(notification=w1140, notifier=w1142, error in (no error)=w1110) -> (notifier out=w1135:refnum<notifier>, error out=w1099:errorcluster)
            n602 = Bundle By Name(cluster=T25 {"R from center"=0.0, "phi (mouse angular position in the cage)"=0.0, "alpha (mouse rot. angle)"=0.0, "X"=0.0, "Y"=0.0, "theta (from center towards mouse)"=0.0, "beta (cage rot. against mouse)"=0.0, "w (mouse angle to wall)"=0.0, "Speed (filtered)"=0.0} ("Animal coordinates and speed"), "X"=w1120, "Y"=w1119, "alpha (mouse rot. angle)"=w1118, "Speed (filtered)"=w1117) -> (w1116:T25)
            n603 = local write "Current position"(w1116) -> ()
            n604 = call <vilib>:"Unset Busy.vi"("error in (no error)"=w1099) -> ("error out"=w1138:errorcluster)  [unwired: 10 in]
          }
          frame True {
            w1154 = 0 ("index")
            w1174 = TRUE ("Has been recorded")
            # "This part is running when working with the recorded data"
            n605 = local read "Loaded.timeline"() -> (w1164:dbl[])
            n606 = global read "SW_Globals_2.2+.vi" "Settings cluster"() -> (w1147:T16)
            n607 = global read "SW_Globals_2.2+.vi" "All references"() -> (w1166:T36)
            n608 = Array Max & Min(array=w1164) -> (max value=w1165:dbl, max index (indices)=w1162:i32, min value=w1143:dbl, min index (indices)=w1163:i32)
            n609 = call "UI_(08A)_Prepare_loaded_data_playback.vi"("Timeline max, s"=w1165, "error in (no error)"=w1168, "Timeline min, s"=w1143, "Settings cluster in"=w1147, "All references in"=w1166) -> ("error out"=w1167:errorcluster)  [unwired: 3 in, 2 out]
            n610 = Bundle(cluster=cluster{"Min":dbl, "Max":dbl} {"Min"=0.0, "Max"=0.0}, "Min"=w1143, "Max"=w1165) -> (w1159:cluster{"Min":dbl, "Max":dbl})
            n611 = Bundle(cluster=T66 {"TL. min index"=0, "TL. max index"=0}, "TL. min index"=w1163, "TL. max index"=w1162) -> (w1158:T66)
            n612 = local write "Timeline absolute min&max indices"(w1158) -> ()
            n613 = local write "Timeline absolute min&max"(w1159) -> ()
            n614 = local read "Start time (SW)"() -> (w1145:timestamp)
            n615 = local write "Timeline min&max"(w1159) -> ()
            n616 = local write "Timeline min&max indices"(w1158) -> ()
            n617 = call "250 ms delay"("error in (no error)"=w1167) -> ("error out"=w1173:errorcluster)  [unwired: 10 in]
            n618 = Add(x=w1143, y=w1145) -> (x+y=w1144:timestamp)
            n619 = local write "Since track start"(w1143) -> ()
            n620 = Get Notifier Status(notifier=w1171, error in (no error)=w1173) -> (notifier out=w1178:refnum<notifier>, current notification=w1177:T46, error out=w1175:errorcluster)  [unwired: 2 out]
            n621 = local write "Current Time"(w1144) -> ()
            n622 = local read "Loaded.X"() -> (w1157:dbl[])
            n623 = local read "Loaded.Y"() -> (w1156:dbl[])
            n624 = local read "Loaded.alpha"() -> (w1155:dbl[])
            n625 = local read "Loaded.speed"() -> (w1153:dbl[])
            n626 = Bundle By Name(cluster=w1177, "Data loaded"=w1174, "Offline mode"=w1174) -> (w1176:T46)
            n627 = Index Array(array=w1157, index=w1154) -> (element=w1151:dbl)
            n628 = Index Array(array=w1156, index=w1154) -> (element=w1150:dbl)
            n629 = Index Array(array=w1155, index=w1154) -> (element=w1149:dbl)
            n630 = Index Array(array=w1153, index=w1154) -> (element=w1148:dbl)
            n631 = Bundle By Name(cluster=T25 {"R from center"=0.0, "phi (mouse angular position in the cage)"=0.0, "alpha (mouse rot. angle)"=0.0, "X"=0.0, "Y"=0.0, "theta (from center towards mouse)"=0.0, "beta (cage rot. against mouse)"=0.0, "w (mouse angle to wall)"=0.0, "Speed (filtered)"=0.0} ("Animal coordinates and speed"), "X"=w1151, "Y"=w1150, "alpha (mouse rot. angle)"=w1149, "Speed (filtered)"=w1148) -> (w1146:T25)
            n632 = Send Notification(notification=w1176, notifier=w1178, error in (no error)=w1175) -> (notifier out=w1169:refnum<notifier>, error out=w1179:errorcluster)
            n633 = local write "Current position"(w1146) -> ()
            n634 = call <vilib>:"Unset Busy.vi"("error in (no error)"=w1179) -> ("error out"=w1172:errorcluster)  [unwired: 10 in]
          }
        }
        n635 = property on="Mouse speed" class="WFChart (strict)"(error in=w1088, "History Data"=waveform(dbl)[] []) -> (error out=w1087:errorcluster)  [unwired: 1 in, 1 out]
      }
      frame "Timeline update" {
        n636 = Get Notifier Status(notifier=w1188, error in (no error)=w1187) -> (notifier out=w1186:refnum<notifier>, current notification=w1185:T46, error out=w1189:errorcluster)  [unwired: 2 out]
        n637 = Unbundle By Name(w1185) -> ("Offline mode"=w1180:bool)
        n638 = case shown="False" w1180 {
          tunnel: w1189 -> [w1198 w1213]
          tunnel: [w1191 w1206] -> w1183
          tunnel: w1186 -> [w1204 w1219]
          tunnel: w1185 -> [_ _]
          tunnel: [w1204 w1219] -> w1184
          tunnel: w1182 -> [w1190 w1205]
          tunnel: [w1190 w1205] -> w1181
          frame True {
            # "This part is running when working offline"
            n639 = local read "Timeline absolute min&max indices"() -> (w1201:T26)
            n640 = local read "Timeline absolute min&max"() -> (w1202:cluster{"Tl. min":dbl, "TL. max":dbl})
            n641 = local read "Timeline min&max indices"() -> (w1199:T26)
            n642 = local read "Timeline min&max"() -> (w1200:cluster{"Tl. min":dbl, "TL. max":dbl})
            n643 = local read "Loaded.timeline"() -> (w1203:dbl[])
            n644 = local read "Timeline"() -> (w1196:T37)
            n645 = call "UI_Update_timeline.vi"("Timeline values in"=w1196, "Loaded.timeline"=w1203, "Timeline absolute min&max in"=w1202, "Timeline absolute min&max indices in"=w1201, "Timeline min&max in"=w1200, "Timeline min&max indices in"=w1199, "Error In"=w1198) -> ("Timeline values out"=w1197:T81, "Cur. pos. slider index"=w1193:i32, "Update timeline index?"=w1192:bool, "Timeline min&max out"=w1195:cluster{"Tl. min":dbl, "TL. max":dbl}, "Error Out"=w1191:errorcluster, "Timeline min&max indices out"=w1194:T26)  [unwired: 3 in]
            n646 = local write "Cur. pos. slider index"(w1193) -> ()
            n647 = local write "Update timeline index?"(w1192) -> ()
            n648 = local write "Timeline"(w1197) -> ()
            n649 = local write "Timeline min&max indices"(w1194) -> ()
            n650 = local write "Timeline min&max"(w1195) -> ()
            n651 = local write "Reset buffers?"(w1192) -> ()
          }
          frame False {
            # "This part is running when working with the recorded data"
            n652 = local read "Timeline absolute min&max indices"() -> (w1216:T26)
            n653 = local read "Timeline absolute min&max"() -> (w1217:cluster{"Tl. min":dbl, "TL. max":dbl})
            n654 = local read "Timeline min&max indices"() -> (w1214:T26)
            n655 = local read "Timeline min&max"() -> (w1215:cluster{"Tl. min":dbl, "TL. max":dbl})
            n656 = local read "Loaded.timeline"() -> (w1218:dbl[])
            n657 = local read "Timeline"() -> (w1211:T37)
            n658 = call "UI_Update_timeline.vi"("Timeline values in"=w1211, "Loaded.timeline"=w1218, "Timeline absolute min&max in"=w1217, "Timeline absolute min&max indices in"=w1216, "Timeline min&max in"=w1215, "Timeline min&max indices in"=w1214, "Error In"=w1213) -> ("Timeline values out"=w1212:T81, "Cur. pos. slider index"=w1208:i32, "Update timeline index?"=w1207:bool, "Timeline min&max out"=w1210:cluster{"Tl. min":dbl, "TL. max":dbl}, "Error Out"=w1206:errorcluster, "Timeline min&max indices out"=w1209:T26)  [unwired: 3 in]
            n659 = local write "Cur. pos. slider index"(w1208) -> ()
            n660 = local write "Update timeline index?"(w1207) -> ()
            n661 = local write "Timeline"(w1212) -> ()
            n662 = local write "Timeline min&max indices"(w1209) -> ()
            n663 = local write "Timeline min&max"(w1210) -> ()
            n664 = local write "Reset buffers?"(w1207) -> ()
          }
        }
      }
      frame "Overlay tracks update" {
        n665 = Get Notifier Status(notifier=w1228, error in (no error)=w1227) -> (notifier out=w1226:refnum<notifier>, current notification=w1225:T46, error out=w1229:errorcluster)  [unwired: 2 out]
        n666 = Unbundle By Name(w1225) -> ("Offline mode"=w1220:bool)
        n667 = case shown="False" w1220 {
          tunnel: w1229 -> [w1266 w1311]
          tunnel: [w1251 w1296] -> w1223
          tunnel: w1226 -> [w1274 w1319]
          tunnel: w1225 -> [_ _]
          tunnel: [w1274 w1319] -> w1224
          tunnel: w1222 -> [w1265 w1310]
          tunnel: [w1265 w1310] -> w1221
          frame True {
            w1262 = cluster{"x":i32, "y":i32} {"x"=480, "y"=480}  # Image size
            # "This part is running when working offline"
            n668 = local read "Mouse drawing parameters"() -> (w1260:T2)
            n669 = local read "Loaded.speed"() -> (w1269:dbl[])
            n670 = call <vilib>:"Set Busy.vi"("error in (no error)"=w1266) -> ("error out"=w1244:errorcluster)  [unwired: 9 in, 1 out]
            n671 = local read "Timeline min&max indices"() -> (w1272:T26)
            n672 = local read "Loaded.X"() -> (w1273:dbl[])
            n673 = local read "Loaded.Y"() -> (w1270:dbl[])
            n674 = local read "Speed threshold"() -> (w1240:dbl)
            n675 = Unbundle By Name(w1260) -> ("Pixels per mm"=w1256:dbl)
            n676 = Unbundle By Name(w1272) -> ("Tl. min index"=w1268:i32, "Tl. max index"=w1271:i32)
            n677 = Bundle By Name(cluster=T4 {"max"=300.0, "min"=0.0, "# bins"=10, "threshold"=8.0, "thr. type"=enum."higher accepted"} ("Histogram parameters"), "threshold"=w1240) -> (w1246:T4)
            n678 = local read "Overlays cluster"() -> (w1230:T27)
            n679 = local read "Stats parameters (online)"() -> (w1236:T1)
            n680 = Subtract(x=w1271, y=w1268) -> (x-y=w1267:i32)
            n681 = Array Subset(array=w1273, index=w1268, length=w1267) -> (w1238:dbl[])
            n682 = Array Subset(array=w1270, index=w1268, length=w1267) -> (w1239:dbl[])
            n683 = Array Subset(array=w1269, index=w1268, length=w1267) -> (w1231:dbl[])
            n684 = Multiply(x=w1238, y=w1256) -> (x*y=w1264:dbl[])
            n685 = Multiply(x=w1239, y=w1256) -> (x*y=w1255:dbl[])
            n686 = call "GET_Travel_(offline).vi"("Loaded.X in"=w1238, "Loaded.Y in"=w1239, "Loaded.Speed in"=w1231, "Speed threshold"=w1240, "Error In"=w1244) -> ("Run length, m"=w1241:dbl, "Loaded.Speed out"=w1242:dbl[], "Error Out"=w1243:errorcluster)  [unwired: 8 in]
            n687 = local write "Run distance, m"(w1241) -> ()
            n688 = call "GET_Statistics_(offline).vi"("Error In"=w1243, "Histogram parameters"=w1246, "Data vector in"=w1242) -> ("Error Out"=w1247:errorcluster, "Mean thresholded"=w1237:dbl, "Perc. thresholded"=w1250:dbl, "Histogram data out"=w1249:T32)  [unwired: 3 in]
            n689 = Unbundle By Name(w1236) -> ("Size of the image (480x480)"=w1235:T82)
            n690 = local write "Histograms"(w1249) -> ()
            n691 = local write "Running, perc. of time"(w1250) -> ()
            n692 = Quotient & Remainder(x=w1262, y=T67 {"Width"=2, "Height"=2}) -> (floor(x/y)=w1261:T67)  [unwired: 1 out]
            n693 = local write "Average speed, mm/s"(w1237) -> ()
            n694 = Unbundle(w1261) -> ("Width"=w1259:u32, "Height"=w1254:u32)
            n695 = Add(x=w1264, y=w1259) -> (x+y=w1258:dbl[])
            n696 = Add(x=w1255, y=w1254) -> (x+y=w1253:dbl[])
            n697 = Round To Nearest(number=w1258) -> (nearest integer value=w1257:dbl[])
            n698 = Round To Nearest(number=w1253) -> (nearest integer value=w1252:dbl[])
            n699 = Build Cluster Array(w1257, w1252) -> (w1232:cluster{dbl, dbl}[])
            n700 = call "DRAW_Track_overlays_(offline).vi"("Image size"=w1235, "Overlays cluster in"=w1230, "Full track array"=w1232, "Speed array"=w1231, "Error In"=w1244) -> ("Overlays cluster out"=w1233:T27, "Error Out"=w1234:errorcluster)  [unwired: 9 in]
            n701 = local write "Active part of track"(w1232) -> ()
            n702 = local write "Overlays cluster"(w1233) -> ()
            n703 = local write "Active speed chunk"(w1231) -> ()
            n704 = Merge Errors(w1234, w1247) -> (w1248:errorcluster)
            n705 = call <vilib>:"Unset Busy.vi"("error in (no error)"=w1248) -> ("error out"=w1251:errorcluster)  [unwired: 10 in]
          }
          frame False {
            w1307 = cluster{"x":i32, "y":i32} {"x"=480, "y"=480}  # Image size
            # "This part is running when working with just recorded data"
            n706 = local read "Mouse drawing parameters"() -> (w1305:T2)
            n707 = local read "Loaded.speed"() -> (w1314:dbl[])
            n708 = call <vilib>:"Set Busy.vi"("error in (no error)"=w1311) -> ("error out"=w1289:errorcluster)  [unwired: 9 in, 1 out]
            n709 = local read "Timeline min&max indices"() -> (w1317:T26)
            n710 = local read "Loaded.X"() -> (w1318:dbl[])
            n711 = local read "Loaded.Y"() -> (w1315:dbl[])
            n712 = local read "Speed threshold"() -> (w1285:dbl)
            n713 = Unbundle By Name(w1305) -> ("Pixels per mm"=w1301:dbl)
            n714 = Bundle By Name(cluster=T4 {"max"=300.0, "min"=0.0, "# bins"=10, "threshold"=8.0, "thr. type"=enum."higher accepted"} ("Histogram parameters"), "threshold"=w1285) -> (w1291:T4)
            n715 = Unbundle By Name(w1317) -> ("Tl. min index"=w1313:i32, "Tl. max index"=w1316:i32)
            n716 = local read "Overlays cluster"() -> (w1275:T27)
            n717 = Subtract(x=w1316, y=w1313) -> (x-y=w1312:i32)
            n718 = Array Subset(array=w1318, index=w1313, length=w1312) -> (w1283:dbl[])
            n719 = Array Subset(array=w1315, index=w1313, length=w1312) -> (w1284:dbl[])
            n720 = Array Subset(array=w1314, index=w1313, length=w1312) -> (w1276:dbl[])
            n721 = Multiply(x=w1283, y=w1301) -> (x*y=w1309:dbl[])
            n722 = Multiply(x=w1284, y=w1301) -> (x*y=w1300:dbl[])
            n723 = call "GET_Travel_(offline).vi"("Loaded.X in"=w1283, "Loaded.Y in"=w1284, "Loaded.Speed in"=w1276, "Speed threshold"=w1285, "Error In"=w1289) -> ("Run length, m"=w1286:dbl, "Loaded.Speed out"=w1287:dbl[], "Error Out"=w1288:errorcluster)  [unwired: 8 in]
            n724 = local read "Stats parameters (online)"() -> (w1281:T1)
            n725 = local write "Run distance, m"(w1286) -> ()
            n726 = call "GET_Statistics_(offline).vi"("Error In"=w1288, "Histogram parameters"=w1291, "Data vector in"=w1287) -> ("Error Out"=w1294:errorcluster, "Mean thresholded"=w1282:dbl, "Perc. thresholded"=w1293:dbl, "Histogram data out"=w1292:T32)  [unwired: 3 in]
            n727 = Unbundle By Name(w1281) -> ("Size of the image (480x480)"=w1280:T82)
            n728 = local write "Histograms"(w1292) -> ()
            n729 = local write "Average speed, mm/s"(w1282) -> ()
            n730 = Quotient & Remainder(x=w1307, y=T67 {"Width"=2, "Height"=2}) -> (floor(x/y)=w1306:T67)  [unwired: 1 out]
            n731 = local write "Running, perc. of time"(w1293) -> ()
            n732 = Unbundle(w1306) -> ("Width"=w1304:u32, "Height"=w1299:u32)
            n733 = Add(x=w1309, y=w1304) -> (x+y=w1303:dbl[])
            n734 = Add(x=w1300, y=w1299) -> (x+y=w1298:dbl[])
            n735 = Round To Nearest(number=w1303) -> (nearest integer value=w1302:dbl[])
            n736 = Round To Nearest(number=w1298) -> (nearest integer value=w1297:dbl[])
            n737 = Build Cluster Array(w1302, w1297) -> (w1277:cluster{dbl, dbl}[])
            n738 = call "DRAW_Track_overlays_(offline).vi"("Image size"=w1280, "Overlays cluster in"=w1275, "Full track array"=w1277, "Speed array"=w1276, "Error In"=w1289) -> ("Overlays cluster out"=w1278:T27, "Error Out"=w1279:errorcluster)  [unwired: 9 in]
            n739 = local write "Active part of track"(w1277) -> ()
            n740 = local write "Overlays cluster"(w1278) -> ()
            n741 = local write "Active speed chunk"(w1276) -> ()
            n742 = Merge Errors(w1279, w1294) -> (w1295:errorcluster)
            n743 = call <vilib>:"Unset Busy.vi"("error in (no error)"=w1295) -> ("error out"=w1296:errorcluster)  [unwired: 10 in]
          }
        }
      }
      frame "Location map update" {
        n744 = Get Notifier Status(notifier=w1328, error in (no error)=w1327) -> (notifier out=w1326:refnum<notifier>, current notification=w1325:T46, error out=w1329:errorcluster)  [unwired: 2 out]
        n745 = Unbundle By Name(w1325) -> ("Offline mode"=w1320:bool)
        n746 = case shown="False" w1320 {
          tunnel: w1329 -> [w1344 w1360]
          tunnel: [w1342 w1358] -> w1323
          tunnel: w1326 -> [w1345 w1361]
          tunnel: w1325 -> [_ _]
          tunnel: [w1345 w1361] -> w1324
          tunnel: w1322 -> [w1343 w1359]
          tunnel: [w1343 w1359] -> w1321
          frame False {
            # "This part is running when working with just recorded data"
            n747 = call <vilib>:"Set Busy.vi"("error in (no error)"=w1344) -> ("error out"=w1334:errorcluster)  [unwired: 9 in, 1 out]
            n748 = local read "Stats parameters (online)"() -> (w1341:T1)
            n749 = Unbundle By Name(w1341) -> ("Size of the image (480x480)"=w1339:T82)
            n750 = local read "Active part of track"() -> (w1336:cluster{"Numeric":dbl, "Numeric":dbl}[])
            n751 = call "GET_Location-based_density_map.vi"("ImageSize"=w1339, "XY data"=w1336, "Log2-transform? (T)"=TRUE, "Normalize to 8 bit? (T)"=TRUE, "error in (no error)"=w1334, "Output as Image? (F)"=TRUE) -> ("8-bit pixmap out"=w1340:u32[][], "Density array out"=w1330:dbl[][], "error out"=w1333:errorcluster)  [unwired: 7 in]
            n752 = local read "Overlays cluster"() -> (w1337:T27)
            n753 = Bundle By Name(cluster=w1337, "Location density map image"=w1340, "Location density map"=w1330) -> (w1338:T27)
            n754 = local write "Overlays cluster"(w1338) -> ()
            n755 = call <vilib>:"Unset Busy.vi"("error in (no error)"=w1333) -> ("error out"=w1342:errorcluster)  [unwired: 10 in]
          }
          frame True {
            # "This part is running when working offline"
            n756 = call <vilib>:"Set Busy.vi"("error in (no error)"=w1360) -> ("error out"=w1347:errorcluster)  [unwired: 9 in, 1 out]
            n757 = local read "Stats parameters (online)"() -> (w1357:T1)
            n758 = local read "Active part of track"() -> (w1352:cluster{"Numeric":dbl, "Numeric":dbl}[])
            n759 = Unbundle By Name(w1357) -> ("Size of the image (480x480)"=w1355:T82)
            n760 = call "GET_Location-based_density_map.vi"("ImageSize"=w1355, "XY data"=w1352, "Log2-transform? (T)"=TRUE, "Normalize to 8 bit? (T)"=TRUE, "error in (no error)"=w1347, "Output as Image? (F)"=TRUE) -> ("8-bit pixmap out"=w1356:u32[][], "Density array out"=w1346:dbl[][], "error out"=w1348:errorcluster)  [unwired: 7 in]
            n761 = local read "Overlays cluster"() -> (w1353:T27)
            n762 = Bundle By Name(cluster=w1353, "Location density map image"=w1356, "Location density map"=w1346) -> (w1354:T27)
            n763 = local write "Overlays cluster"(w1354) -> ()
            n764 = call <vilib>:"Unset Busy.vi"("error in (no error)"=w1348) -> ("error out"=w1358:errorcluster)  [unwired: 10 in]
          }
        }
      }
      frame "Speed map update" {
        n765 = Get Notifier Status(notifier=w1370, error in (no error)=w1369) -> (notifier out=w1368:refnum<notifier>, current notification=w1367:T46, error out=w1371:errorcluster)  [unwired: 2 out]
        n766 = Unbundle By Name(w1367) -> ("Offline mode"=w1362:bool)
        n767 = case shown="False" w1362 {
          tunnel: w1371 -> [w1387 w1404]
          tunnel: [w1385 w1402] -> w1365
          tunnel: w1368 -> [w1388 w1405]
          tunnel: w1367 -> [_ _]
          tunnel: [w1388 w1405] -> w1366
          tunnel: w1364 -> [w1386 w1403]
          tunnel: [w1386 w1403] -> w1363
          frame True {
            # "This part is running when working offline"
            n768 = call <vilib>:"Set Busy.vi"("error in (no error)"=w1387) -> ("error out"=w1377:errorcluster)  [unwired: 9 in, 1 out]
            n769 = local read "Stats parameters (online)"() -> (w1384:T1)
            n770 = Unbundle By Name(w1384) -> ("Size of the image (480x480)"=w1382:T82)
            n771 = local read "Active part of track"() -> (w1379:cluster{"Numeric":dbl, "Numeric":dbl}[])
            n772 = local read "Active speed chunk"() -> (w1373:dbl[])
            n773 = call "GET_Speed-based_density_map.vi"("ImageSize"=w1382, "XY data"=w1379, "Log2-transform? (T)"=TRUE, "Normalize to 8 bit? (T)"=TRUE, "error in (no error)"=w1377, "Output as Image? (F)"=TRUE, "Loaded.speed"=w1373) -> ("8-bit pixmap out"=w1383:u32[][], "Density array out"=w1372:dbl[][], "error out"=w1376:errorcluster)  [unwired: 6 in]
            n774 = local read "Overlays cluster"() -> (w1380:T27)
            n775 = Bundle By Name(cluster=w1380, "Speed density map image"=w1383, "Speed density map"=w1372) -> (w1381:T27)
            n776 = local write "Overlays cluster"(w1381) -> ()
            n777 = call <vilib>:"Unset Busy.vi"("error in (no error)"=w1376) -> ("error out"=w1385:errorcluster)  [unwired: 10 in]
          }
          frame False {
            # "This part is running when working with just recorded data"
            n778 = call <vilib>:"Set Busy.vi"("error in (no error)"=w1404) -> ("error out"=w1394:errorcluster)  [unwired: 9 in, 1 out]
            n779 = local read "Stats parameters (online)"() -> (w1401:T1)
            n780 = local read "Active part of track"() -> (w1396:cluster{"Numeric":dbl, "Numeric":dbl}[])
            n781 = Unbundle By Name(w1401) -> ("Size of the image (480x480)"=w1399:T82)
            n782 = local read "Active speed chunk"() -> (w1390:dbl[])
            n783 = call "GET_Speed-based_density_map.vi"("ImageSize"=w1399, "XY data"=w1396, "Log2-transform? (T)"=TRUE, "Normalize to 8 bit? (T)"=TRUE, "error in (no error)"=w1394, "Output as Image? (F)"=TRUE, "Loaded.speed"=w1390) -> ("8-bit pixmap out"=w1400:u32[][], "Density array out"=w1389:dbl[][], "error out"=w1393:errorcluster)  [unwired: 6 in]
            n784 = local read "Overlays cluster"() -> (w1397:T27)
            n785 = Bundle By Name(cluster=w1397, "Speed density map image"=w1400, "Speed density map"=w1389) -> (w1398:T27)
            n786 = local write "Overlays cluster"(w1398) -> ()
            n787 = call <vilib>:"Unset Busy.vi"("error in (no error)"=w1393) -> ("error out"=w1402:errorcluster)  [unwired: 10 in]
          }
        }
      }
      frame "Load recorded data" {
        n788 = global read "SW_Globals_2.2+.vi" "Paths"() -> (w1422:T77)
        n789 = call <vilib>:"Set Busy.vi"("error in (no error)"=w1421) -> ("error out"=w1409:errorcluster)  [unwired: 9 in, 1 out]
        n790 = Unbundle By Name(w1422) -> ("Folder"=w1411:path)
        n791 = Strip Path(path=w1411) -> (stripped path=w1410:path)  [unwired: 1 out]
        n792 = call "File Dialog"("start path"=w1410, "prompt"="Open previously recorded track", "button label"="Open", "error in"=w1409, "pattern (all files)"="*.tdms", "pattern label"="MHC track") -> ("selected path"=w1412:path, "exists"=w1413:bool, "cancelled"=w1414:bool, "error out"=w1416:errorcluster)  [unwired: 6 in]
        n793 = case shown="No Error" w1416 {
          selector: w1416 -> [w1426 w1466]
          tunnel: w1414 -> [w1431 _]
          tunnel: w1413 -> [w1429 _]
          tunnel: w1412 -> [w1427 _]
          tunnel: [w1425 w1470] -> w1408
          tunnel: w1407 -> [w1424 w1469]
          tunnel: [w1423 w1468] -> w1406
          frame No Error {
            n794 = Not(x=w1431) -> (.not. x?=w1430:bool)
            n795 = And(x=w1429, y=w1430) -> (x .and. y?=w1428:bool)
            n796 = case shown="True" w1428 {
              tunnel: w1427 -> [_ w1447]
              tunnel: w1426 -> [w1435 w1463]
              tunnel: [w1437 w1453] -> w1425
              tunnel: w1424 -> [w1434 w1444]
              tunnel: [w1433 w1440] -> w1423
              frame False {
                n797 = Enqueue Element(queue=w1434, element=CTL_Control_States."Switch to Online mode", error in (no error)=w1435) -> (queue out=w1433:refnum<queue>, error out=w1432:errorcluster)  [unwired: 1 in, 1 out]
                n798 = call <vilib>:"Unset Busy.vi"("error in (no error)"=w1432) -> ("error out"=w1437:errorcluster)  [unwired: 10 in]
              }
              frame True {
                n799 = local write "Loaded.TDMS.path"(w1447) -> ()
                n800 = call "SW_Load_proc_data_from_TDMS.vi"("error in (no error)"=w1463, "TDMS track ref. in"=w1447) -> ("error out"=w1445:errorcluster, "Rec start Time Stamp"=w1439:timestamp, "Loaded data output"=w1438:T83)  [unwired: 7 in]
                n801 = Unbundle By Name(w1438) -> ("HW ts and Frame HW time"=w1452:u32[][], "SW timestamp"=w1451:dbl[], "Coords data"=w1450:dbl[][], "TTL IO and Key"=w1449:string[][], "Track properties"=w1441:string[][], "Zone"=w1448:i8[])
                n802 = local write "Start time (SW)"(w1439) -> ()
                n803 = Enqueue Element(queue=w1444, element=CTL_Control_States."Switch to Offline mode", error in (no error)=w1445) -> (queue out=w1443:refnum<queue>, error out=w1446:errorcluster)  [unwired: 1 in, 1 out]
                n804 = local write "Loaded.zones"(w1448) -> ()
                n805 = local write "Loaded.HW ts and Frame HW time"(w1452) -> ()
                n806 = local write "Loaded.timeline"(w1451) -> ()
                n807 = local write "Loaded.Properties"(w1441) -> ()
                n808 = local write "Loaded.TTL IO and Key"(w1449) -> ()
                n809 = Enqueue Element(queue=w1443, element=CTL_Control_States."Process loaded settings", error in (no error)=w1446) -> (queue out=w1440:refnum<queue>, error out=w1453:errorcluster)  [unwired: 1 in, 1 out]
                n810 = Index Array(array=w1450, index (row) #1=0 ("index (row)"), index (row) #2=1 ("index (row)"), index (row) #3=2 ("index (row)"), index (row) #4=3 ("index (row)")) -> (element #1=w1458:dbl[], element #2=w1457:dbl[], element #3=w1456:dbl[], element #4=w1455:dbl[])  [unwired: 4 in]
                n811 = local write "Loaded.X"(w1458) -> ()
                n812 = local write "Loaded.Y"(w1457) -> ()
                n813 = local write "Loaded.alpha"(w1456) -> ()
                n814 = local write "Loaded.speed"(w1455) -> ()
              }
            }
          }
          frame Error {
            n815 = call <vilib>:"Clear Errors.vi"("error in (no error)"=w1466) -> ("error out"=w1465:errorcluster)  [unwired: 5 in, 1 out]
            n816 = Enqueue Element(queue=w1469, element=CTL_Control_States."Switch to Online mode", error in (no error)=w1465) -> (queue out=w1468:refnum<queue>, error out=w1464:errorcluster)  [unwired: 1 in, 1 out]
            n817 = call <vilib>:"Unset Busy.vi"("error in (no error)"=w1464) -> ("error out"=w1470:errorcluster)  [unwired: 10 in]
          }
        }
      }
      frame "Recalculate track with new settings" {
        n818 = disable-structure shown="Disabled" {
          disable-tunnel: w1473 -> [w1485 _]
          disable-tunnel: [w1483 _] -> w1472
          disable-tunnel: w1471 -> [w1482 _]
          frame Disabled {
            n819 = call <vilib>:"Set Busy.vi"("error in (no error)"=w1485) -> ("error out"=w1481:errorcluster)  [unwired: 9 in, 1 out]
            n820 = call "Start Module.vi"("error in (no error)"=w1481) -> ("error out"=w1480:errorcluster, "Wait for Event Sync?"=w1477:bool, "Tracks Repair Broadcast Events"=w1479:T42)  [unwired: 7 in, 1 out]
            n821 = register-events(reference=w1482, error in=w1480, w1479) -> (error out=w1478:errorcluster)  [unwired: 3 in, 1 out]
            n822 = call "Synchronize Module Events.vi"("error in (no error)"=w1478, "Wait for Event Sync?"=w1477) -> ("error out"=w1476:errorcluster)  [unwired: 9 in]
            n823 = call "Show Panel.vi"("error in (no error)"=w1476) -> ("error out"=w1484:errorcluster)  [unwired: 10 in]
            n824 = call <vilib>:"Unset Busy.vi"("error in (no error)"=w1484) -> ("error out"=w1483:errorcluster)  [unwired: 10 in]
          }
          frame Enabled {
          }
        }
      }
      frame "Load custom settings" {
        n825 = global read "SW_Globals_2.2+.vi" "Paths"() -> (w1503:T77)
        n826 = call <vilib>:"Set Busy.vi"("error in (no error)"=w1502) -> ("error out"=w1490:errorcluster)  [unwired: 9 in, 1 out]
        n827 = Unbundle By Name(w1503) -> ("Folder"=w1492:path)
        n828 = Strip Path(path=w1492) -> (stripped path=w1491:path)  [unwired: 1 out]
        n829 = call "Load Settings"("start path"=w1491, "prompt"="Load previously saved settings", "button label"="Load", "error in"=w1490, "pattern (all files)"="*.trset", "pattern label"="Tracker settings") -> ("selected path"=w1493:path, "exists"=w1494:bool, "cancelled"=w1495:bool, "error out"=w1497:errorcluster)  [unwired: 6 in]
        n830 = case shown="No Error" w1497 {
          selector: w1497 -> [w1507 w1523]
          tunnel: w1495 -> [w1512 _]
          tunnel: w1494 -> [w1510 _]
          tunnel: w1493 -> [w1508 _]
          tunnel: [w1506 w1525] -> w1489
          tunnel: w1486 -> [w1505 w1524]
          tunnel: [w1504 w1524] -> w1488
          frame No Error {
            n831 = Not(x=w1512) -> (.not. x?=w1511:bool)
            n832 = And(x=w1510, y=w1511) -> (x .and. y?=w1509:bool)
            n833 = case shown="True" w1509 {
              tunnel: w1508 -> [_ w1516]
              tunnel: w1507 -> [w1513 w1518]
              tunnel: [w1513 w1517] -> w1506
              tunnel: w1505 -> [w1514 w1519]
              tunnel: [w1514 w1520] -> w1504
              frame False {
              }
              frame True {
                n834 = local write "Settings path to load"(w1516) -> ()
                n835 = local write "Load custom? (F)"(TRUE ("Load custom? (F)")) -> ()
                n836 = Enqueue Element(queue=w1519, element=CTL_Control_States."Start over", error in (no error)=w1518) -> (queue out=w1520:refnum<queue>, error out=w1517:errorcluster)  [unwired: 1 in, 1 out]
              }
            }
          }
          frame Error {
            n837 = call <vilib>:"Simple Error Handler.vi"("error in (no error)"=w1523) -> ("error out"=w1522:errorcluster)  [unwired: 4 in, 4 out]
            n838 = call <vilib>:"Clear Errors.vi"("error in (no error)"=w1522) -> ("error out"=w1525:errorcluster)  [unwired: 5 in, 1 out]
          }
        }
        n839 = call <vilib>:"Unset Busy.vi"("error in (no error)"=w1489) -> ("error out"=w1487:errorcluster)  [unwired: 10 in]
      }
      frame "Process loaded settings" {
        w1564 = 1 ("disabled index (col)")
        n840 = local read "Loaded.Properties"() -> (w1567:string[][])
        n841 = global read "SW_Globals_2.2+.vi" "All references"() -> (w1563:T36)
        n842 = local read "Loaded.TDMS.path"() -> (w1535:path)
        n843 = Index Array(array=w1567, index (row) #1=3 ("index (row)"), index (col) #1=w1564, index (row) #2=4 ("index (row)"), index (col) #2=w1564) -> (element #1=w1529:string)  [unwired: 1 out]
        n844 = call "SW_Save_Cluster_from_String.vi"("Data String in"=w1529, "Settings cluster in"=T16 {"Defaults"={"Default User"=0.0, "VISA Resource Name "="Tracker", "Histogram parameters"={"max"=300.0, "min"=0.0, "# bins"=10, "threshold"=8.0, "thr. type"=enum."higher accepted"}}, "Recording and saving"={"Researcher name"="Researcher", "Name prefix"="Track", "Data post-processing"={"Filter type"=enum."Savitzky-Golay", "Length"=31, "Order"=3}, "Stop at"=0.0, "\"Stop at\" enabled"=FALSE, "Default save folder path"=path "", "Acquisition FPS"=enum."Max"}, "Geometry"={"Sensor board size"=enum."", "Bridge swap"=FALSE, "Twisted neck"=FALSE, "Bridge H. offset"=0.0, "Bridge V. offset"=0.0, "Magnets orientation"=180.0, "Cage type"=0, "Cage parameters"={"Round"=variant(i16 0), "Square"=variant(u16 30), "Donut-maze"=variant(u16 75), "T-maze"=variant(u8 2), "Sociability-maze"=variant(u8 4)}}, "IO parameters"={"IO general config."=12, "IO 1 configuration"=1, "IO 2 configuration"=1, "IO 3 configuration"=0, "IO 4 configuration"=0, "Activate ext. RS-232"=0, "IO inversion config."=0, "Sync capability"=1}, "Conditions presets array"=[{"Enabled"=FALSE, "Name"="", "Specifier(s)"=[], "Response"={"Response type"=enum."Air puff", "TTL port"=enum."Port 1", "TTL pulse length, ms"=0.0}, "Has been set"=FALSE}, {"Enabled"=FALSE, "Name"="", "Specifier(s)"=[], "Response"={"Response type"=enum."Air puff", "TTL port"=enum."Port 1", "TTL pulse length, ms"=0.0}, "Has been set"=FALSE}, {"Enabled"=FALSE, "Name"="", "Specifier(s)"=[], "Response"={"Response type"=enum."Air puff", "TTL port"=enum."Port 1", "TTL pulse length, ms"=0.0}, "Has been set"=FALSE}, {"Enabled"=FALSE, "Name"="", "Specifier(s)"=[], "Response"={"Response type"=enum."Air puff", "TTL port"=enum."Port 1", "TTL pulse length, ms"=0.0}, "Has been set"=FALSE}, {"Enabled"=FALSE, "Name"="", "Specifier(s)"=[], "Response"={"Response type"=enum."Air puff", "TTL port"=enum."Port 1", "TTL pulse length, ms"=0.0}, "Has been set"=FALSE}, {"Enabled"=FALSE, "Name"="", "Specifier(s)"=[], "Response"={"Response type"=enum."Air puff", "TTL port"=enum."Port 1", "TTL pulse length, ms"=0.0}, "Has been set"=FALSE}, {"Enabled"=FALSE, "Name"="", "Specifier(s)"=[], "Response"={"Response type"=enum."Air puff", "TTL port"=enum."Port 1", "TTL pulse length, ms"=0.0}, "Has been set"=FALSE}, {"Enabled"=FALSE, "Name"="", "Specifier(s)"=[], "Response"={"Response type"=enum."Air puff", "TTL port"=enum."Port 1", "TTL pulse length, ms"=0.0}, "Has been set"=FALSE}, {"Enabled"=FALSE, "Name"="", "Specifier(s)"=[], "Response"={"Response type"=enum."Air puff", "TTL port"=enum."Port 1", "TTL pulse length, ms"=0.0}, "Has been set"=FALSE}, {"Enabled"=FALSE, "Name"="", "Specifier(s)"=[], "Response"={"Response type"=enum."Air puff", "TTL port"=enum."Port 1", "TTL pulse length, ms"=0.0}, "Has been set"=FALSE}, {"Enabled"=FALSE, "Name"="", "Specifier(s)"=[], "Response"={"Response type"=enum."Air puff", "TTL port"=enum."Port 1", "TTL pulse length, ms"=0.0}, "Has been set"=FALSE}, {"Enabled"=FALSE, "Name"="", "Specifier(s)"=[], "Response"={"Response type"=enum."Air puff", "TTL port"=enum."Port 1", "TTL pulse length, ms"=0.0}, "Has been set"=FALSE}, {"Enabled"=FALSE, "Name"="", "Specifier(s)"=[], "Response"={"Response type"=enum."Air puff", "TTL port"=enum."Port 1", "TTL pulse length, ms"=0.0}, "Has been set"=FALSE}, {"Enabled"=FALSE, "Name"="", "Specifier(s)"=[], "Response"={"Response type"=enum."Air puff", "TTL port"=enum."Port 1", "TTL pulse length, ms"=0.0}, "Has been set"=FALSE}], "Calibration parameters"={"Timing calibration sw/hw"=1.0, "True FPS"=80.0, "True frame time, s"=0.0125, "Disp. calibration info"=[]}, "Settings loaded OK"=FALSE} ("Settings cluster"), "error in (no error)"=w1528) -> ("Settings cluster out"=w1526:T16, "error out"=w1527:errorcluster)  [unwired: 3 in]
        n845 = Unbundle By Name(w1563) -> ("Indicators references.IO status indicator"=w1562:refnum<vi>)
        n846 = Strip Path(path=w1535) -> (stripped path=w1531:path)  [unwired: 1 out]
        n847 = Unbundle By Name(w1526) -> ("Calibration parameters.True frame time, s"=w1559:dbl, "IO parameters"=w1555:T22)
        n848 = Bundle By Name(cluster=w1526, "Recording and saving.Default save folder path"=w1531) -> (w1536:T16)
        n849 = local write "Act. frame time, s"(w1559) -> ()
        n850 = call "SW_get_IO_ports_representation_2.vi"("Sync parameters cluster input"=w1555) -> ("IO status indicator"=w1561:T39)
        n851 = local write "Settings cluster (local)"(w1526) -> ()
        n852 = property class="Clust"(reference=w1562, error in=w1527, "Value"=w1561) -> (error out=w1560:errorcluster)  [unwired: 1 out]
        n853 = global read "SW_Globals_2.2+.vi" "Paths"() -> (w1537:T77)
        n854 = call "SW_Get_Save_Paths_2.vi"("Settings cluster in"=w1536, "Paths in"=w1537, "error in (no error)"=w1527, "Create new? (F)"=FALSE) -> ("Paths out"=w1533:T77, "error out"=w1532:errorcluster)  [unwired: 1 in, 2 out]
        n855 = Merge Errors(w1532, w1527, w1560) -> (w1568:errorcluster)
        n856 = Enqueue Element(queue=w1558, element=CTL_Control_States."Zones layout update", error in (no error)=w1568) -> (queue out=w1551:refnum<queue>, error out=w1553:errorcluster)  [unwired: 1 in, 1 out]
        n857 = global write "SW_Globals_2.2+.vi" "Paths"(w1533) -> ()
        n858 = Enqueue Element(queue=w1551, element=CTL_Control_States."Prepare loaded data playback", error in (no error)=w1553) -> (queue out=w1550:refnum<queue>, error out=w1552:errorcluster)  [unwired: 1 in, 1 out]
        n859 = Enqueue Element(queue=w1550, element=CTL_Control_States."Timeline update", error in (no error)=w1552) -> (queue out=w1542:refnum<queue>, error out=w1541:errorcluster)  [unwired: 1 in, 1 out]
        n860 = Enqueue Element(queue=w1542, element=CTL_Control_States."Overlay tracks update", error in (no error)=w1541) -> (queue out=w1543:refnum<queue>, error out=w1545:errorcluster)  [unwired: 1 in, 1 out]
        n861 = Enqueue Element(queue=w1543, element=CTL_Control_States."Location map update", error in (no error)=w1545) -> (queue out=w1547:refnum<queue>, error out=w1548:errorcluster)  [unwired: 1 in, 1 out]
        n862 = Enqueue Element(queue=w1547, element=CTL_Control_States."Speed map update", error in (no error)=w1548) -> (queue out=w1539:refnum<queue>, error out=w1540:errorcluster)  [unwired: 1 in, 1 out]
      }
      frame "Save density map(s)" {
        n863 = local read "Overlays cluster"() -> (w1581:T27)
        n864 = global read "SW_Globals_2.2+.vi" "Paths"() -> (w1615:T77)
        n865 = call <vilib>:"Set Busy.vi"("error in (no error)"=w1586) -> ("error out"=w1571:errorcluster)  [unwired: 9 in, 1 out]
        n866 = call "Get Layout Image as Array.vi"("error in (no error)"=w1571) -> ("error out"=w1569:errorcluster, "Reply Payload"=w1573:T84)  [unwired: 8 in, 1 out]
        n867 = Merge Errors(w1571, w1569) -> (w1570:errorcluster)
        n868 = Unbundle By Name(w1581) -> ("Location density map image"=w1579:u32[][], "Speed density map image"=w1576:u32[][])
        n869 = Unbundle By Name(w1573) -> ("Layout image array (U32)"=w1572:u32[][])
        n870 = Unbundle By Name(w1615) -> ("Density map matrix (time)"=w1595:path, "Density map matrix (speed)"=w1585:path, "Density map picture (time)"=w1583:path, "Density map picture (speed)"=w1582:path)
        n871 = Unbundle By Name(w1581) -> ("Location density map"=w1591:dbl[][], "Speed density map"=w1584:dbl[][])
        n872 = call <vilib>:"Check if File or Folder Exists.vi"("error in (no error)"=w1570, "path"=w1595) -> ("error out"=w1603:errorcluster, "file or folder exists?"=w1614:bool, "dup path"=w1613:path)  [unwired: 7 in]
        n873 = call <vilib>:"Check if File or Folder Exists.vi"("error in (no error)"=w1570, "path"=w1585) -> ("error out"=w1602:errorcluster, "file or folder exists?"=w1607:bool, "dup path"=w1604:path)  [unwired: 7 in]
        n874 = call <vilib>:"Check if File or Folder Exists.vi"("error in (no error)"=w1570, "path"=w1583) -> ("error out"=w1594:errorcluster, "file or folder exists?"=w1598:bool, "dup path"=w1592:path)  [unwired: 7 in]
        n875 = call <vilib>:"Check if File or Folder Exists.vi"("error in (no error)"=w1570, "path"=w1582) -> ("error out"=w1577:errorcluster, "file or folder exists?"=w1587:bool, "dup path"=w1575:path)  [unwired: 7 in]
        n876 = Not(x=w1614) -> (.not. x?=w1612:bool)
        n877 = Not(x=w1607) -> (.not. x?=w1608:bool)
        n878 = Not(x=w1598) -> (.not. x?=w1597:bool)
        n879 = Not(x=w1587) -> (.not. x?=w1588:bool)
        n880 = call-poly <userlib>:"Valid Path__ogtk.vi"("path"=w1595) -> ("valid"=w1610:bool)
        n881 = call-poly <userlib>:"Valid Path__ogtk.vi"("path"=w1585) -> ("valid"=w1609:bool)
        n882 = call-poly <userlib>:"Valid Path__ogtk.vi"("path"=w1583) -> ("valid"=w1596:bool)
        n883 = call-poly <userlib>:"Valid Path__ogtk.vi"("path"=w1582) -> ("valid"=w1589:bool)
        n884 = And(x=w1612, y=w1610) -> (x .and. y?=w1611:bool)
        n885 = And(x=w1608, y=w1609) -> (x .and. y?=w1605:bool)
        n886 = And(x=w1597, y=w1596) -> (x .and. y?=w1593:bool)
        n887 = And(x=w1588, y=w1589) -> (x .and. y?=w1578:bool)
        n888 = case shown="True" w1611 {
          tunnel: w1613 -> [_ w1646]
          tunnel: w1591 -> [_ w1645]
          tunnel: w1603 -> [w1642 w1644]
          tunnel: [w1642 w1643] -> w1601
          frame False {
          }
          frame True {
            n889 = call-poly <vilib>:"Write Delimited Spreadsheet.vi"("file path (dialog if empty)"=w1646, "2D data"=w1645, "error in (no error)"=w1644) -> ("error out"=w1643:errorcluster)  [unwired: 11 in, 1 out]
          }
        }
        n890 = case shown="True" w1605 {
          tunnel: w1604 -> [_ w1641]
          tunnel: w1584 -> [_ w1640]
          tunnel: w1602 -> [w1637 w1639]
          tunnel: [w1637 w1638] -> w1600
          frame False {
          }
          frame True {
            n891 = call-poly <vilib>:"Write Delimited Spreadsheet.vi"("file path (dialog if empty)"=w1641, "2D data"=w1640, "error in (no error)"=w1639) -> ("error out"=w1638:errorcluster)  [unwired: 11 in, 1 out]
          }
        }
        n892 = case shown="True" w1593 {
          tunnel: w1594 -> [w1627 w1634]
          tunnel: [w1627 w1635] -> w1590
          tunnel: w1592 -> [_ w1636]
          tunnel: w1579 -> [_ w1632]
          tunnel: w1572 -> [_ w1633]
          frame False {
          }
          frame True {
            n893 = call "SW_Create_Images_overlay.vi"("Blend factor"=0.15, "Background color"=u32 16777216, "Overlay Image"=w1632, "Background image"=w1633) -> ("Output Image"=w1631:u32[][])  [unwired: 1 in, 1 out]
            n894 = call <vilib>:"Flatten Pixmap.vi"("24-bit pixmap"=w1631) -> ("image data"=w1630:T85)  [unwired: 10 in]
            n895 = call <vilib>:"Write PNG File.vi"("error in (no error)"=w1634, "image data"=w1630, "path to PNG file"=w1636) -> ("error out"=w1635:errorcluster)  [unwired: 7 in, 1 out]
          }
        }
        n896 = case shown="True" w1578 {
          tunnel: w1577 -> [w1617 w1624]
          tunnel: [w1617 w1625] -> w1574
          tunnel: w1575 -> [_ w1626]
          tunnel: w1576 -> [_ w1622]
          tunnel: w1572 -> [_ w1623]
          frame False {
          }
          frame True {
            n897 = call "SW_Create_Images_overlay.vi"("Blend factor"=0.07, "Background color"=u32 16777216, "Overlay Image"=w1622, "Background image"=w1623) -> ("Output Image"=w1621:u32[][])  [unwired: 1 in, 1 out]
            n898 = call <vilib>:"Flatten Pixmap.vi"("24-bit pixmap"=w1621) -> ("image data"=w1620:T85)  [unwired: 10 in]
            n899 = call <vilib>:"Write PNG File.vi"("error in (no error)"=w1624, "image data"=w1620, "path to PNG file"=w1626) -> ("error out"=w1625:errorcluster)  [unwired: 7 in, 1 out]
          }
        }
        n900 = Merge Errors(w1601, w1600, w1590, w1574) -> (w1599:errorcluster)
        n901 = call <vilib>:"Unset Busy.vi"("error in (no error)"=w1599) -> ("error out"=w1580:errorcluster)  [unwired: 10 in]
      }
      frame "Upd. FPS" {
        n902 = Get Notifier Status(notifier=w1659, error in (no error)=w1658) -> (notifier out=w1649:refnum<notifier>, current notification=w1657:T46, error out=w1651:errorcluster)  [unwired: 2 out]
        n903 = Unbundle By Name(w1657) -> ("Acq. is ON"=w1653:bool, "Offline mode"=w1656:bool)
        n904 = Not(x=w1656) -> (.not. x?=w1655:bool)
        n905 = Not(x=w1653) -> (.not. x?=w1652:bool)
        n906 = And(x=w1652, y=w1655) -> (x .and. y?=w1654:bool)
        n907 = case shown="True" w1654 {
          tunnel: w1651 -> [w1661 w1676]
          tunnel: [w1661 w1666] -> w1650
          tunnel: w1648 -> [w1660 w1672]
          tunnel: [w1660 w1665] -> w1647
          frame False {
          }
          frame True {
            # "Change FPS while device is online, but acqusition is stopped."
            n908 = global read "SW_Globals_2.2+.vi" "Settings cluster"() -> (w1662:T16)
            n909 = Unbundle By Name(w1662) -> ("Defaults.VISA Resource Name"=w1681:string, "Recording and saving.Acquisition FPS"=w1680:T18)
            n910 = local read "Sensor board size"() -> (w1679:string)
            n911 = local read "FPS status"() -> (w1678:i32)
            n912 = call "LL_Set_FPS_on_device.vi"("VISA in"=w1681, "Desired FPS"=w1680, "Sensor board size"=w1679, "Current FPS"=w1678, "Error in (no error)"=w1676) -> ("FPS set on device"=w1677:i32, "Error out"=w1675:errorcluster)  [unwired: 9 in, 4 out]
            n913 = local write "FPS status"(w1677) -> ()
            n914 = call "Calibration will be executed"("error in (no error)"=w1675, "Enable"=TRUE) -> ("error out"=w1673:errorcluster)  [unwired: 8 in, 1 out]
            n915 = Enqueue Element(queue=w1672, element=CTL_Control_States."Play Stop", error in (no error)=w1673) -> (queue out=w1669:refnum<queue>, error out=w1668:errorcluster)  [unwired: 1 in, 1 out]
            n916 = Enqueue Element(queue=w1669, element=CTL_Control_States."Play Start", error in (no error)=w1668) -> (queue out=w1664:refnum<queue>, error out=w1667:errorcluster)  [unwired: 1 in, 1 out]
            n917 = Enqueue Element(queue=w1664, element=CTL_Control_States."Timings calibration start", error in (no error)=w1667) -> (queue out=w1665:refnum<queue>, error out=w1666:errorcluster)  [unwired: 1 in, 1 out]
          }
        }
      }
      frame "Upd. trace length" {
        (unwired) u32[] [14308646, 16156991, 16694328, 14206596, 6913947] ("Initial colors ramp array")
        w1684 = T86 [255, 65535, 6618880, 16776960, 16744448, 16711680] ("Initial colors ramp array")
        n918 = global read "SW_Globals_2.2+.vi" "All references"() -> (w1711:T36)
        n919 = local read "UI update period"() -> (w1709:i64)
        n920 = Unbundle By Name(w1711) -> ("Controls references.Trace, s"=w1710:refnum<vi>, "Controls references.Rainbow (time)"=w1702:refnum<vi>, "Controls references.Rainbow (speed)"=w1696:refnum<vi>)
        n921 = To Double Precision Float(number=i64 1000 ("x")) -> (double precision float=w1698:dbl)
        n922 = To Double Precision Float(number=w1709) -> (double precision float=w1697:dbl)
        n923 = Divide(x=w1698, y=w1697) -> (x/y=w1706:dbl)
        n924 = property class="Slide (strict)"(reference=w1710, error in=w1704) -> (error out=w1695:errorcluster, "Value"=w1707:u16)  [unwired: 1 out]
        n925 = Multiply(x=w1707, y=w1706) -> (x*y=w1705:dbl)
        n926 = To Unsigned Word Integer(number=w1705) -> (unsigned 16bit integer=w1689:u16)
        n927 = property class="Bool (strict)"(reference=w1696, error in=w1695) -> (error out=w1694:errorcluster, "Value"=w1687:bool)  [unwired: 1 out]
        n928 = Select(t=w1684, s=w1687, f=w1684) -> (s? t:f=w1691:T86)
        n929 = Select(t=u16 300, s=w1687, f=w1689) -> (s? t:f=w1693:u16)
        n930 = call "GEN_Colors_positions.vi"("Highest color position"=w1693, "Initial colors ramp array in"=w1691) -> ("Colors positions"=w1682:dbl[])  [unwired: 1 out]
        n931 = property class="Bool (strict)"(reference=w1702, error in=w1695) -> (error out=w1700:errorcluster, "Value"=w1699:bool)  [unwired: 1 out]
        n932 = call "SW_Generate_Color_Ramp.vi"("Colors rel. pos."=w1682, "Colors array"=w1691) -> ("Colors array"=w1686:u32[])
        n933 = local write "Trace length, samples"(w1689) -> ()
        n934 = local write "Colors array"(w1686) -> ()
        n935 = Or(x=w1699, y=w1687) -> (x .or. y?=w1688:bool)
        n936 = local write "Rainbow track"(w1688) -> ()
        n937 = local write "Rainbow is speed"(w1687) -> ()
        n938 = Merge Errors(w1695, w1700, w1694) -> (w1701:errorcluster)
        n939 = local read "Mouse drawing parameters"() -> (w1690:T2)
        n940 = Bundle By Name(cluster=w1690, "Trace length, samples"=w1689, "Rainbow track"=w1688, "Rainbow track is speed"=w1687, "Colors array"=w1686) -> (w1685:T2)
        n941 = local write "Mouse drawing parameters"(w1685) -> ()
      }
      frame "Timings calibration start" {
        n942 = Get Notifier Status(notifier=w1719, error in (no error)=w1718) -> (notifier out=w1717:refnum<notifier>, current notification=w1713:T46, error out=w1720:errorcluster)  [unwired: 2 out]
        n943 = Unbundle By Name(w1713) -> ("Offline mode"=w1716:bool)
        n944 = case shown="False" w1716 {
          tunnel: w1720 -> [w1734 w1736]
          tunnel: [w1723 w1736] -> w1715
          tunnel: w1717 -> [w1733 w1735]
          tunnel: [w1722 w1735] -> w1714
          tunnel: w1713 -> [w1732 _]
          frame False {
            # "This part is running when working online"
            n945 = call <vilib>:"Set Busy.vi"("error in (no error)"=w1734) -> ("error out"=w1729:errorcluster)  [unwired: 9 in, 1 out]
            n946 = local read "Calibration samples"() -> (w1721:i32)
            n947 = Bundle By Name(cluster=w1732, "Calibration mode"=TRUE) -> (w1730:T46)
            n948 = call <vilib>:"Launch Progress Bar.vi"("error in (no error)"=w1729, "Enable Cancellation? (T)"=FALSE, "Main Title (\"Working...\")"="Collecting samples..." ("Main Title (\"Working...\")"), "Total Count"=w1721) -> ("error out"=w1728:errorcluster, "Progress Bar Dialog"=w1724:refnum<class "Progress Bar Dialog.lvclass">)  [unwired: 6 in]
            n949 = local write "Progress Bar Dialog"(w1724) -> ()
            n950 = call "550 ms delay"("error in (no error)"=w1728) -> ("error out"=w1725:errorcluster)  [unwired: 10 in]
            n951 = Send Notification(notification=w1730, notifier=w1733, error in (no error)=w1725) -> (notifier out=w1722:refnum<notifier>, error out=w1723:errorcluster)
          }
          frame True {
            # "This part is running when working with the recorded data"
          }
        }
      }
      frame "Timings calibration finish" {
        n952 = Get Notifier Status(notifier=w1745, error in (no error)=w1744) -> (notifier out=w1743:refnum<notifier>, current notification=w1739:T46, error out=w1746:errorcluster)  [unwired: 2 out]
        n953 = Unbundle By Name(w1739) -> ("Stop and Exit"=w1742:bool)
        n954 = case shown="False" w1742 {
          tunnel: w1746 -> [w1771 w1774]
          tunnel: [w1770 w1774] -> w1741
          tunnel: w1743 -> [w1753 w1773]
          tunnel: [w1750 w1773] -> w1740
          tunnel: w1739 -> [w1749 _]
          tunnel: w1738 -> [w1760 w1772]
          tunnel: [w1759 w1772] -> w1737
          frame False {
            # "This part is running when working online"
            n955 = local read "Progress Bar Dialog"() -> (w1765:refnum<class "Progress Bar Dialog.lvclass">)
            n956 = local read "Calibration HW timings"() -> (w1768:u32[])
            n957 = local read "Calibration SW timings"() -> (w1767:dbl[])
            n958 = global read "SW_Globals_2.2+.vi" "Settings cluster"() -> (w1755:T16)
            n959 = global read "SW_Globals_2.2+.vi" "Paths"() -> (w1766:T77)
            n960 = Unbundle By Name(w1766) -> ("Program settings"=w1764:path)
            n961 = call <vilib>:"Close Progress Bar.vi"("error in (no error)"=w1771, "Progress Bar Dialog"=w1765) -> ("error out"=w1769:errorcluster)  [unwired: 9 in]
            n962 = call "HW_Timings_Calibration.vi"("Error In"=w1769, "Calibration SW timings"=w1767, "Calibration HW timings"=w1768, "Settings cluster in"=w1755) -> ("Error out"=w1762:T41, "Settings cluster out"=w1756:T16)  [unwired: 1 out]
            n963 = call "SW_Save_Settings_2.vi"("error in (no error)"=w1762, "Parameter group to save"=T61 "Calibration", "Settings cluster"=w1756, "Settings path in"=w1764) -> ("error out"=w1763:errorcluster)  [unwired: 5 in, 1 out]
            n964 = Unbundle By Name(w1756) -> ("Calibration parameters"=w1761:T23, "Calibration parameters.True frame time, s"=w1754:dbl)
            n965 = Bundle By Name(cluster=w1749, "Calibration mode"=FALSE) -> (w1748:T46)
            n966 = global write "SW_Globals_2.2+.vi" "Settings cluster"(w1756) -> ()
            n967 = local write "Settings cluster (local)"(w1756) -> ()
            n968 = local write "Calibration parameters"(w1761) -> ()
            n969 = Enqueue Element(queue=w1760, element=CTL_Control_States."Update filter", error in (no error)=w1763) -> (queue out=w1759:refnum<queue>, error out=w1752:errorcluster)  [unwired: 1 in, 1 out]
            n970 = local write "Act. frame time, s"(w1754) -> ()
            n971 = Send Notification(notification=w1748, notifier=w1753, error in (no error)=w1752) -> (notifier out=w1750:refnum<notifier>, error out=w1751:errorcluster)
            n972 = call <vilib>:"Unset Busy.vi"("error in (no error)"=w1751) -> ("error out"=w1770:errorcluster)  [unwired: 10 in]
          }
          frame True {
            # "This part is running when working with the recorded data"
          }
        }
      }
      frame "Dispension calibration" {
        n973 = global read "SW_Globals_2.2+.vi" "Settings cluster"() -> (w1775:T16)
        n974 = call "SW_Dispension_Calibration.vi"("error in (no error)"=w1783, "Settings cluster in"=w1775) -> ("error out"=w1777:errorcluster, "Settings cluster out"=w1776:T16)  [unwired: 8 in]
        n975 = global write "SW_Globals_2.2+.vi" "Settings cluster"(w1776) -> ()
        n976 = local write "Settings cluster (local)"(w1776) -> ()
        n977 = global read "SW_Globals_2.2+.vi" "Paths"() -> (w1782:T77)
        n978 = Unbundle By Name(w1782) -> ("Program settings"=w1780:path)
        n979 = Unbundle By Name(w1776) -> ("Calibration parameters"=w1781:T23)
        n980 = local write "Calibration parameters"(w1781) -> ()
        n981 = call "SW_Save_Settings_2.vi"("error in (no error)"=w1777, "Parameter group to save"=T61 "Calibration", "Settings cluster"=w1776, "Settings path in"=w1780) -> ("error out"=w1778:errorcluster)  [unwired: 5 in, 1 out]
      }
      frame "Add Reward condition" {
        n982 = local read "Settings cluster (local)"() -> (w1789:T16)
        n983 = local read "Array of conditions"() -> (w1802:T6)
        n984 = control-ref of="Reward and stimulation"() -> (w1799:refnum<vi>)
        n985 = local read "Calibration parameters"() -> (w1800:T23)
        n986 = Unbundle By Name(w1789) -> ("IO parameters"=w1788:T22)
        n987 = call "SW_Add_or_Modify_Reward_Condition.vi"("IO parameters cluster"=w1788, "Add or Modify?"=enum16{"Add", "Modify"}."Add", "error in (no error)"=w1803, "Main Tree Control in"=w1799, "Calibration parameters"=w1800, "Array of conditions in"=w1802) -> ("error out"=w1801:T41, "Main Tree Control out"=w1798:refnum<vi>, "Array of conditions out"=w1791:T6)  [unwired: 3 in]
        n988 = call "DATA_Reorder_after_condition_modification.vi"("Array of conditions"=w1791) -> ("Reordered conditions array"=w1790:T7[])  [unwired: 2 in]
        n989 = Bundle By Name(cluster=w1789, "Conditions presets array"=w1790) -> (w1786:T16)
        n990 = local write "Array of conditions"(w1790) -> ()
        n991 = call "SW_Generate_Full_Condition(s)_text.vi"("error in (no error)"=w1801, "Array of conditions in"=w1790, "Calibration parameters"=w1800, "TreeControl ref in"=w1798) -> ("error out"=w1796:errorcluster)  [unwired: 6 in, 1 out]
        n992 = Enqueue Element(queue=w1795, element=CTL_Control_States."Check Reward condition(s)", error in (no error)=w1796) -> (queue out=w1794:refnum<queue>, error out=w1793:errorcluster)  [unwired: 1 in, 1 out]
        n993 = call "Set Parameters and data.vi"("Data"=w1786, "Parameter"=CTL_Parameter_transfer_name."All parameters") -> ()  [unwired: 9 in, 1 out]
        n994 = local write "Settings cluster (local)"(w1786) -> ()
        n995 = global write "SW_Globals_2.2+.vi" "Settings cluster"(w1786) -> ()
      }
      frame "Modify Reward condition" {
        n996 = local read "Array of conditions"() -> (w1827:T6)
        n997 = control-ref of="Reward and stimulation"() -> (w1825:refnum<vi>)
        n998 = local read "Calibration parameters"() -> (w1817:T23)
        n999 = local read "Settings cluster (local)"() -> (w1816:T16)
        n1000 = Unbundle By Name(w1816) -> ("IO parameters"=w1815:T22)
        n1001 = call "SW_Add_or_Modify_Reward_Condition.vi"("IO parameters cluster"=w1815, "Add or Modify?"=enum16{"Add", "Modify"}."Modify", "error in (no error)"=w1828, "Main Tree Control in"=w1825, "Calibration parameters"=w1817, "Array of conditions in"=w1827) -> ("error out"=w1826:T41, "Main Tree Control out"=w1824:refnum<vi>, "Array of conditions out"=w1819:T6)  [unwired: 3 in]
        n1002 = call "DATA_Reorder_after_condition_modification.vi"("Array of conditions"=w1819) -> ("Reordered conditions array"=w1818:T7[])  [unwired: 2 in]
        n1003 = Bundle By Name(cluster=w1816, "Conditions presets array"=w1818) -> (w1806:T16)
        n1004 = call "SW_Generate_Full_Condition(s)_text.vi"("error in (no error)"=w1826, "Array of conditions in"=w1818, "Calibration parameters"=w1817, "TreeControl ref in"=w1824) -> ("error out"=w1813:errorcluster, "TreeControl ref out"=w1814:refnum<vi>)  [unwired: 6 in]
        n1005 = local write "Array of conditions"(w1818) -> ()
        n1006 = property class="Tree (strict)"(reference=w1814, error in=w1813) -> (reference out=w1809:refnum<vi>, error out=w1810:errorcluster, "TopLeft"=w1808:T87)
        n1007 = Unbundle By Name(w1808) -> ("Node"=w1807:string)
        n1008 = local write "Settings cluster (local)"(w1806) -> ()
        n1009 = global write "SW_Globals_2.2+.vi" "Settings cluster"(w1806) -> ()
        n1010 = call "Set Parameters and data.vi"("Data"=w1806, "Parameter"=CTL_Parameter_transfer_name."All parameters") -> ()  [unwired: 9 in, 1 out]
        n1011 = property class="Tree (strict)"(reference=w1809, error in=w1810, "Value"=w1807) -> (error out=w1811:errorcluster)  [unwired: 1 out]
        n1012 = Enqueue Element(queue=w1821, element=CTL_Control_States."Check Reward condition(s)", error in (no error)=w1811) -> (queue out=w1820:refnum<queue>, error out=w1812:errorcluster)  [unwired: 1 in, 1 out]
      }
      frame "Delete Reward condition" {
        n1013 = local read "Array of conditions"() -> (w1844:T6)
        n1014 = control-ref of="Reward and stimulation"() -> (w1850:refnum<vi>)
        n1015 = local read "Calibration parameters"() -> (w1852:T23)
        n1016 = call "SW_Init_Array_of_Conditions.vi"("error in (no error)"=w1847) -> ("error out"=w1845:T41, "Array of conditions"=w1846:T6)  [unwired: 1 in]
        n1017 = local read "Settings cluster (local)"() -> (w1851:T16)
        n1018 = call "GET_Index_of_selected_Tree_element_and_N_Conditions.vi"("error in (no error)"=w1845, "TreeControl in"=w1850) -> ("error out"=w1848:errorcluster, "Index of selected element"=w1843:i32, "TreeControl out"=w1849:refnum<vi>)  [unwired: 6 in, 1 out]
        n1019 = Index Array(array=w1846, index=w1843) -> (element=w1842:T7)
        n1020 = Replace Array Subset(array=w1844, new element=w1842, index=w1843) -> (w1841:T6)
        n1021 = call "DATA_Reorder_after_condition_modification.vi"("Array of conditions"=w1841) -> ("Reordered conditions array"=w1840:T7[])  [unwired: 2 in]
        n1022 = call "SW_Generate_Full_Condition(s)_text.vi"("error in (no error)"=w1848, "Array of conditions in"=w1840, "Calibration parameters"=w1852, "TreeControl ref in"=w1849) -> ("error out"=w1834:errorcluster, "TreeControl ref out"=w1835:refnum<vi>)  [unwired: 6 in]
        n1023 = Bundle By Name(cluster=w1851, "Conditions presets array"=w1840) -> (w1831:T16)
        n1024 = local write "Array of conditions"(w1840) -> ()
        n1025 = property class="Tree (strict)"(reference=w1835, error in=w1834, "Value"="") -> (error out=w1833:errorcluster)  [unwired: 1 out]
        n1026 = local write "Settings cluster (local)"(w1831) -> ()
        n1027 = global write "SW_Globals_2.2+.vi" "Settings cluster"(w1831) -> ()
        n1028 = Enqueue Element(queue=w1837, element=CTL_Control_States."Check Reward condition(s)", error in (no error)=w1833) -> (queue out=w1836:refnum<queue>, error out=w1838:errorcluster)  [unwired: 1 in, 1 out]
        n1029 = call "Set Parameters and data.vi"("Data"=w1831, "Parameter"=CTL_Parameter_transfer_name."All parameters") -> ()  [unwired: 9 in, 1 out]
      }
      frame "Check Reward condition(s)" {
        n1030 = control-ref of="Reward and stimulation"() -> (w1864:refnum<vi>)
        n1031 = call "GET_Index_of_selected_Tree_element_and_N_Conditions.vi"("error in (no error)"=w1863, "TreeControl in"=w1864) -> ("error out"=w1856:errorcluster, "Index of selected element"=w1862:i32, "Amount of conditions"=w1854:i32)  [unwired: 6 in, 1 out]
        n1032 = Greater Than 0?(x=w1854) -> (x > 0?=w1861:bool)
        n1033 = Greater Or Equal To 0?(x=w1862) -> (x >= 0?=w1860:bool)
        n1034 = Build Array(w1861, w1860) -> (w1859:bool[])
        n1035 = Boolean Array To Number(Boolean array=w1859) -> (number=w1858:u32)
        n1036 = To Long Integer(number=w1858) -> (32bit integer=w1855:i32)
        n1037 = case shown="3" w1855 {
          selector: w1855 -> [w1867 w1874 _]
          tunnel: w1854 -> [_ _ w1881]
          frame 0, Default {
            # "No elements selected, array is empty"
            n1038 = feedback-in #4(w1867) -> ()
            n1039 = feedback #4(-1) -> (w1868:i32)
            n1040 = Not Equal?(x=w1868, y=w1867) -> (x != y?=w1866:bool)
            n1041 = case shown="True" w1866 {
              frame False {
              }
              frame True {
                n1042 = property on="Add Reward" class="Bool (strict)"("DisabledEnum"=T63."Enabled" ("Disabled")) -> ()  [unwired: 2 in, 2 out]
                n1043 = property on="Modify Reward" class="Bool (strict)"("DisabledEnum"=T63."Disabled and Grayed Out" ("Disabled")) -> ()  [unwired: 2 in, 2 out]
                n1044 = property on="Remove Reward" class="Bool (strict)"("DisabledEnum"=T63."Disabled and Grayed Out" ("Disabled")) -> ()  [unwired: 2 in, 2 out]
              }
            }
          }
          frame 1 {
            # "No elements selected, array is not empty"
            n1045 = feedback-in #5(w1874) -> ()
            n1046 = feedback #5(-1) -> (w1875:i32)
            n1047 = Not Equal?(x=w1875, y=w1874) -> (x != y?=w1873:bool)
            n1048 = case shown="True" w1873 {
              frame False {
              }
              frame True {
                n1049 = property on="Add Reward" class="Bool (strict)"("DisabledEnum"=T63."Disabled and Grayed Out" ("f")) -> ()  [unwired: 2 in, 2 out]
                n1050 = property on="Modify Reward" class="Bool (strict)"("DisabledEnum"=T63."Disabled and Grayed Out" ("Disabled")) -> ()  [unwired: 2 in, 2 out]
                n1051 = property on="Remove Reward" class="Bool (strict)"("DisabledEnum"=T63."Disabled and Grayed Out" ("Disabled")) -> ()  [unwired: 2 in, 2 out]
              }
            }
          }
          frame 3 {
            # "Element selected, array is not empty"
            n1052 = case shown="True" TRUE {
              tunnel: w1881 -> [_ w1887]
              frame False {
              }
              frame True {
                w1886 = 9  # Max number of conditions
                n1053 = Less?(x=w1887, y=w1886) -> (x < y?=w1885:bool)
                n1054 = Select(t=T63."Enabled" ("Disabled"), s=w1885, f=T63."Disabled and Grayed Out") -> (s? t:f=w1883:T63)
                n1055 = property on="Add Reward" class="Bool (strict)"("DisabledEnum"=w1883) -> ()  [unwired: 2 in, 2 out]
                n1056 = property on="Modify Reward" class="Bool (strict)"("DisabledEnum"=T63."Enabled" ("Disabled")) -> ()  [unwired: 2 in, 2 out]
                n1057 = property on="Remove Reward" class="Bool (strict)"("DisabledEnum"=T63."Enabled" ("Disabled")) -> ()  [unwired: 2 in, 2 out]
              }
            }
          }
        }
      }
      frame "Save all settings" {
        n1058 = global read "SW_Globals_2.2+.vi" "Paths"() -> (w1896:T77)
        n1059 = Unbundle By Name(w1896) -> ("Program settings"=w1895:path)
        n1060 = global read "SW_Globals_2.2+.vi" "Settings cluster"() -> (w1892:T16)
        n1061 = call "SW_Save_Settings_2.vi"("error in (no error)"=w1890, "Parameter group to save"=T61 "All", "Settings cluster"=w1892, "Settings path in"=w1895) -> ("error out"=w1894:errorcluster)  [unwired: 5 in, 1 out]
      }
      frame "Save all settings to custom location" {
        n1062 = global read "SW_Globals_2.2+.vi" "Paths"() -> (w1906:T77)
        n1063 = call <vilib>:"Set Busy.vi"("error in (no error)"=w1912) -> ("error out"=w1907:errorcluster)  [unwired: 9 in, 1 out]
        n1064 = Unbundle By Name(w1906) -> ("Folder"=w1905:path)
        n1065 = Strip Path(path=w1905) -> (stripped path=w1904:path)  [unwired: 1 out]
        n1066 = call "Save all settings"("start path"=w1904, "prompt"="Please enter save name and location", "button label"="Save", "default name"="Custom_settings", "error in"=w1907, "pattern (all files)"="*.trset", "pattern label"="Tracker settings") -> ("selected path"=w1910:path, "cancelled"=w1898:bool, "error out"=w1909:errorcluster)  [unwired: 5 in, 1 out]
        n1067 = case shown="No Error" w1909 {
          selector: w1909 -> [w1918 w1929]
          tunnel: [w1921 w1928] -> w1913
          tunnel: w1910 -> [w1920 _]
          tunnel: w1898 -> [w1915 _]
          frame No Error {
            n1068 = call-poly <userlib>:"Valid Path__ogtk.vi"("path"=w1920) -> ("valid"=w1919:bool)
            n1069 = Not(x=w1915) -> (.not. x?=w1916:bool)
            n1070 = And(x=w1916, y=w1919) -> (x .and. y?=w1917:bool)
            n1071 = case shown="True" w1917 {
              tunnel: [w1922 w1927] -> w1921
              tunnel: w1920 -> [_ w1924]
              tunnel: w1918 -> [w1922 w1923]
              frame False {
              }
              frame True {
                n1072 = global read "SW_Globals_2.2+.vi" "Settings cluster"() -> (w1925:T16)
                n1073 = call "SW_Save_Settings_2.vi"("error in (no error)"=w1923, "Parameter group to save"=T61 "All", "Settings cluster"=w1925, "Settings path in"=w1924) -> ("error out"=w1927:errorcluster)  [unwired: 5 in, 1 out]
              }
            }
          }
          frame Error {
            n1074 = call <vilib>:"Simple Error Handler.vi"("error in (no error)"=w1929) -> ("error out"=w1930:errorcluster)  [unwired: 4 in, 4 out]
            n1075 = call <vilib>:"Clear Errors.vi"("error in (no error)"=w1930) -> ("error out"=w1928:errorcluster)  [unwired: 5 in, 1 out]
          }
        }
        n1076 = call <vilib>:"Unset Busy.vi"("error in (no error)"=w1913) -> ("error out"=w1911:errorcluster)  [unwired: 10 in]
      }
      frame "Close App" {
        w1932 = 5.0 ("Timeout to Wait for Stop (s) (-1: no timeout)")
        w1957 = T88 128 items=["Flush Receive Buffer"=16, "Write Transmit Buffer to Device"=32, "Flush Receive Buffer (No I/O)"=64, "Flush Transmit Buffer"=128] ("Mask")
        n1077 = global read "SW_Globals_2.2+.vi" "Settings cluster"() -> (w1941:T16)
        n1078 = Unbundle By Name(w1941) -> ("Defaults.VISA Resource Name"=w1946:string)
        n1079 = disable-structure shown="Disabled" {
          disable-tunnel: [w1965 _] -> w1940
          disable-tunnel: w1932 -> [w1964 _]
          frame Disabled {
            n1080 = call "Stop Module.vi"("Timeout to Wait for Stop (s) (-1: no timeout)"=w1964) -> ("error out"=w1965:errorcluster)  [unwired: 10 in]
          }
          frame Enabled {
          }
        }
        n1081 = call "Prepare to Exit.vi"() -> ("error out"=w1938:errorcluster)  [unwired: 11 in]
        n1082 = call "Stop Module.vi"("Timeout to Wait for Stop (s) (-1: no timeout)"=w1932) -> ("error out"=w1937:errorcluster)  [unwired: 10 in]
        n1083 = call "Stop Module.vi"("Timeout to Wait for Stop (s) (-1: no timeout)"=w1932) -> ("error out"=w1931:errorcluster)  [unwired: 10 in]
        n1084 = call "HW_Acquisition_Stop.vi"("Error In"=w1944, "VISA resource name in"=w1946) -> ("Error Out"=w1934:errorcluster, "VISA resource name out"=w1945:refnum<visa-resource-name>)
        n1085 = Merge Errors(w1934, w1940, w1938, w1937, w1931) -> (w1939:errorcluster)
        n1086 = call "1.5s delay"("error in (no error)"=w1939) -> ("error out"=w1933:errorcluster)  [unwired: 10 in]
        n1087 = VISA Flush I/O Buffer(VISA resource name=w1945, mask (16)=w1957, error in (no error)=w1933) -> (VISA resource name out=w1958:refnum<visa-resource-name>, error out=w1959:errorcluster)
        n1088 = VISA Clear(VISA resource name=w1958, error in (no error)=w1959) -> (VISA resource name out=w1961:refnum<visa-resource-name>, error out=w1960:errorcluster)
        n1089 = VISA Close(VISA resource name=w1961, error in (no error)=w1960) -> (error out=w1962:errorcluster)
        n1090 = call <vilib>:"Clear Errors.vi"("error in (no error)"=w1962) -> ("error out"=w1954:errorcluster)  [unwired: 5 in, 1 out]
        n1091 = Get Notifier Status(notifier=w1955, error in (no error)=w1954) -> (notifier out=w1952:refnum<notifier>, current notification=w1951:T46, error out=w1953:errorcluster)  [unwired: 2 out]
        n1092 = Bundle By Name(cluster=w1951, "Stop and Exit"=TRUE) -> (w1950:T46)
        n1093 = Send Notification(notification=w1950, notifier=w1952, error in (no error)=w1953) -> (notifier out=w1948:refnum<notifier>, error out=w1935:errorcluster)
        n1094 = property class="App"() -> ("App.Kind"=w1947:T70)  [unwired: 2 in, 2 out]
        n1095 = call "IMAQ Dispose"("All Images? (No)"=TRUE, "error in (no error)"=w1935) -> ("error out"=w1942:errorcluster)  [unwired: 4 in]
        n1096 = case shown="\"invalid app kind\", Default" w1947 {
          tunnel: w1942 -> [w1967 w1970]
          tunnel: [w1966 w1970] -> w1936
          frame "invalid app kind", Default {
            # "Close FP only if app is compiled"
            n1097 = global read "SW_Globals_2.2+.vi" "All references"() -> (w1969:T36)
            n1098 = Unbundle By Name(w1969) -> ("Service references.This VI"=w1968:refnum<vi>)
            n1099 = invoke class="VI" method="FP.Close"(reference=w1968, error in=w1967) -> (error out=w1966:errorcluster)  [unwired: 1 in, 2 out]
          }
          frame "Development System" {
          }
        }
      }
    }
    n1100 = call "Error (IDL).vi"("Previous step"=w289, "Error In"=w291, "Queue In"=w293) -> ("Error Out"=w290:errorcluster, "Error data"=w288:variant, "Queue Out"=w292:refnum<queue>)  [unwired: 6 in]
    n1101 = node-c288(w290) -> ()  [unwired: 1 out]
  }
  n1102 = node-c288(w19, i64 499 ("Period"), 100 ("Priority"), "Whatchdog" ("Structure Name"), w37) -> (w43:T48)
  n1103 = node-c288(w19, i64 2 ("Period"), 45000 ("Priority"), "Proc_and_save" ("Structure Name"), w24) -> (w35:T48)
  n1104 = node-c288(w19, i64 53 ("Period"), 1000 ("Priority"), "UI_response" ("Structure Name"), w17) -> (w65:T48)
  n1105 = timed-loop {
    timing: w43 -> [_]
    timing-out: [_] -> w42
    tunnel: w22 -> [w2004]
    tunnel: w23 -> [w1993]
    tunnel: w36 -> [w1998]
    stop <- w2001 stop-if-true
    # "Whatchdog and slow stuff loop"
    n1106 = node-c288() -> (w2003:errorcluster, w1999:i64)  [unwired: 1 in]
    n1107 = Get Notifier Status(notifier=w2004, error in (no error)=w2003) -> (current notification=w2002:T46, error out=w2000:errorcluster)  [unwired: 3 out]
    n1108 = local read "UI update period"() -> (w1996:i64)
    n1109 = call "SW_Get_CPU_load.vi"("error in (no error)"=w2000, "Buffer length, sec"=5.0, "Scan interval, ms"=w1999, "CPU monitor .NET reference in"=w1998) -> ("error out"=w1992:errorcluster, "Historical CPU load, %"=w1991:sgl)  [unwired: 2 out]
    n1110 = call "SW_Adjust_UI_draw_interwal.vi"("UI update period (l.v.o.) in"=w1996, "Historical CPU load, %"=w1991) -> ("Updated?"=w1994:bool, "UI update period (l.v.o.) out"=w1995:i64)
    n1111 = Unbundle By Name(w2002) -> ("Stop and Exit"=w2001:bool, "Acq. is ON"=w1987:bool, "Offline mode"=w1988:bool, "Recording now"=w1976:bool)
    n1112 = local write "CPU load"(w1991) -> ()
    n1113 = local write "UI update period"(w1995) -> ()
    n1114 = case shown="True" w1994 {
      tunnel: w1993 -> [w2017 w2022]
      tunnel: w1992 -> [w2018 w2021]
      tunnel: [w2018 w2020] -> w1989
      tunnel: [w2017 w2019] -> w1979
      frame False {
        # "No update"
      }
      frame True {
        # "Update trace length"
        n1115 = Enqueue Element(queue=w2022, element=CTL_Control_States."Upd. trace length", error in (no error)=w2021) -> (queue out=w2019:refnum<queue>, error out=w2020:errorcluster)  [unwired: 1 in, 1 out]
      }
    }
    n1116 = Not(x=w1988) -> (.not. x?=w1986:bool)
    n1117 = And(x=w1987, y=w1986) -> (x .and. y?=w1977:bool)
    n1118 = local read "Since track start"() -> (w1980:dbl)
    n1119 = global read "SW_Globals_2.2+.vi" "All references"() -> (w1990:T36)
    n1120 = global read "SW_Globals_2.2+.vi" "Settings cluster"() -> (w1985:T16)
    n1121 = Unbundle By Name(w1985) -> ("Recording and saving.\"Stop at\" enabled"=w1984:bool, "Recording and saving.Stop at"=w1981:dbl)
    n1122 = call "UI_Set_Slider_values_when_online.vi"("error in (no error)"=w1989, "Online? (F)"=w1977, "Since track start"=w1980, "All references"=w1990) -> ("error out"=w1982:errorcluster)  [unwired: 7 in]
    n1123 = Compound Arithmetic op=AND(w1977, w1976, w1984) -> (w1978:bool)
    n1124 = case shown="True" w1978 {
      tunnel: [w2005 w2006] -> w1983
      tunnel: w1982 -> [w2005 w2008]
      tunnel: w1981 -> [_ w2010]
      tunnel: w1980 -> [_ w2011]
      tunnel: w1979 -> [_ w2007]
      frame False {
      }
      frame True {
        n1125 = Greater Or Equal?(x=w2011, y=w2010) -> (x >= y?=w2009:bool)
        n1126 = case shown="True" w2009 {
          tunnel: [w2012 w2016] -> w2006
          tunnel: w2008 -> [w2012 w2015]
          tunnel: w2007 -> [_ w2014]
          frame False {
          }
          frame True {
            n1127 = Enqueue Element(queue=w2014, element=CTL_Control_States."Stop Recording", error in (no error)=w2015) -> (error out=w2016:errorcluster)  [unwired: 1 in, 2 out]
          }
        }
      }
    }
    n1128 = node-c288(w1983) -> ()  [unwired: 1 out]
  }
  n1129 = timed-loop {
    timing: w35 -> [_]
    timing-out: [_] -> w34
    tunnel: w22 -> [w2048]
    tunnel: w26 -> [w2047]
    tunnel: w23 -> [w2034]
    tunnel: [w2030] -> w25
    stop <- w2031 stop-if-true
    # "Data processing, saving and calibration loop"
    n1130 = node-c288() -> (w2037:errorcluster)  [unwired: 1 in]
    n1131 = call <extravilib>:"Read.vi"("timeout in ms (-1)"=563, "channel"=w2047) -> ("element"=w2039:T51, "timed out?"=w2042:bool, "count"=w2041:i32)  [unwired: 5 in, 2 out]
    n1132 = Get Notifier Status(notifier=w2048, error in (no error)=w2037) -> (notifier out=w2033:refnum<notifier>, current notification=w2032:T46, error out=w2038:errorcluster)  [unwired: 2 out]
    n1133 = Not(x=w2042) -> (.not. x?=w2045:bool)
    n1134 = Equal To 0?(x=w2041) -> (x = 0?=w2044:bool)
    n1135 = Unbundle By Name(w2032) -> ("Stop and Exit"=w2031:bool)
    n1136 = Not(x=w2031) -> (.not. x?=w2043:bool)
    n1137 = Compound Arithmetic op=AND(w2045, w2044, w2043) -> (w2040:bool)
    n1138 = case shown="True" w2040 {
      tunnel: w2039 -> [_ w2059]
      tunnel: w2037 -> [w2049 w2058]
      tunnel: [w2049 w2057] -> w2035
      tunnel: w2034 -> [_ w2056]
      tunnel: w2033 -> [_ w2052]
      tunnel: w2032 -> [_ w2051]
      tunnel: [_ w2050] -> w2030
      frame False {
      }
      frame True {
        n1139 = Unbundle By Name(w2051) -> ("Calibration mode"=w2055:bool)
        n1140 = feedback-in #6(w2055) -> ()
        n1141 = feedback #6(FALSE ("Calibration mode")) -> (w2053:bool)
        n1142 = case shown="False" w2055 {
          tunnel: w2059 -> [w2080 w2096]
          tunnel: w2058 -> [w2081 w2100]
          tunnel: [w2061 w2092] -> w2057
          tunnel: w2056 -> [w2077 w2098]
          tunnel: w2053 -> [_ w2089]
          tunnel: w2052 -> [w2079 w2094]
          tunnel: [w2065 _] -> w2050
          frame False {
            # "Regular samples are recorded/tested here"
            n1143 = local read "IO parameters"() -> (w2082:T22)
            n1144 = call "FL_React_on_incoming_TTLs.vi"("IO parameters in"=w2082, "Data in"=w2080, "Notifier in"=w2079, "Queue in"=w2077, "error in (no error)"=w2081) -> ("TTL received at (HW)"=w2073:u32, "TTL received at (SW)"=w2078:timestamp, "Data out"=w2070:T51, "Notifier out"=w2075:refnum<notifier>, "error out"=w2069:errorcluster)  [unwired: 5 in, 1 out]
            n1145 = local write "TTL in time (SW)"(w2078) -> ()
            n1146 = local write "TTL in time (HW)"(w2073) -> ()
            n1147 = local read "Stats parameters (online)"() -> (w2072:T1)
            n1148 = local read "Reset barplot"() -> (w2071:bool)
            n1149 = call "GET_Statistics_(online).vi"("Animal coordinates in"=w2070, "Stats parameters (online)"=w2072, "Reset? (F)"=w2071, "error in (no error)"=w2069) -> ("Animal coordinates out"=w2063:T51, "error out"=w2068:T41)  [unwired: 3 in]
            n1150 = Get Notifier Status(notifier=w2075, error in (no error)=w2068) -> (current notification=w2076:T89, error out=w2067:errorcluster)  [unwired: 3 out]
            n1151 = Unbundle By Name(w2076) -> ("Recording now"=w2074:bool)
            n1152 = case shown="True" w2074 {
              tunnel: w2067 -> [w2083 w2087]
              tunnel: [w2083 w2084] -> w2062
              tunnel: w2063 -> [_ w2086]
              frame False {
              }
              frame True {
                n1153 = local read "Key_pressed"() -> (w2085:string)
                n1154 = local read "TDMS ref."() -> (w2088:refnum<k34>)
                n1155 = call "PR_Write_tracker_stream_to_TDMS.vi"("error in (no error)"=w2087, "Key_pressed"=w2085, "Data in"=w2086, "TDMS ref. in"=w2088) -> ("error out"=w2084:errorcluster)  [unwired: 6 in, 1 out]
              }
            }
            n1156 = Unbundle By Name(w2063) -> ("Measurements and statistics"=w2066:T52)
            n1157 = call "Send Frame.vi"("error in (no error)"=w2062, "Data in"=w2063) -> ("error out"=w2064:errorcluster)  [unwired: 9 in]
            n1158 = call "Send frame.vi"("error in (no error)"=w2062, "Coordinates and speed"=w2063) -> ("error out"=w2060:errorcluster)  [unwired: 9 in]
            n1159 = call <extravilib>:"Write.vi"("element"=w2066) -> ("channel"=w2065:T90)  [unwired: 8 in, 2 out]
            n1160 = Merge Errors(w2064, w2060) -> (w2061:errorcluster)
          }
          frame True {
            # "Calibration samples acquisition happens here"
            n1161 = local read "Progress Bar Dialog"() -> (w2099:refnum<class "Progress Bar Dialog.lvclass">)
            n1162 = local read "Calibration samples"() -> (w2095:i32)
            n1163 = Not(x=w2089) -> (.not. x?=w2097:bool)
            n1164 = call "FL_Collect_Timings_Data.vi"("Control"=w2098, "Progress Bar Dialog in"=w2099, "States"=w2094, "Calibration buffer length, samples"=w2095, "Reset"=w2097, "error in (no error)"=w2100, "Data in"=w2096) -> ("Calibration HW timings"=w2091:u32[], "Calibration SW timings"=w2090:dbl[], "Done"=w2093:bool, "error out"=w2092:errorcluster)  [unwired: 5 in]
            n1165 = case shown="True" w2093 {
              tunnel: w2091 -> [_ w2102]
              tunnel: w2090 -> [_ w2101]
              frame False {
              }
              frame True {
                n1166 = local write "Calibration HW timings"(w2102) -> ()
                n1167 = local write "Calibration SW timings"(w2101) -> ()
              }
            }
          }
        }
      }
    }
    n1168 = Merge Errors(w2035, w2038) -> (w2036:errorcluster)
    n1169 = node-c288(w2036) -> ()  [unwired: 1 out]
  }
  n1170 = timed-loop {
    timing: w54 -> [_]
    timing-out: [_] -> w53
    tunnel: w23 -> [_]
    tunnel: w22 -> [w2132]
    tunnel: w27 -> [w2131]
    tunnel: w28 -> [w2117]
    tunnel: w25 -> [w2110]
    stop <- w2120 stop-if-true
    # "UI drawings and plots update loop"
    n1171 = node-c288() -> (w2108:errorcluster)  [unwired: 1 in]
    n1172 = Get Notifier Status(notifier=w2132, error in (no error)=w2108) -> (current notification=w2133:T46, error out=w2119:errorcluster)  [unwired: 3 out]
    n1173 = local read "Play/Pause"() -> (w2122:bool)
    n1174 = Unbundle By Name(w2133) -> ("Calibration mode"=w2109:bool, "Updating layout"=w2112:bool, "Offline mode"=w2115:bool, "Data loaded"=w2121:bool, "Stop and Exit"=w2120:bool)
    n1175 = Not(x=w2112) -> (.not. x?=w2111:bool)
    n1176 = Not(x=w2120) -> (.not. x?=w2128:bool)
    n1177 = Select(t=0, s=w2115, f=563 ("timeout in ms (-1)")) -> (s? t:f=w2114:i32)
    n1178 = call <extravilib>:"Read.vi"("channel"=w2131, "timeout in ms (-1)"=w2114) -> ("element"=w2130:T25, "count"=w2124:i32, "timed out?"=w2129:bool)  [unwired: 4 in, 3 out]
    n1179 = Not(x=w2129) -> (.not. x?=w2126:bool)
    n1180 = Equal To 0?(x=w2124) -> (x = 0?=w2127:bool)
    n1181 = Compound Arithmetic op=AND(w2122, w2126, w2127, w2128, w2111) -> (w2125:bool)
    n1182 = case shown="False" w2125 {
      tunnel: w2130 -> [_ w2217]
      tunnel: w2122 -> [w2134 _]
      tunnel: w2121 -> [w2143 _]
      tunnel: w2115 -> [w2142 _]
      tunnel: w2120 -> [w2141 _]
      tunnel: w2119 -> [w2139 w2221]
      tunnel: [w2138 w2220] -> w2118
      tunnel: w2117 -> [w2136 _]
      tunnel: w2111 -> [w2135 _]
      tunnel: w2110 -> [_ w2216]
      tunnel: w2109 -> [_ w2209]
      frame False {
        # "Offline stuff here"
        n1183 = Not(x=w2141) -> (.not. x?=w2140:bool)
        n1184 = Compound Arithmetic op=AND(w2143, w2142, w2140, w2135) -> (w2137:bool)
        n1185 = case shown="True" w2134 {
          tunnel: w2139 -> [w2154 w2191]
          tunnel: [w2153 w2190] -> w2138
          tunnel: w2137 -> [w2147 w2189]
          tunnel: w2136 -> [w2152 _]
          frame True {
            # "Draw this when Play is active"
            n1186 = call <extravilib>:"Read.vi"("channel"=w2152, "timeout in ms (-1)"=563) -> ("element"=w2144:dbl[], "count"=w2149:i32, "timed out?"=w2150:bool)  [unwired: 4 in, 3 out]
            n1187 = Equal To 0?(x=w2149) -> (x = 0?=w2146:bool)
            n1188 = Not(x=w2150) -> (.not. x?=w2145:bool)
            n1189 = Compound Arithmetic op=AND(w2145, w2146, w2147) -> (w2148:bool)
            n1190 = case shown="True" w2148 {
              tunnel: w2154 -> [w2155 w2180]
              tunnel: [w2155 w2184] -> w2153
              tunnel: w2144 -> [_ w2181]
              frame False {
              }
              frame True {
                n1191 = local read "Timeline min&max"() -> (w2178:cluster{"Tl. min":dbl, "TL. max":dbl})
                n1192 = Index Array(array=w2181) -> (element #1=w2158:dbl, element #2=w2174:dbl, element #3=w2173:dbl, element #4=w2172:dbl, element #5=w2160:dbl, element #6=w2167:dbl)  [unwired: 6 in]
                n1193 = Unbundle(w2178) -> ("Tl. min"=w2177:dbl, "TL. max"=w2176:dbl)
                n1194 = To Time Stamp(1:w2158) -> (0:w2169:timestamp)
                n1195 = local write "Since track start"(w2158) -> ()
                n1196 = Build Array(w2160) -> (w2170:dbl[])
                n1197 = Bundle By Name(cluster=T25 {"R from center"=0.0, "phi (mouse angular position in the cage)"=0.0, "alpha (mouse rot. angle)"=0.0, "X"=0.0, "Y"=0.0, "theta (from center towards mouse)"=0.0, "beta (cage rot. against mouse)"=0.0, "w (mouse angle to wall)"=0.0, "Speed (filtered)"=0.0} ("Animal coordinates and speed"), "X"=w2174, "Y"=w2173, "alpha (mouse rot. angle)"=w2172, "Speed (filtered)"=w2160) -> (w2171:T25)
                n1198 = Bundle("Tl. min"=w2177, "TL. max"=w2176, "Numeric"=w2158) -> (w2179:T91)  [unwired: 1 in]
                n1199 = local write "Timeline"(w2179) -> ()
                n1200 = Bundle By Name("t0"=w2169, "Y"=w2170) -> (w2168:waveform(dbl))  [unwired: 1 in]
                n1201 = local read "Diagram (generated)"() -> (w2188:T15)
                n1202 = local read "Reset buffers?"() -> (w2183:bool)
                n1203 = local read "Track show state"() -> (w2186:u32)
                n1204 = local read "Overlays cluster"() -> (w2185:T27)
                n1205 = local write "Mouse speed"(w2168) -> ()
                n1206 = local read "Mouse drawing parameters"() -> (w2156:T2)
                n1207 = local write "Current position"(w2171) -> ()
                n1208 = call "DRAW_Mouse_DAQmx_w_overlay.vi"("Overlay track show state"=w2186, "Reset buffers? (F)"=w2183, "Overlays cluster"=w2185, "Error In (no error)"=w2180, "Mouse position"=w2171, "Mouse drawing parameters"=w2156, "Image In"=w2188) -> ("Error Out"=w2184:errorcluster, "Reset buffers out"=w2182:bool, "Image Out"=w2187:T15)  [unwired: 1 in]
                n1209 = To Byte Integer(number=w2167) -> (8bit integer=w2162:i8)
                n1210 = local write "Diagram (display)"(w2187) -> ()
                n1211 = local write "Mouse speed, mm/s"(w2160) -> ()
                n1212 = local write "Reset buffers?"(w2182) -> ()
                n1213 = Decrement(x=w2162) -> (x-1=w2165:i8)
                n1214 = local read "Start time (SW)"() -> (w2159:timestamp)
                n1215 = Replace Array Subset(array=bool[] [FALSE, FALSE, FALSE, FALSE, FALSE, FALSE, FALSE, FALSE, FALSE, FALSE, FALSE, FALSE, FALSE, FALSE, FALSE, FALSE], new element=TRUE ("new element/subarray"), index=w2165) -> (w2163:bool[])
                n1216 = Add(x=w2158, y=w2159) -> (x+y=w2157:timestamp)
                n1217 = local write "Current Time"(w2157) -> ()
                n1218 = Array To Cluster(array=w2163) -> (cluster=w2161:T92)
                n1219 = local write "Current zone"(w2161) -> ()
              }
            }
          }
          frame False {
            # "Draw this when Play is Off"
            n1220 = case shown="True" w2189 {
              tunnel: w2191 -> [w2194 w2199]
              tunnel: [w2194 w2198] -> w2190
              frame False {
                n1221 = Get Date/Time In Seconds() -> (seconds since 1Jan1904=w2193:timestamp)
                n1222 = local write "Current Time"(w2193) -> ()
                n1223 = Wait Until Next ms Multiple(millisecond multiple=u32 500) -> ()  [unwired: 1 out]
              }
              frame True {
                n1224 = local read "Mouse drawing parameters"() -> (w2204:T2)
                n1225 = local read "Diagram (generated)"() -> (w2203:T15)
                n1226 = local read "Track show state"() -> (w2201:u32)
                n1227 = local read "Overlays cluster"() -> (w2200:T27)
                n1228 = local read "Current position"() -> (w2195:T25)
                n1229 = local read "Reset buffers?"() -> (w2196:bool)
                n1230 = call "DRAW_Mouse_DAQmx_w_overlay.vi"("Overlay track show state"=w2201, "Reset buffers? (F)"=w2196, "Overlays cluster"=w2200, "Error In (no error)"=w2199, "Mouse position"=w2195, "Mouse drawing parameters"=w2204, "Image In"=w2203) -> ("Error Out"=w2198:errorcluster, "Reset buffers out"=w2197:bool, "Image Out"=w2202:T15)  [unwired: 1 in]
                n1231 = local write "Diagram (display)"(w2202) -> ()
                n1232 = local write "Reset buffers?"(w2197) -> ()
              }
            }
          }
        }
      }
      frame True {
        # "Online activities here (Play or Record)"
        n1233 = Not(x=w2209) -> (.not. x?=w2208:bool)
        n1234 = call <extravilib>:"Read.vi"("channel"=w2216, "timeout in ms (-1)"=563) -> ("element"=w2215:T52, "element valid?"=w2214:bool, "timed out?"=w2210:bool)  [unwired: 4 in, 3 out]
        n1235 = Not(x=w2210) -> (.not. x?=w2211:bool)
        n1236 = local read "Mouse drawing parameters"() -> (w2225:T2)
        n1237 = local read "Diagram (generated)"() -> (w2227:T15)
        n1238 = local read "Start time (SW)"() -> (w2223:timestamp)
        n1239 = Compound Arithmetic op=AND(w2214, w2211, w2208) -> (w2212:bool)
        n1240 = Get Date/Time In Seconds() -> (seconds since 1Jan1904=w2205:timestamp)
        n1241 = Subtract(x=w2205, y=w2223) -> (x-y=w2219:dbl)
        n1242 = local write "Since track start"(w2219) -> ()
        n1243 = Unbundle By Name(w2217) -> ("Speed (filtered)"=w2207:dbl)
        n1244 = To Time Stamp(1:w2219) -> (0:w2222:timestamp)
        n1245 = call "SW_Draw_mouse_DAQmx.vi"("Size of the image (480x480)"=T82 {"Numeric Control"=480.0, "Numeric Control"=480.0}, "Error In (no error)"=w2221, "Mouse position"=w2217, "Mouse drawing parameters"=w2225, "Image In"=w2227) -> ("Error Out"=w2220:errorcluster, "Image Out"=w2226:T15)  [unwired: 2 in]
        n1246 = Build Array(w2207) -> (w2224:dbl[])
        n1247 = Bundle By Name("t0"=w2222, "Y"=w2224) -> (w2206:waveform(dbl))  [unwired: 1 in]
        n1248 = case shown="True" w2212 {
          tunnel: w2215 -> [_ w2235]
          tunnel: w2207 -> [_ w2229]
          tunnel: w2206 -> [_ w2234]
          frame False {
          }
          frame True {
            n1249 = Unbundle By Name(w2235) -> ("Zone #"=w2242:i8, "Histogram"=w2239:dbl[], "Running, perc. of time"=w2237:dbl, "Run, meters"=w2236:dbl, "Avg. speed"=w2233:dbl)
            n1250 = local read "Hist. X axis"() -> (w2238:dbl[])
            n1251 = Decrement(x=w2242) -> (x-1=w2246:i8)
            n1252 = local write "Average speed, mm/s"(w2233) -> ()
            n1253 = local write "Running, perc. of time"(w2237) -> ()
            n1254 = Bundle By Name(cluster=T32 {"X Values"=[15.0, 45.0, 75.0, 105.0, 135.0, 165.0, 195.0, 225.0, 255.0, 285.0], "Histogram: h(x)"=[-1.0, -1.0, 0.0, 1.0, 2.0, 1.0, 0.0, -1.0, -1.0, -1.0]} ("XY Graph - Light"), "X Values"=w2238, "Histogram: h(x)"=w2239) -> (w2240:T32)
            n1255 = Replace Array Subset(array=bool[] [FALSE, FALSE, FALSE, FALSE, FALSE, FALSE, FALSE, FALSE, FALSE, FALSE, FALSE, FALSE, FALSE, FALSE, FALSE, FALSE], new element=TRUE ("new element/subarray"), index=w2246) -> (w2244:bool[])
            n1256 = local write "Mouse speed"(w2234) -> ()
            n1257 = Array To Cluster(array=w2244) -> (cluster=w2243:T92)
            n1258 = local write "Histograms"(w2240) -> ()
            n1259 = local write "Current zone"(w2243) -> ()
            n1260 = local write "Run distance, m"(w2236) -> ()
            n1261 = local read "Speed threshold"() -> (w2230:dbl)
            n1262 = Greater?(x=w2229, y=w2230) -> (0:w2228:bool)
            n1263 = Select(t=w2229, s=w2228, f=0.0) -> (s? t:f=w2231:dbl)
            n1264 = local write "Mouse speed, mm/s"(w2231) -> ()
          }
        }
        n1265 = local write "Current Time"(w2205) -> ()
        n1266 = local write "Diagram (display)"(w2226) -> ()
      }
    }
    n1267 = local read "UI update period"() -> (w2123:i64)
    n1268 = node-c288(w2118, w2123) -> ()  [unwired: 1 out]
  }
  n1269 = timed-loop {
    timing: w65 -> [_]
    timing-out: [_] -> w64
    tunnel: w23 -> [w2260]
    tunnel: w22 -> [w2259]
    tunnel: w13 -> [w2255]
    tunnel: [w2254] -> w12
    stop <- w2261 stop-if-true
    # "UI response loop"
    n1270 = node-c288() -> (w2257:errorcluster)  [unwired: 1 in]
    n1271 = event shown="[2] Menu Selection (User)" {
      selector: w2255 -> [_ _ _ _ _ _ _ _ _ _ _ _ _ _ _ _ _ _ _ _ _ _ _ _ _ _ _ _ _]
      dyn-events: [_ _ _ _ _ _ _ _ _ _ _ _ _ _ _ _ _ _ _ _ _ _ _ _ _ _ _ _ _] -> w2254
      timeout: _ -> [_ _ _ _ _ _ _ _ _ _ _ _ _ _ _ _ _ _ _ _ _ _ _ _ _ _ _ _ _]
      tunnel: [_ TRUE w2275 _ _ _ _ _ _ _ _ _ _ _ _ _ _ _ _ _ _ _ _ _ _ _ _ _ _] -> w2261
      tunnel: w2260 -> [_ w2271 w2276 w2376 w2386 w2392 w2406 w2420 w2424 _ w2497 w2522 w2527 w2532 w2537 _ _ w2580 _ w2591 w2626 w2643 w2655 w2657 _ w2668 w2684 _ _]
      tunnel: w2259 -> [_ _ _ _ _ _ _ _ _ _ _ _ _ _ _ _ _ _ _ w2588 w2623 _ _ _ _ _ _ _ _]
      tunnel: w2257 -> [w2263 w2269 w2274 w2369 w2380 w2390 w2404 w2418 w2431 w2464 w2496 w2524 w2529 w2534 w2539 w2548 w2571 w2576 w2581 w2587 w2622 w2641 w2653 w2656 w2663 w2667 w2683 w2686 w2697]
      tunnel: [w2262 w2268 w2273 w2370 w2379 w2389 w2399 w2413 w2422 w2463 w2482 w2523 w2528 w2533 w2538 w2540 w2570 w2577 w2581 w2589 w2624 w2640 w2652 w2659 w2663 w2666 w2680 w2685 w2696] -> w2256
      event Timeout {
        n1272 = event-data() -> ()  [unwired: 1 in, 3 out]
        n1273 = global read "SW_Globals_2.2+.vi" "All references"() -> (w2265:T36)
        n1274 = Get Date/Time In Seconds() -> (seconds since 1Jan1904=w2266:timestamp)
        n1275 = Unbundle By Name(w2265) -> ("Indicators references.Current Time"=w2264:refnum<vi>)
        n1276 = property class="AbsTime (strict)"(reference=w2264, error in=w2263, "Value"=w2266) -> (error out=w2262:errorcluster)  [unwired: 1 out]
      }
      event Panel Close? {
        n1277 = event-data() -> ()  [unwired: 1 in, 4 out]
        n1278 = Enqueue Element(queue=w2271, element=CTL_Control_States."Close App", error in (no error)=w2269) -> (error out=w2268:errorcluster)  [unwired: 1 in, 2 out]
        n1279 = event-data("Discard?"=TRUE) -> ()  [unwired: 1 in, 1 out]
      }
      event Menu Selection (User) {
        n1280 = event-data() -> ("ItemTag"=w2277:string)  [unwired: 1 in, 6 out]
        n1281 = case shown="\"Fix broken track\"" w2277 {
          tunnel: w2276 -> [_ w2281 w2290 w2296 w2305 w2311 w2315 w2319 w2323 w2327 w2331 w2335 w2339 _ w2345 w2349 w2353 _]
          tunnel: [_ TRUE _ _ _ _ _ _ _ _ _ _ _ _ _ _ _ _] -> w2275
          tunnel: w2274 -> [w2278 w2283 w2288 w2297 w2306 w2309 w2313 w2317 w2321 w2325 w2329 w2333 w2337 w2341 w2343 w2347 w2351 w2359]
          tunnel: [w2278 w2284 w2287 w2299 w2301 w2308 w2312 w2316 w2320 w2324 w2328 w2332 w2336 w2340 w2342 w2346 w2350 w2356] -> w2273
          frame "", Default {
          }
          frame "Exit" {
            n1282 = Enqueue Element(queue=w2281, element=CTL_Control_States."Save all settings", error in (no error)=w2283) -> (queue out=w2280:refnum<queue>, error out=w2282:errorcluster)  [unwired: 1 in, 1 out]
            n1283 = Enqueue Element(queue=w2280, element=CTL_Control_States."Close App", error in (no error)=w2282) -> (error out=w2284:errorcluster)  [unwired: 1 in, 2 out]
          }
          frame "Configure port(s)" {
            n1284 = Enqueue Element(queue=w2290, element=CTL_Control_States."Configure port(s)", error in (no error)=w2288) -> (error out=w2287:errorcluster)  [unwired: 1 in, 2 out]
          }
          frame "Timings calibration" {
            n1285 = Enqueue Element(queue=w2296, element=CTL_Control_States."Play Stop", error in (no error)=w2297) -> (queue out=w2294:refnum<queue>, error out=w2295:errorcluster)  [unwired: 1 in, 1 out]
            n1286 = Enqueue Element(queue=w2294, element=CTL_Control_States."Play Start", error in (no error)=w2295) -> (queue out=w2292:refnum<queue>, error out=w2293:errorcluster)  [unwired: 1 in, 1 out]
            n1287 = Enqueue Element(queue=w2292, element=CTL_Control_States."Timings calibration start", error in (no error)=w2293) -> (error out=w2299:errorcluster)  [unwired: 1 in, 2 out]
          }
          frame "Dispension rate calibration" {
            n1288 = Enqueue Element(queue=w2305, element=CTL_Control_States."Play Stop", error in (no error)=w2306) -> (queue out=w2303:refnum<queue>, error out=w2304:errorcluster)  [unwired: 1 in, 1 out]
            n1289 = Enqueue Element(queue=w2303, element=CTL_Control_States."Dispension calibration", error in (no error)=w2304) -> (error out=w2301:errorcluster)  [unwired: 1 in, 2 out]
          }
          frame "I/O Configuration" {
            n1290 = Enqueue Element(queue=w2311, element=CTL_Control_States."Set I/O config", error in (no error)=w2309) -> (error out=w2308:errorcluster)  [unwired: 1 in, 2 out]
          }
          frame "Cage and Recording" {
            n1291 = Enqueue Element(queue=w2315, element=CTL_Control_States."Cage and recording settings", error in (no error)=w2313) -> (error out=w2312:errorcluster)  [unwired: 1 in, 2 out]
          }
          frame "Play Start" {
            n1292 = Enqueue Element(queue=w2319, element=CTL_Control_States."Play Start", error in (no error)=w2317) -> (error out=w2316:errorcluster)  [unwired: 1 in, 2 out]
          }
          frame "Play Stop" {
            n1293 = Enqueue Element(queue=w2323, element=CTL_Control_States."Play Stop", error in (no error)=w2321) -> (error out=w2320:errorcluster)  [unwired: 1 in, 2 out]
          }
          frame "Start Recording" {
            n1294 = Enqueue Element(queue=w2327, element=CTL_Control_States."Start Recording", error in (no error)=w2325) -> (error out=w2324:errorcluster)  [unwired: 1 in, 2 out]
          }
          frame "Stop Recording" {
            n1295 = Enqueue Element(queue=w2331, element=CTL_Control_States."Stop Recording", error in (no error)=w2329) -> (error out=w2328:errorcluster)  [unwired: 1 in, 2 out]
          }
          frame "Start Over" {
            n1296 = Enqueue Element(queue=w2335, element=CTL_Control_States."Start over", error in (no error)=w2333) -> (error out=w2332:errorcluster)  [unwired: 1 in, 2 out]
          }
          frame "Fix broken track" {
            n1297 = Enqueue Element(queue=w2339, element=CTL_Control_States."Recalculate track with new settings", error in (no error)=w2337) -> (error out=w2336:errorcluster)  [unwired: 1 in, 2 out]
          }
          frame "Stream Data" {
            n1298 = call "Show Panel.vi"("error in (no error)"=w2341) -> ("error out"=w2340:errorcluster)  [unwired: 10 in]
          }
          frame "Save density maps" {
            n1299 = Enqueue Element(queue=w2345, element=CTL_Control_States."Save density map(s)", error in (no error)=w2343) -> (error out=w2342:errorcluster)  [unwired: 1 in, 2 out]
          }
          frame "Save Settings" {
            n1300 = Enqueue Element(queue=w2349, element=CTL_Control_States."Save all settings to custom location", error in (no error)=w2347) -> (error out=w2346:errorcluster)  [unwired: 1 in, 2 out]
          }
          frame "Load Settings" {
            n1301 = Enqueue Element(queue=w2353, element=CTL_Control_States."Load custom settings", error in (no error)=w2351) -> (error out=w2350:errorcluster)  [unwired: 1 in, 2 out]
          }
          frame "Open Manual" {
            n1302 = call <vilib>:"Application Directory.vi"() -> ("Application Directory"=w2354:path)
            n1303 = call "Get Abs Manual File Path.vi"("error in (no error)"=w2359, "Application directory"=w2354) -> ("error out"=w2358:errorcluster, "Manual file path"=w2355:path)
            n1304 = call-poly <userlib>:"File Exists__ogtk.vi"("file path"=w2355) -> ("exists"=w2357:bool)  [unwired: 6 in, 1 out]
            n1305 = case shown="False" w2357 {
              tunnel: w2358 -> [w2365 w2368]
              tunnel: [w2364 w2367] -> w2356
              tunnel: w2355 -> [w2363 w2366]
              frame False {
                n1306 = Path To String(path=w2363) -> (string=w2362:string)
                n1307 = Concatenate Strings("Help file not found: " ("string"), w2362) -> (w2361:string)
                n1308 = call "Display Message to User"("error in (no error)"=w2365, "Message"=w2361) -> ("error out"=w2364:errorcluster)  [unwired: 8 in, 1 out]
              }
              frame True {
                n1309 = call <vilib>:"Open a Document on Disk.vi"("error in (no error)"=w2368, "document path"=w2366) -> ("error out"=w2367:errorcluster)  [unwired: 5 in]
              }
            }
          }
        }
      }
      event "Check HW connection": Value Change {
        n1310 = event-data() -> ("CtlRef"=w2371:refnum<vi>, "OldVal"=w2372:bool)  [unwired: 1 in, 4 out]
        n1311 = Enqueue Element(queue=w2376, element=CTL_Control_States."HW Init", error in (no error)=w2369) -> (error out=w2374:errorcluster)  [unwired: 1 in, 2 out]
        n1312 = flat-sequence {
          tunnel: w2374 -> [w2377]
          tunnel: [w2377] -> w2373
          frame #0 {
            n1313 = Wait (ms)(milliseconds to wait=u32 500) -> ()  [unwired: 1 out]
          }
        }
        n1314 = property class="Bool (strict)"(reference=w2371, error in=w2373, "Value"=w2372) -> (error out=w2370:errorcluster)  [unwired: 1 out]
      }
      event "Set IO config": Value Change {
        n1315 = event-data() -> ("CtlRef"=w2381:refnum<vi>, "OldVal"=w2382:bool)  [unwired: 1 in, 4 out]
        n1316 = Enqueue Element(queue=w2386, element=CTL_Control_States."Set I/O config", error in (no error)=w2380) -> (error out=w2384:errorcluster)  [unwired: 1 in, 2 out]
        n1317 = flat-sequence {
          tunnel: w2384 -> [w2387]
          tunnel: [w2387] -> w2383
          frame #0 {
            n1318 = Wait (ms)(milliseconds to wait=u32 300) -> ()  [unwired: 1 out]
          }
        }
        n1319 = property class="Bool (strict)"(reference=w2381, error in=w2383, "Value"=w2382) -> (error out=w2379:errorcluster)  [unwired: 1 out]
      }
      event "Show zones", "Show magnets": Value Change {
        n1320 = event-data() -> ()  [unwired: 1 in, 6 out]
        n1321 = Enqueue Element(queue=w2392, element=CTL_Control_States."Zones layout update", error in (no error)=w2390) -> (error out=w2389:errorcluster)  [unwired: 1 in, 2 out]
      }
      event "Rainbow (time)": Value Change {
        w2394 = FALSE ("Rainbow (speed)")
        n1322 = event-data() -> ("NewVal"=w2395:bool)  [unwired: 1 in, 5 out]
        n1323 = Enqueue Element(queue=w2406, element=CTL_Control_States."Upd. trace length", error in (no error)=w2404) -> (error out=w2400:errorcluster)  [unwired: 1 in, 2 out]
        n1324 = Select(t=i64 53 ("Period"), s=w2395, f=i64 31 ("Period")) -> (s? t:f=w2403:i64)
        n1325 = local read "Show heatmap"() -> (w2393:bool)
        n1326 = local read "Show full track"() -> (w2398:bool)
        n1327 = property on="Rainbow (speed)" class="Bool (strict)"(error in=w2400, "Value"=w2394) -> (error out=w2399:errorcluster)  [unwired: 1 in, 1 out]
        n1328 = local write "UI update period"(w2403) -> ()
        n1329 = Build Array(w2395, w2394, w2398, w2393) -> (w2397:bool[])
        n1330 = Boolean Array To Number(Boolean array=w2397) -> (number=w2396:u32)
        n1331 = local write "Track show state"(w2396) -> ()
      }
      event "Rainbow (speed)": Value Change {
        w2408 = FALSE ("Rainbow (speed)")
        n1332 = event-data() -> ("NewVal"=w2409:bool)  [unwired: 1 in, 5 out]
        n1333 = Enqueue Element(queue=w2420, element=CTL_Control_States."Upd. trace length", error in (no error)=w2418) -> (error out=w2414:errorcluster)  [unwired: 1 in, 2 out]
        n1334 = Select(t=i64 53 ("Period"), s=w2409, f=i64 31 ("Period")) -> (s? t:f=w2417:i64)
        n1335 = local read "Show heatmap"() -> (w2407:bool)
        n1336 = local read "Show full track"() -> (w2412:bool)
        n1337 = property on="Rainbow (time)" class="Bool (strict)"(error in=w2414, "Value"=w2408) -> (error out=w2413:errorcluster)  [unwired: 1 in, 1 out]
        n1338 = local write "UI update period"(w2417) -> ()
        n1339 = Build Array(w2408, w2409, w2412, w2407) -> (w2411:bool[])
        n1340 = Boolean Array To Number(Boolean array=w2411) -> (number=w2410:u32)
        n1341 = local write "Track show state"(w2410) -> ()
      }
      event "Show heatmap": Value Change {
        n1342 = event-data() -> ("NewVal"=w2433:bool)  [unwired: 1 in, 5 out]
        n1343 = local read "Timeline"() -> (w2430:T37)
        n1344 = Unbundle By Name(w2430) -> ("Slider"=w2429:dbl, "Slider"=w2428:dbl)
        n1345 = First Call?() -> (First Call?: T/F=w2421:bool)
        n1346 = call <vilib>:"Value Has Changed PtByPt.vi"("input data point"=w2429, "initialize"=w2421) -> ("has changed"=w2426:bool)  [unwired: 1 out]
        n1347 = call <vilib>:"Value Has Changed PtByPt.vi"("input data point"=w2428, "initialize"=w2421) -> ("has changed"=w2425:bool)  [unwired: 1 out]
        n1348 = Compound Arithmetic op=OR(w2426, w2425) -> (w2427:bool)
        n1349 = case shown="True" w2433 {
          selector: w2433 -> [_ w2457]
          tunnel: w2431 -> [w2453 w2459]
          tunnel: [w2445 w2459] -> w2423
          tunnel: [w2451 w2456] -> w2432
          frame True {
            w2452 = FALSE ("Show full track")
            n1350 = local read "Rainbow (time)"() -> (w2449:bool)
            n1351 = local read "Rainbow (speed)"() -> (w2450:bool)
            n1352 = local read "Show heatmap"() -> (w2454:bool)
            n1353 = property on="Show full track" class="Bool (strict)"(error in=w2453, "Value"=w2452) -> (error out=w2446:errorcluster)  [unwired: 1 in, 1 out]
            n1354 = Select(t=w2449, s=w2450, f=TRUE) -> (s? t:f=w2447:bool)
            n1355 = property on="Rainbow (time)" class="Bool (strict)"(error in=w2446, "Value"=w2447) -> (error out=w2445:errorcluster)  [unwired: 1 in, 1 out]
            n1356 = Build Array(w2447, w2450, w2452, w2454) -> (w2455:bool[])
            n1357 = Boolean Array To Number(Boolean array=w2455) -> (number=w2451:u32)
          }
          frame False {
            n1358 = local read "Rainbow (time)"() -> (w2461:bool)
            n1359 = local read "Rainbow (speed)"() -> (w2460:bool)
            n1360 = local read "Show full track"() -> (w2458:bool)
            n1361 = Build Array(w2461, w2460, w2458, w2457) -> (w2462:bool[])
            n1362 = Boolean Array To Number(Boolean array=w2462) -> (number=w2456:u32)
          }
        }
        n1363 = case shown="True" w2427 {
          tunnel: w2424 -> [_ w2438]
          tunnel: w2423 -> [w2434 w2435]
          tunnel: [w2434 w2442] -> w2422
          frame False {
          }
          frame True {
            n1364 = Enqueue Element(queue=w2438, element=CTL_Control_States."Overlay tracks update", error in (no error)=w2435) -> (queue out=w2436:refnum<queue>, error out=w2439:errorcluster)  [unwired: 1 in, 1 out]
            n1365 = Enqueue Element(queue=w2436, element=CTL_Control_States."Location map update", error in (no error)=w2439) -> (queue out=w2441:refnum<queue>, error out=w2443:errorcluster)  [unwired: 1 in, 1 out]
            n1366 = Enqueue Element(queue=w2441, element=CTL_Control_States."Speed map update", error in (no error)=w2443) -> (error out=w2442:errorcluster)  [unwired: 1 in, 2 out]
          }
        }
        n1367 = local write "Track show state"(w2432) -> ()
      }
      event "Show full track": Value Change {
        n1368 = event-data() -> ("NewVal"=w2466:bool)  [unwired: 1 in, 5 out]
        n1369 = case shown="False" w2466 {
          tunnel: w2464 -> [w2469 w2476]
          tunnel: [w2471 w2478] -> w2465
          tunnel: [w2467 w2476] -> w2463
          frame True {
            w2468 = FALSE ("Show full track")
            n1370 = local read "Rainbow (time)"() -> (w2473:bool)
            n1371 = local read "Rainbow (speed)"() -> (w2472:bool)
            n1372 = local read "Show full track"() -> (w2470:bool)
            n1373 = property on="Show heatmap" class="Bool (strict)"(error in=w2469, "Value"=w2468) -> (error out=w2467:errorcluster)  [unwired: 1 in, 1 out]
            n1374 = Build Array(w2473, w2472, w2470, w2468) -> (w2474:bool[])
            n1375 = Boolean Array To Number(Boolean array=w2474) -> (number=w2471:u32)
          }
          frame False {
            n1376 = local read "Rainbow (time)"() -> (w2480:bool)
            n1377 = local read "Rainbow (speed)"() -> (w2479:bool)
            n1378 = local read "Show full track"() -> (w2477:bool)
            n1379 = local read "Show heatmap"() -> (w2475:bool)
            n1380 = Build Array(w2480, w2479, w2477, w2475) -> (w2481:bool[])
            n1381 = Boolean Array To Number(Boolean array=w2481) -> (number=w2478:u32)
          }
        }
        n1382 = local write "Track show state"(w2465) -> ()
      }
      event "Timeline": Mouse Up {
        n1383 = event-data() -> ()  [unwired: 1 in, 8 out]
        n1384 = local read "Timeline"() -> (w2494:T37)
        n1385 = Unbundle By Name(w2494) -> ("Slider"=w2493:dbl, "Slider"=w2492:dbl, "Slider"=w2489:dbl)
        n1386 = First Call?() -> (First Call?: T/F=w2487:bool)
        n1387 = local read "Play/Pause"() -> (w2495:bool)
        n1388 = Not(x=w2495) -> (.not. x?=w2488:bool)
        n1389 = call <vilib>:"Value Has Changed PtByPt.vi"("input data point"=w2489, "initialize"=w2487) -> ("has changed"=w2486:bool)  [unwired: 1 out]
        n1390 = call <vilib>:"Value Has Changed PtByPt.vi"("input data point"=w2493, "initialize"=w2487) -> ("has changed"=w2485:bool)  [unwired: 1 out]
        n1391 = call <vilib>:"Value Has Changed PtByPt.vi"("input data point"=w2492, "initialize"=w2487) -> ("has changed"=w2484:bool)  [unwired: 1 out]
        n1392 = Compound Arithmetic op=OR(w2485, w2484, w2486) -> (w2490:bool)
        n1393 = And(x=w2488, y=w2490) -> (x .and. y?=w2491:bool)
        n1394 = Or(x=w2485, y=w2484) -> (x .or. y?=w2483:bool)
        n1395 = case shown="True" w2491 {
          tunnel: w2497 -> [w2498 w2505]
          tunnel: w2496 -> [w2499 w2506]
          tunnel: [w2499 w2503] -> w2482
          tunnel: [w2498 w2502] -> _
          tunnel: w2483 -> [_ w2504]
          frame False {
          }
          frame True {
            n1396 = Enqueue Element(queue=w2505, element=CTL_Control_States."Timeline update", error in (no error)=w2506) -> (queue out=w2501:refnum<queue>, error out=w2500:errorcluster)  [unwired: 1 in, 1 out]
            n1397 = case shown="True" w2504 {
              tunnel: [w2509 w2516] -> w2503
              tunnel: [w2508 w2515] -> w2502
              tunnel: w2501 -> [w2508 w2513]
              tunnel: w2500 -> [w2509 w2512]
              frame False {
              }
              frame True {
                n1398 = Enqueue Element(queue=w2513, element=CTL_Control_States."Overlay tracks update", error in (no error)=w2512) -> (queue out=w2511:refnum<queue>, error out=w2510:errorcluster)  [unwired: 1 in, 1 out]
                n1399 = Enqueue Element(queue=w2511, element=CTL_Control_States."Location map update", error in (no error)=w2510) -> (queue out=w2519:refnum<queue>, error out=w2518:errorcluster)  [unwired: 1 in, 1 out]
                n1400 = Enqueue Element(queue=w2519, element=CTL_Control_States."Speed map update", error in (no error)=w2518) -> (queue out=w2515:refnum<queue>, error out=w2516:errorcluster)  [unwired: 1 in, 1 out]
              }
            }
          }
        }
      }
      event "Add Reward": Value Change {
        n1401 = event-data() -> ("OldVal"=w2525:bool)  [unwired: 1 in, 5 out]
        n1402 = local write "Add Reward"(w2525) -> ()
        n1403 = Enqueue Element(queue=w2522, element=CTL_Control_States."Add Reward condition", error in (no error)=w2524) -> (error out=w2523:errorcluster)  [unwired: 1 in, 2 out]
      }
      event "Modify Reward": Value Change {
        n1404 = event-data() -> ("OldVal"=w2530:bool)  [unwired: 1 in, 5 out]
        n1405 = local write "Modify Reward"(w2530) -> ()
        n1406 = Enqueue Element(queue=w2527, element=CTL_Control_States."Modify Reward condition", error in (no error)=w2529) -> (error out=w2528:errorcluster)  [unwired: 1 in, 2 out]
      }
      event "Remove Reward": Value Change {
        n1407 = event-data() -> ("OldVal"=w2535:bool)  [unwired: 1 in, 5 out]
        n1408 = local write "Remove Reward"(w2535) -> ()
        n1409 = Enqueue Element(queue=w2532, element=CTL_Control_States."Delete Reward condition", error in (no error)=w2534) -> (error out=w2533:errorcluster)  [unwired: 1 in, 2 out]
      }
      event "Reward and stimulation": Value Change; "Reward and stimulation": Double Click; "Reward and stimulation": Mouse Down {
        n1410 = event-data() -> ()  [unwired: 1 in, 4 out]
        n1411 = Enqueue Element(queue=w2537, element=CTL_Control_States."Check Reward condition(s)", error in (no error)=w2539) -> (error out=w2538:errorcluster)  [unwired: 1 in, 2 out]
      }
      event "Diagram (display)": Mouse Up {
        n1412 = event-data() -> ()  [unwired: 1 in, 8 out]
        n1413 = property on="Diagram (display)" class="ImageControl"(error in=w2548) -> (error out=w2541:errorcluster, "ROI"=w2547:T29)  [unwired: 1 in, 1 out]
        n1414 = local write "ROIs"(w2547) -> ()
        n1415 = Unbundle By Name(w2547) -> ("Contours"=w2546:T93)
        n1416 = for {
          tunnel: w2546 -> [w2556] mode=indexing
          tunnel: [w2553] -> w2544 mode=indexing
          tunnel: [w2549] -> w2545 mode=indexing
          i -> [w2555]
          n1417 = Unbundle By Name(w2556) -> ("ROI Type"=w2550:u32)
          n1418 = Increment(x=w2555) -> (x+1=w2554:i32)
          n1419 = case shown="0, Default" w2550 {
            tunnel: ["Unknown" "Rect" "Rot. rect" "Polygon" "Freehand" "Oval" "Annulus"] -> w2549
            frame 0, Default {
            }
            frame 3 {
            }
            frame 12 {
            }
            frame 5 {
            }
            frame 6 {
            }
            frame 4 {
            }
            frame 7 {
            }
          }
          n1420 = Format Value(string ("")="ROI #" ("string"), format string="%02u", value (0)=w2554) -> (output string=w2553:string)
        }
        n1421 = Build Array(w2545) -> (w2543:string[][])
        n1422 = Transpose 2D Array(2D array=w2543) -> (transposed array=w2542:string[][])
        n1423 = property on="ROIs list" class="MCListbox (strict)"(error in=w2541, "ItemNames"=w2542, "RowHdrs[]"=w2544) -> (error out=w2540:errorcluster)  [unwired: 1 in, 1 out]
      }
      event "Multiplyer of chart RX": Value Change {
        n1424 = event-data() -> ("NewVal"=w2564:u8)  [unwired: 1 in, 5 out]
        n1425 = property on="Mouse speed" class="WFChart (strict)"(error in=w2571) -> (error out=w2565:errorcluster, "XScale.Minimum"=w2568:dbl)  [unwired: 1 in, 1 out]
        n1426 = Scale By Power Of 2(n=w2564, x=10) -> (x*2^n=w2567:i32)
        n1427 = Add(x=w2568, y=w2567) -> (x+y=w2566:dbl)
        n1428 = property on="Mouse speed" class="WFChart (strict)"(error in=w2565, "XScale.Maximum"=w2566) -> (error out=w2570:errorcluster)  [unwired: 1 in, 1 out]
      }
      event Value Change {
        n1429 = event-data() -> ("NewVal"=w2573:T14)  [unwired: 1 in, 5 out]
        n1430 = local read "Settings cluster (local)"() -> (w2575:T16)
        n1431 = call "SW_Update_radial_segmentation_variable_info.vi"("error in (no error)"=w2576, "NewVal"=w2573, "Settings cluster (local) in"=w2575) -> ("error out"=w2572:errorcluster, "Settings cluster (local) out"=w2574:T16)  [unwired: 1 in]
        n1432 = Enqueue Element(queue=w2580, element=CTL_Control_States."Zones layout update", error in (no error)=w2572) -> (error out=w2578:errorcluster)  [unwired: 1 in, 2 out]
        n1433 = local write "Settings cluster (local)"(w2574) -> ()
        n1434 = call "100 ms"("error in (no error)"=w2578) -> ("error out"=w2577:errorcluster)  [unwired: 10 in]
      }
      event User Event {
        n1435 = event-data() -> ("Active rules"=w2583:bool[])  [unwired: 1 in, 4 out]
        n1436 = Array To Cluster(array=w2583) -> (cluster=w2582:T94)
        n1437 = local write "Active rules"(w2582) -> ()
      }
      event "Play/Pause": Value Change {
        n1438 = event-data() -> ("NewVal"=w2590:bool)  [unwired: 1 in, 5 out]
        n1439 = Get Notifier Status(notifier=w2588, error in (no error)=w2587) -> (current notification=w2585:T46, error out=w2586:errorcluster)  [unwired: 3 out]
        n1440 = Unbundle By Name(w2585) -> ("Offline mode"=w2584:bool)
        n1441 = case shown="False" w2584 {
          tunnel: w2591 -> [w2595 w2607]
          tunnel: w2590 -> [w2594 w2606]
          tunnel: w2586 -> [w2593 w2605]
          tunnel: [w2592 w2604] -> w2589
          frame True {
            # "Offline mode"
            n1442 = case shown="True" w2594 {
              tunnel: w2595 -> [w2598 w2603]
              tunnel: w2593 -> [w2597 w2601]
              tunnel: [w2596 w2600] -> w2592
              frame True {
                # "Play Start"
                n1443 = Enqueue Element(queue=w2598, element=CTL_Control_States."Play Start", error in (no error)=w2597) -> (error out=w2596:errorcluster)  [unwired: 1 in, 2 out]
              }
              frame False {
                # "Play Stop"
                n1444 = Enqueue Element(queue=w2603, element=CTL_Control_States."Play Stop", error in (no error)=w2601) -> (error out=w2600:errorcluster)  [unwired: 1 in, 2 out]
              }
            }
          }
          frame False {
            # "Online mode"
            n1445 = case shown="True" w2606 {
              tunnel: w2607 -> [w2608 w2618]
              tunnel: w2605 -> [w2613 w2616]
              tunnel: [w2610 w2615] -> w2604
              frame True {
                # "Play Start"
                n1446 = call <vilib>:"Set Busy.vi"("error in (no error)"=w2613) -> ("error out"=w2612:errorcluster)  [unwired: 9 in, 1 out]
                n1447 = Enqueue Element(queue=w2608, element=CTL_Control_States."Play Start", error in (no error)=w2612) -> (error out=w2611:errorcluster)  [unwired: 1 in, 2 out]
                n1448 = call "1.5s delay"("error in (no error)"=w2611) -> ("error out"=w2609:errorcluster)  [unwired: 10 in]
                n1449 = call <vilib>:"Unset Busy.vi"("error in (no error)"=w2609) -> ("error out"=w2610:errorcluster)  [unwired: 10 in]
              }
              frame False {
                # "Play Stop"
                n1450 = Enqueue Element(queue=w2618, element=CTL_Control_States."Play Stop", error in (no error)=w2616) -> (error out=w2615:errorcluster)  [unwired: 1 in, 2 out]
              }
            }
          }
        }
      }
      event "Start over": Value Change {
        n1451 = event-data() -> ("NewVal"=w2625:bool)  [unwired: 1 in, 5 out]
        n1452 = Get Notifier Status(notifier=w2623, error in (no error)=w2622) -> (current notification=w2620:T46, error out=w2621:errorcluster)  [unwired: 3 out]
        n1453 = Unbundle By Name(w2620) -> ("Offline mode"=w2619:bool)
        n1454 = case shown="True" w2619 {
          tunnel: w2626 -> [w2630 _]
          tunnel: w2625 -> [w2629 _]
          tunnel: w2621 -> [w2628 w2639]
          tunnel: [w2627 w2639] -> w2624
          frame True {
            # "Offline mode"
            n1455 = case shown="True" w2629 {
              tunnel: w2630 -> [w2633 w2638]
              tunnel: w2628 -> [w2632 w2636]
              tunnel: [w2631 w2635] -> w2627
              frame True {
                # "Play Start"
                n1456 = Enqueue Element(queue=w2633, element=CTL_Control_States."Start over", error in (no error)=w2632) -> (error out=w2631:errorcluster)  [unwired: 1 in, 2 out]
              }
              frame False {
                # "Play Stop"
                n1457 = Enqueue Element(queue=w2638, element=CTL_Control_States."Play Stop", error in (no error)=w2636) -> (error out=w2635:errorcluster)  [unwired: 1 in, 2 out]
              }
            }
          }
          frame False {
            # "Online mode"
          }
        }
      }
      event "Record/Stop": Value Change {
        n1458 = event-data() -> ("NewVal"=w2642:bool)  [unwired: 1 in, 5 out]
        n1459 = case shown="False" w2642 {
          tunnel: w2643 -> [w2646 w2651]
          tunnel: w2641 -> [w2645 w2649]
          tunnel: [w2644 w2648] -> w2640
          frame True {
            # "Record Start"
            n1460 = Enqueue Element(queue=w2646, element=CTL_Control_States."Start Recording", error in (no error)=w2645) -> (error out=w2644:errorcluster)  [unwired: 1 in, 2 out]
          }
          frame False {
            # "Recording Stop"
            n1461 = Enqueue Element(queue=w2651, element=CTL_Control_States."Stop Recording", error in (no error)=w2649) -> (error out=w2648:errorcluster)  [unwired: 1 in, 2 out]
          }
        }
      }
      event "Trace, s": Value Change {
        n1462 = event-data() -> ()  [unwired: 1 in, 6 out]
        n1463 = Enqueue Element(queue=w2655, element=CTL_Control_States."Upd. trace length", error in (no error)=w2653) -> (error out=w2652:errorcluster)  [unwired: 1 in, 2 out]
      }
      event "Open File": Value Change {
        n1464 = event-data() -> ("OldVal"=w2660:bool)  [unwired: 1 in, 5 out]
        n1465 = local write "Open File"(w2660) -> ()
        n1466 = Enqueue Element(queue=w2657, element=CTL_Control_States."Load recorded data", error in (no error)=w2656) -> (error out=w2659:errorcluster)  [unwired: 1 in, 2 out]
      }
      event "Reset barplot": Value Change {
        n1467 = event-data() -> ("OldVal"=w2661:bool)  [unwired: 1 in, 5 out]
        n1468 = flat-sequence {
          tunnel: [w2665] -> w2662
          tunnel: w2661 -> [w2665]
          frame #0 {
            n1469 = Wait (ms)(milliseconds to wait=u32 10) -> ()  [unwired: 1 out]
          }
        }
        n1470 = local write "Reset barplot"(w2662) -> ()
      }
      event Value Change {
        n1471 = event-data() -> ("NewVal"=w2670:T38)  [unwired: 1 in, 5 out]
        n1472 = To Unsigned Byte Integer(number=w2670) -> (unsigned 8bit integer=w2671:u8)
        n1473 = Build Array(w2671) -> (w2669:u8[])
        n1474 = flat-sequence {
          tunnel: w2669 -> [w2672]
          tunnel: w2668 -> [w2676]
          tunnel: w2667 -> [w2675]
          tunnel: [w2674] -> w2666
          frame #0 {
            n1475 = global write "SW_Globals_2.2+.vi" "Regions to mark selected"(w2672) -> ()
          }
          frame #1 {
            n1476 = Wait (ms)(milliseconds to wait=u32 50) -> ()  [unwired: 1 out]
          }
          frame #2 {
            n1477 = Enqueue Element(queue=w2676, element=CTL_Control_States."Zones layout update", error in (no error)=w2675) -> (error out=w2674:errorcluster)  [unwired: 1 in, 2 out]
          }
        }
      }
      event "Speed threshold": Value Change {
        n1478 = event-data() -> ()  [unwired: 1 in, 6 out]
        n1479 = Enqueue Element(queue=w2684, element=CTL_Control_States."Zones layout update", error in (no error)=w2683) -> (queue out=w2679:refnum<queue>, error out=w2681:errorcluster)  [unwired: 1 in, 1 out]
        n1480 = Enqueue Element(queue=w2679, element=CTL_Control_States."Overlay tracks update", error in (no error)=w2681) -> (error out=w2680:errorcluster)  [unwired: 1 in, 2 out]
      }
      event Key Down {
        n1481 = event-data() -> ("VKey"=w2687:T95, "ScanCode"=w2688:i16)  [unwired: 1 in, 8 out]
        n1482 = case shown="72, 75, 77, 80" w2688 {
          tunnel: w2687 -> [_ w2693]
          tunnel: w2686 -> [w2689 w2692]
          tunnel: [w2689 w2691] -> w2685
          frame Default {
          }
          frame 72, 75, 77, 80 {
            n1483 = Format Into String(format string="%s", error in=w2692, w2693) -> (resulting string=w2690:string, error out=w2691:errorcluster)  [unwired: 1 in]
            n1484 = local write "Key_pressed"(w2690) -> ()
          }
        }
      }
      event Key Up {
        n1485 = event-data() -> ("ScanCode"=w2695:i16, "Mods"=w2698:cluster{"Num Pad":bool, "Menu Key":bool})  [unwired: 1 in, 5 out]
        n1486 = case shown="72, 75, 77, 80" w2695 {
          tunnel: w2698 -> [_ _]
          tunnel: w2697 -> [w2699 w2701]
          tunnel: [w2699 w2701] -> w2696
          frame Default {
          }
          frame 72, 75, 77, 80 {
            n1487 = local write "Key_pressed"("----" ("Key_pressed")) -> ()
          }
        }
      }
    }
    n1488 = call <vilib>:"Simple Error Handler.vi"("error in (no error)"=w2256) -> ("error out"=w2258:errorcluster)  [unwired: 4 in, 4 out]
    n1489 = node-c288(w2258) -> ()  [unwired: 1 out]
  }
  n1490 = node-c288(w42) -> (w3:errorcluster)
  n1491 = node-c288(w34) -> (w30:errorcluster)
  n1492 = node-c288(w64) -> (w46:errorcluster)
  n1493 = node-c288(w53) -> (w29:errorcluster)
  n1494 = node-c288(w59) -> (w47:errorcluster)
  n1495 = node-c288(w71) -> (w48:errorcluster)
  n1496 = Flush Queue(queue=w67, error in (no error)=w48) -> (queue out=w66:refnum<queue>, error out=w49:errorcluster)  [unwired: 1 out]
  n1497 = Merge Errors(w29, w30, w3) -> (w38:errorcluster)
  n1498 = Release Queue(queue=w66, error in (no error)=w49) -> (error out=w45:errorcluster)  [unwired: 1 in, 2 out]
  n1499 = Merge Errors(w45, w46, w47, w38) -> (w11:errorcluster)
  n1500 = Unregister For Events(event registration refnum=w12, error in=w11) -> (error out=w10:errorcluster)
  n1501 = Release Notifier(notifier=w44, error in (no error)=w10) -> (error out=w21:errorcluster)  [unwired: 1 in, 2 out]
  n1502 = call <vilib>:"Clear Timing Source.vi"("error in (no error)"=w21, "name"=w19) -> ("error out"=→"error out":errorcluster)  [unwired: 8 in, 1 out]
